vi "TCE.vi"() -> (11 "placeholder image":T1(plugin-control))   [LabVIEW 2024]
uses:
  DataCluster_TCAL.ctl
  <vilib>/vision/Image Controls.llb/IMAQ Image.ctl
  TCE_Config.ctl
  <vilib>/Utility/file.llb/Read Delimited Spreadsheet (string).vi
  <vilib>/Utility/file.llb/Write Delimited Spreadsheet (string).vi
  <vilib>/Utility/file.llb/Write Delimited Spreadsheet (DBL).vi
  <vilib>/Analysis/NI_AALBase.lvlib
panel:
  out "FreezeFract Concatinated":dbl[](array[numeric])
  in  "Correct Data":bool
  out "Offset Applied?":bool
  out "recentPaths":path[](array[path])=[path "D:/OneDrive/OneDrive - Aarhus Universitet/Data/D20_4/Result Data.csv"]
  out "version":string="version 0.0.0.1" caption="Version"
  out "Title":string="Thermal Camera Evaluation" caption="Version"
  in  "Remove_Correction":bool
  out "Offsets":dbl[](array[numeric])
  in  "Calc_All":bool
  in  "Well":i32=251
  in  "ImageIdx":u32(slide)=98 scale=0.0..527.0
  in  "Path":path
  out "MeltTemps":dbl[](array[numeric])=[-5.408275862068933, -5.766551724137912, -5.134827586206882, -4.684827586206836, -7.485172413793066, -5.2834482758620425, -5.345517241379298, -6.320689655172373, -3.992413793103424, -3.7082758620689447, -3.4782758620689265, -5.388275862068895, -5.597241379310333, -4.740689655172389, -4.031034482758571, -4.187241379310308, -6.245172413793114, -4.773793103448213, -4.427586206896535, -3.742413793103424, -4.568965517241338, -5.621379310344764, -4.7503448275861615, -5.029999999999973, -5.895517241379309, -4.551379310344771, -4.0196551724137635, -4.698965517241334, -4.126551724137926, -2.993448275862022, -4.383448275862065, -4.888965517241331, -5.901724137931012, -8.037586206896549, -3.918275862068924, -4.438620689655181, -5.749655172413782, -4.38241379310341, -4.932758620689583, -4.997586206896528, -4.125862068965489, -3.4279310344827536, -5.144482758620654, -2.891379310344803, -2.92999999999995, -3.1620689655172214, -3.216206896551739, -4.3248275862068795, -1.3320689655172373, -2.026551724137903, 0.5675862068965785, -0.5103448275861524, 0.4782758620689833, -1.9634482758620493, -0.1275862068965239, -0.1651724137930728, -0.9937931034482403, -0.6210344827586027, 0.2934482758620902, 0.6917241379310894, 1.3537931034483108, -1.852758620689599, -1.3782758620689037, 1.2606896551724844, -0.0275862068965012, -2.2548275862068294, -1.0710344827585914, -1.4565517241379098, -0.7220689655172237, -0.853793103448254, -0.2686206896551653, -0.5562068965517142, 0.0324137931034443, -0.2768965517241213, 1.1982758620689538, 1.2775862068966148, -0.6427586206896194, 0.5986206896552062, -0.3313793103448006, -0.6034482758620356, -2.0755172413792593, -2.182758620689583, -1.6548275862068635, -0.7234482758620402, -0.6872413793103078, -0.9086206896551516, -0.5427586206895967, -0.0527586206895876, 1.211379310344853, 0.2365517241379393, -0.526551724137903, -0.1537931034482085, 1.1865517241379848, 0.7089655172413813, -1.8837931034482267, 0.5872413793103988, -2.0686206896551766, -2.519310344827545, -2.2079310344827263, -2.2441379310344587, -2.0355172413792957, -2.3782758620689037, -2.0879310344827218, -1.998965517241345, -2.0948275862068613, -2.1227586206896376, -2.195517241379264, -1.969655172413752, -2.0175862068965102, -2.061724137931037, -2.028275862068938, -1.7403448275861706, -2.1765517241378802, -2.432758620689583, -2.186551724137928, -2.063448275862015, -2.331724137931019, -2.1351724137931, -2.0499999999999545, -2.1537931034482085, -2.235172413793066, -2.213793103448211, -2.082758620689617, -2.1703448275861774, -2.0434482758620334, -2.173448275862029, -1.9048275862068635, -1.683793103448238, -1.8931034482758378, -2.165172413793073, -2.068965517241338, -2.1862068965517096, -2.161034482758623, -2.085517241379307, -2.0631034482758537, -2.134137931034445, -2.104827586206852, -2.1775862068965353, -2.2255172413792934, -2.161724137931003, -2.0251724137930864, -2.0106896551724276, -2.211379310344796, -1.9093103448275315, -2.3158620689654867, -1.9827586206895944, -2.258275862068899, -2.2927586206895967, -2.0868965517241236, -2.0810344827585823, -2.17931034482757, -2.134137931034445, -2.151379310344794, -2.101034482758621, -2.2465517241379303, -2.339999999999975, -2.061379310344819, -2.082413793103399, -2.220689655172407, -2.0658620689654867, -2.1337931034482267, -2.0158620689654754, -2.1179310344827513, -2.1999999999999886, -2.130344827586157, -2.0489655172413563, -2.0534482758620243, -2.0851724137930887, -2.1079310344827036, -2.0241379310344882, -2.0693103448275565, -2.1348275862068817, -2.1431034482758378, -2.0268965517241213, -2.0317241379310076, -1.6172413793103146, -2.02103448275858, -2.331724137931019, -2.4068965517241168, -2.2337931034482494, -2.383103448275847, -2.1417241379310212, -2.1768965517240986, -2.2579310344827377, -2.1786206896551334, -2.032068965517226, -2.1162068965517165, -2.2706896551724185, -1.9220689655172123, -2.174482758620684, -2.11206896551721, -2.0858620689654686, -0.1458620689654708, -0.1541379310344837, -0.0103448275861524, -0.2106896551724162, -0.2299999999999613, -0.243448275862022, -0.2624137931034056, -0.2906896551724003, -0.3306896551724208, -0.3089655172413472, -0.2099999999999795, -0.276551724137903, -0.15896551724137, -0.0637931034482335, -0.2572413793103578, 0.1706896551724526, -0.0779310344827309, -0.0958620689654595, 0.0658620689655436, -0.1041379310344723, -0.4631034482758308, -0.1158620689654981, -0.1268965517240872, -0.3313793103448006, -0.2803448275861911, -0.1562068965517369, -0.06793103448274, -0.131379310344812, -0.0282758620689378, 0.0079310344827945, 0.0748275862069363, 0.2665517241379689, 0.0537931034482995, -0.2062068965516914, -0.1179310344827513, -0.3424137931033897, -0.0275862068965012, -0.2003448275861501, -0.1096551724137953, -0.0944827586206429, -0.4137931034482563, -0.5093103448275542, 0.0627586206896922, -0.1789655172413518, -0.0096551724137726, 0.0068965517241395, -0.0334482758620425, 0.2120689655172896, -0.1099999999999568, -0.2282758620689265, -0.1213793103447642, -0.1482758620689424, -0.2106896551724162, -0.0927586206896081, -0.1093103448275201, -0.076206896551696, -0.1593103448275315, -0.0886206896551585, -0.1924137931034124, -0.0558620689654958, -0.0313793103447892, -0.0799999999999841, -0.1262068965517074, 0.2117241379310713, -0.1141379310344632, -0.1796551724137885, -0.2003448275861501, -0.0327586206896058, 0.0655172413793252, -0.1886206896551812, -0.0327586206896058, -0.1424137931034011, -0.2406896551723889, -0.034827586206859, -0.1527586206896103, -0.1848275862068363, -0.0313793103447892, -0.0158620689654754, -0.0372413793103306, 0.2079310344827832, -0.2451724137931137, -0.6586206896551516, -0.0858620689654686, -0.2462068965517119, -0.2631034482758423, -0.0217241379310167, -0.2486206896551266, 0.0455172413793434, -0.2441379310344587, -0.1786206896551334, -0.230689655172398, -0.0131034482758423, -0.2613793103448074, -0.4093103448275315, -0.0124137931034056, 0.1572413793103919, 0.0, 0.0, 0.0, 1.7110344827586346, 1.5944827586206998, 1.9227586206896488, 0.1648275862069113, 1.3268965517241327, 0.0, 0.0, 0.0, 1.441379310344871, 0.8996551724138158, 2.017586206896567, 1.1068965517241622, 2.3413793103448484, 1.119655172413843, 1.9251724137931205, 1.484482758620743, 1.7410344827586641, 1.624137931034511, 1.9227586206896488, 1.88793103448279, 1.3758620689655459, -0.8037931034482426, 1.6562068965517938, 1.90758620689661, 2.0327586206896626, 1.5831034482758923, 2.1006896551724594, 2.216206896551796, 2.153448275862104, 1.9158620689655093, 2.1862068965517665, 1.9189655172414175, 2.0968965517241713, 1.4434482758620675, 1.914482758620693, 1.868620689655188, 1.9841379310345246, 2.0734482758621198, 1.9231034482759242, 1.7982758620689765, 1.852068965517276, 2.086551724137962, 2.055172413793173, 1.9510344827586437, 2.1220689655172578, 2.108620689655197, 2.3431034482758832, 0.0, 1.7272413793103851, 2.039655172413859, 1.9255172413793389, 2.2200000000000273, 1.5868965517241804, 1.914482758620693, 1.9610344827586343, 2.145517241379366, 1.9279310344828102, 1.8203448275862115, 2.199310344827609, 2.312413793103474, 2.407931034482772, 2.4206896551724526, 1.8224137931034647, 2.3637931034483017, 1.6882758620689629, 1.8193103448276133, 1.7324137931034898, 2.3037931034482995, 1.794137931034527, 2.011034482758646, 2.0013793103448734, 1.7558620689655413, 1.8893103448276065, 2.1520689655172873, 1.9962068965517685, 2.3103448275862206, 2.1217241379310963, 1.863103448275922, 1.9231034482759242, 1.5434482758620902, 1.6648275862069113, 1.8944827586207111, 1.63793103448279, 1.8379310344827786, 1.948620689655229, 2.157241379310392, 1.835517241379364, 1.950344827586207, 2.018275862069004, 1.9565517241379666, 1.7651724137931524, 2.068965517241395, 2.168275862068981]
  out "FreezeArray":bool[](array[boolean])=[TRUE, TRUE, TRUE, TRUE, TRUE, TRUE, TRUE, TRUE, TRUE, TRUE, TRUE, TRUE, TRUE, TRUE, TRUE, TRUE, TRUE, TRUE, TRUE, TRUE, TRUE, TRUE, TRUE, TRUE, TRUE, TRUE, TRUE, TRUE, TRUE, TRUE, TRUE, TRUE, TRUE, TRUE, TRUE, TRUE, TRUE, TRUE, TRUE, TRUE, TRUE, TRUE, TRUE, TRUE, TRUE, TRUE, TRUE, TRUE, TRUE, TRUE, TRUE, TRUE, TRUE, TRUE, TRUE, TRUE, TRUE, TRUE, TRUE, TRUE, TRUE, TRUE, TRUE, TRUE, TRUE, TRUE, TRUE, TRUE, TRUE, TRUE, TRUE, TRUE, TRUE, TRUE, TRUE, TRUE, TRUE, TRUE, TRUE, TRUE, TRUE, TRUE, TRUE, TRUE, TRUE, TRUE, TRUE, TRUE, TRUE, TRUE, TRUE, TRUE, TRUE, TRUE, TRUE, TRUE, TRUE, TRUE, TRUE, TRUE, TRUE, TRUE, TRUE, TRUE, TRUE, TRUE, TRUE, TRUE, TRUE, TRUE, TRUE, TRUE, TRUE, TRUE, TRUE, TRUE, TRUE, TRUE, TRUE, TRUE, TRUE, TRUE, TRUE, TRUE, TRUE, TRUE, TRUE, TRUE, TRUE, TRUE, TRUE, TRUE, TRUE, TRUE, TRUE, TRUE, TRUE, TRUE, TRUE, TRUE, TRUE, TRUE, TRUE, TRUE, TRUE, TRUE, TRUE, TRUE, TRUE, TRUE, TRUE, TRUE, TRUE, TRUE, TRUE, TRUE, TRUE, TRUE, TRUE, TRUE, TRUE, TRUE, TRUE, TRUE, TRUE, TRUE, TRUE, TRUE, TRUE, TRUE, TRUE, TRUE, TRUE, TRUE, TRUE, TRUE, TRUE, TRUE, TRUE, TRUE, TRUE, TRUE, TRUE, TRUE, TRUE, TRUE, TRUE, TRUE, TRUE, TRUE, TRUE, TRUE, TRUE, TRUE, TRUE, TRUE, TRUE, TRUE, TRUE, TRUE, TRUE, TRUE, TRUE, TRUE, TRUE, TRUE, TRUE, TRUE, TRUE, TRUE, TRUE, TRUE, TRUE, TRUE, TRUE, TRUE, TRUE, TRUE, TRUE, TRUE, TRUE, TRUE, TRUE, TRUE, TRUE, TRUE, TRUE, TRUE, TRUE, TRUE, TRUE, TRUE, TRUE, TRUE, TRUE, TRUE, TRUE, TRUE, TRUE, TRUE, TRUE, TRUE, TRUE, TRUE, TRUE, TRUE, TRUE, TRUE, TRUE, TRUE, TRUE, TRUE, TRUE, TRUE, TRUE, TRUE, TRUE, TRUE, TRUE, TRUE, TRUE, TRUE, TRUE, TRUE, TRUE, TRUE, TRUE, TRUE, TRUE, TRUE, TRUE, TRUE, TRUE, TRUE, TRUE, TRUE, TRUE, TRUE, TRUE, TRUE, TRUE, TRUE, TRUE, TRUE, TRUE, TRUE, TRUE, TRUE, FALSE, FALSE, FALSE, TRUE, TRUE, TRUE, TRUE, TRUE, FALSE, FALSE, FALSE, TRUE, TRUE, TRUE, TRUE, TRUE, TRUE, TRUE, TRUE, TRUE, TRUE, TRUE, TRUE, TRUE, TRUE, TRUE, TRUE, TRUE, TRUE, TRUE, TRUE, TRUE, TRUE, TRUE, TRUE, TRUE, TRUE, TRUE, TRUE, TRUE, TRUE, TRUE, TRUE, TRUE, TRUE, TRUE, TRUE, TRUE, TRUE, TRUE, FALSE, TRUE, TRUE, TRUE, TRUE, TRUE, TRUE, TRUE, TRUE, TRUE, TRUE, TRUE, TRUE, TRUE, TRUE, TRUE, TRUE, TRUE, TRUE, TRUE, TRUE, TRUE, TRUE, TRUE, TRUE, TRUE, TRUE, TRUE, TRUE, TRUE, TRUE, TRUE, TRUE, TRUE, TRUE, TRUE, TRUE, TRUE, TRUE, TRUE, TRUE, TRUE, TRUE, TRUE, TRUE, TRUE]
  out "ThermTemps":dbl[](array[numeric])
  out "PartitionArray":string[](array[string])=["A, MQ unfiltered", "A, MQ unfiltered", "A, MQ unfiltered", "A, MQ unfiltered", "A, MQ unfiltered", "A, MQ unfiltered", "A, MQ unfiltered", "A, MQ unfiltered", "A, MQ unfiltered", "A, MQ unfiltered", "A, MQ unfiltered", "A, MQ unfiltered", "A, MQ unfiltered", "A, MQ unfiltered", "A, MQ unfiltered", "A, MQ unfiltered", "A, MQ unfiltered", "A, MQ unfiltered", "A, MQ unfiltered", "A, MQ unfiltered", "A, MQ unfiltered", "A, MQ unfiltered", "A, MQ unfiltered", "A, MQ unfiltered", "A, MQ unfiltered", "A, MQ unfiltered", "A, MQ unfiltered", "A, MQ unfiltered", "A, MQ unfiltered", "A, MQ unfiltered", "A, MQ unfiltered", "A, MQ unfiltered", "A, MQ unfiltered", "A, MQ unfiltered", "A, MQ unfiltered", "A, MQ unfiltered", "A, MQ unfiltered", "A, MQ unfiltered", "A, MQ unfiltered", "A, MQ unfiltered", "A, MQ unfiltered", "A, MQ unfiltered", "A, MQ unfiltered", "A, MQ unfiltered", "A, MQ unfiltered", "A, MQ unfiltered", "A, MQ unfiltered", "A, MQ unfiltered", "B, D2O unfiltered", "B, D2O unfiltered", "B, D2O unfiltered", "B, D2O unfiltered", "B, D2O unfiltered", "B, D2O unfiltered", "B, D2O unfiltered", "B, D2O unfiltered", "B, D2O unfiltered", "B, D2O unfiltered", "B, D2O unfiltered", "B, D2O unfiltered", "B, D2O unfiltered", "B, D2O unfiltered", "B, D2O unfiltered", "B, D2O unfiltered", "B, D2O unfiltered", "B, D2O unfiltered", "B, D2O unfiltered", "B, D2O unfiltered", "B, D2O unfiltered", "B, D2O unfiltered", "B, D2O unfiltered", "B, D2O unfiltered", "B, D2O unfiltered", "B, D2O unfiltered", "B, D2O unfiltered", "B, D2O unfiltered", "B, D2O unfiltered", "B, D2O unfiltered", "B, D2O unfiltered", "B, D2O unfiltered", "B, D2O unfiltered", "B, D2O unfiltered", "B, D2O unfiltered", "B, D2O unfiltered", "B, D2O unfiltered", "B, D2O unfiltered", "B, D2O unfiltered", "B, D2O unfiltered", "B, D2O unfiltered", "B, D2O unfiltered", "B, D2O unfiltered", "B, D2O unfiltered", "B, D2O unfiltered", "B, D2O unfiltered", "B, D2O unfiltered", "B, D2O unfiltered", "C, 1mg/ml Snomax in MQ", "C, 1mg/ml Snomax in MQ", "C, 1mg/ml Snomax in MQ", "C, 1mg/ml Snomax in MQ", "C, 1mg/ml Snomax in MQ", "C, 1mg/ml Snomax in MQ", "C, 1mg/ml Snomax in MQ", "C, 1mg/ml Snomax in MQ", "C, 1mg/ml Snomax in MQ", "C, 1mg/ml Snomax in MQ", "C, 1mg/ml Snomax in MQ", "C, 1mg/ml Snomax in MQ", "C, 1mg/ml Snomax in MQ", "C, 1mg/ml Snomax in MQ", "C, 1mg/ml Snomax in MQ", "C, 1mg/ml Snomax in MQ", "C, 1mg/ml Snomax in MQ", "C, 1mg/ml Snomax in MQ", "C, 1mg/ml Snomax in MQ", "C, 1mg/ml Snomax in MQ", "C, 1mg/ml Snomax in MQ", "C, 1mg/ml Snomax in MQ", "C, 1mg/ml Snomax in MQ", "C, 1mg/ml Snomax in MQ", "C, 1mg/ml Snomax in MQ", "C, 1mg/ml Snomax in MQ", "C, 1mg/ml Snomax in MQ", "C, 1mg/ml Snomax in MQ", "C, 1mg/ml Snomax in MQ", "C, 1mg/ml Snomax in MQ", "C, 1mg/ml Snomax in MQ", "C, 1mg/ml Snomax in MQ", "C, 1mg/ml Snomax in MQ", "C, 1mg/ml Snomax in MQ", "C, 1mg/ml Snomax in MQ", "C, 1mg/ml Snomax in MQ", "C, 1mg/ml Snomax in MQ", "C, 1mg/ml Snomax in MQ", "C, 1mg/ml Snomax in MQ", "C, 1mg/ml Snomax in MQ", "C, 1mg/ml Snomax in MQ", "C, 1mg/ml Snomax in MQ", "C, 1mg/ml Snomax in MQ", "C, 1mg/ml Snomax in MQ", "C, 1mg/ml Snomax in MQ", "C, 1mg/ml Snomax in MQ", "C, 1mg/ml Snomax in MQ", "C, 1mg/ml Snomax in MQ", "C, 1mg/ml Snomax in MQ", "C, 1mg/ml Snomax in MQ", "C, 1mg/ml Snomax in MQ", "C, 1mg/ml Snomax in MQ", "C, 1mg/ml Snomax in MQ", "C, 1mg/ml Snomax in MQ", "C, 1mg/ml Snomax in MQ", "C, 1mg/ml Snomax in MQ", "C, 1mg/ml Snomax in MQ", "C, 1mg/ml Snomax in MQ", "C, 1mg/ml Snomax in MQ", "C, 1mg/ml Snomax in MQ", "C, 1mg/ml Snomax in MQ", "C, 1mg/ml Snomax in MQ", "C, 1mg/ml Snomax in MQ", "C, 1mg/ml Snomax in MQ", "C, 1mg/ml Snomax in MQ", "C, 1mg/ml Snomax in MQ", "C, 1mg/ml Snomax in MQ", "C, 1mg/ml Snomax in MQ", "C, 1mg/ml Snomax in MQ", "C, 1mg/ml Snomax in MQ", "C, 1mg/ml Snomax in MQ", "C, 1mg/ml Snomax in MQ", "C, 1mg/ml Snomax in MQ", "C, 1mg/ml Snomax in MQ", "C, 1mg/ml Snomax in MQ", "C, 1mg/ml Snomax in MQ", "C, 1mg/ml Snomax in MQ", "C, 1mg/ml Snomax in MQ", "C, 1mg/ml Snomax in MQ", "C, 1mg/ml Snomax in MQ", "C, 1mg/ml Snomax in MQ", "C, 1mg/ml Snomax in MQ", "C, 1mg/ml Snomax in MQ", "C, 1mg/ml Snomax in MQ", "C, 1mg/ml Snomax in MQ", "C, 1mg/ml Snomax in MQ", "C, 1mg/ml Snomax in MQ", "C, 1mg/ml Snomax in MQ", "C, 1mg/ml Snomax in MQ", "C, 1mg/ml Snomax in MQ", "C, 1mg/ml Snomax in MQ", "C, 1mg/ml Snomax in MQ", "C, 1mg/ml Snomax in MQ", "C, 1mg/ml Snomax in MQ", "C, 1mg/ml Snomax in MQ", "C, 1mg/ml Snomax in MQ", "D, 1mg/ml Snomax in 1:1 MQ:D2O", "D, 1mg/ml Snomax in 1:1 MQ:D2O", "D, 1mg/ml Snomax in 1:1 MQ:D2O", "D, 1mg/ml Snomax in 1:1 MQ:D2O", "D, 1mg/ml Snomax in 1:1 MQ:D2O", "D, 1mg/ml Snomax in 1:1 MQ:D2O", "D, 1mg/ml Snomax in 1:1 MQ:D2O", "D, 1mg/ml Snomax in 1:1 MQ:D2O", "D, 1mg/ml Snomax in 1:1 MQ:D2O", "D, 1mg/ml Snomax in 1:1 MQ:D2O", "D, 1mg/ml Snomax in 1:1 MQ:D2O", "D, 1mg/ml Snomax in 1:1 MQ:D2O", "D, 1mg/ml Snomax in 1:1 MQ:D2O", "D, 1mg/ml Snomax in 1:1 MQ:D2O", "D, 1mg/ml Snomax in 1:1 MQ:D2O", "D, 1mg/ml Snomax in 1:1 MQ:D2O", "D, 1mg/ml Snomax in 1:1 MQ:D2O", "D, 1mg/ml Snomax in 1:1 MQ:D2O", "D, 1mg/ml Snomax in 1:1 MQ:D2O", "D, 1mg/ml Snomax in 1:1 MQ:D2O", "D, 1mg/ml Snomax in 1:1 MQ:D2O", "D, 1mg/ml Snomax in 1:1 MQ:D2O", "D, 1mg/ml Snomax in 1:1 MQ:D2O", "D, 1mg/ml Snomax in 1:1 MQ:D2O", "D, 1mg/ml Snomax in 1:1 MQ:D2O", "D, 1mg/ml Snomax in 1:1 MQ:D2O", "D, 1mg/ml Snomax in 1:1 MQ:D2O", "D, 1mg/ml Snomax in 1:1 MQ:D2O", "D, 1mg/ml Snomax in 1:1 MQ:D2O", "D, 1mg/ml Snomax in 1:1 MQ:D2O", "D, 1mg/ml Snomax in 1:1 MQ:D2O", "D, 1mg/ml Snomax in 1:1 MQ:D2O", "D, 1mg/ml Snomax in 1:1 MQ:D2O", "D, 1mg/ml Snomax in 1:1 MQ:D2O", "D, 1mg/ml Snomax in 1:1 MQ:D2O", "D, 1mg/ml Snomax in 1:1 MQ:D2O", "D, 1mg/ml Snomax in 1:1 MQ:D2O", "D, 1mg/ml Snomax in 1:1 MQ:D2O", "D, 1mg/ml Snomax in 1:1 MQ:D2O", "D, 1mg/ml Snomax in 1:1 MQ:D2O", "D, 1mg/ml Snomax in 1:1 MQ:D2O", "D, 1mg/ml Snomax in 1:1 MQ:D2O", "D, 1mg/ml Snomax in 1:1 MQ:D2O", "D, 1mg/ml Snomax in 1:1 MQ:D2O", "D, 1mg/ml Snomax in 1:1 MQ:D2O", "D, 1mg/ml Snomax in 1:1 MQ:D2O", "D, 1mg/ml Snomax in 1:1 MQ:D2O", "D, 1mg/ml Snomax in 1:1 MQ:D2O", "D, 1mg/ml Snomax in 1:1 MQ:D2O", "D, 1mg/ml Snomax in 1:1 MQ:D2O", "D, 1mg/ml Snomax in 1:1 MQ:D2O", "D, 1mg/ml Snomax in 1:1 MQ:D2O", "D, 1mg/ml Snomax in 1:1 MQ:D2O", "D, 1mg/ml Snomax in 1:1 MQ:D2O", "D, 1mg/ml Snomax in 1:1 MQ:D2O", "D, 1mg/ml Snomax in 1:1 MQ:D2O", "D, 1mg/ml Snomax in 1:1 MQ:D2O", "D, 1mg/ml Snomax in 1:1 MQ:D2O", "D, 1mg/ml Snomax in 1:1 MQ:D2O", "D, 1mg/ml Snomax in 1:1 MQ:D2O", "D, 1mg/ml Snomax in 1:1 MQ:D2O", "D, 1mg/ml Snomax in 1:1 MQ:D2O", "D, 1mg/ml Snomax in 1:1 MQ:D2O", "D, 1mg/ml Snomax in 1:1 MQ:D2O", "D, 1mg/ml Snomax in 1:1 MQ:D2O", "D, 1mg/ml Snomax in 1:1 MQ:D2O", "D, 1mg/ml Snomax in 1:1 MQ:D2O", "D, 1mg/ml Snomax in 1:1 MQ:D2O", "D, 1mg/ml Snomax in 1:1 MQ:D2O", "D, 1mg/ml Snomax in 1:1 MQ:D2O", "D, 1mg/ml Snomax in 1:1 MQ:D2O", "D, 1mg/ml Snomax in 1:1 MQ:D2O", "D, 1mg/ml Snomax in 1:1 MQ:D2O", "D, 1mg/ml Snomax in 1:1 MQ:D2O", "D, 1mg/ml Snomax in 1:1 MQ:D2O", "D, 1mg/ml Snomax in 1:1 MQ:D2O", "D, 1mg/ml Snomax in 1:1 MQ:D2O", "D, 1mg/ml Snomax in 1:1 MQ:D2O", "D, 1mg/ml Snomax in 1:1 MQ:D2O", "D, 1mg/ml Snomax in 1:1 MQ:D2O", "D, 1mg/ml Snomax in 1:1 MQ:D2O", "D, 1mg/ml Snomax in 1:1 MQ:D2O", "D, 1mg/ml Snomax in 1:1 MQ:D2O", "D, 1mg/ml Snomax in 1:1 MQ:D2O", "D, 1mg/ml Snomax in 1:1 MQ:D2O", "D, 1mg/ml Snomax in 1:1 MQ:D2O", "D, 1mg/ml Snomax in 1:1 MQ:D2O", "D, 1mg/ml Snomax in 1:1 MQ:D2O", "D, 1mg/ml Snomax in 1:1 MQ:D2O", "D, 1mg/ml Snomax in 1:1 MQ:D2O", "D, 1mg/ml Snomax in 1:1 MQ:D2O", "D, 1mg/ml Snomax in 1:1 MQ:D2O", "D, 1mg/ml Snomax in 1:1 MQ:D2O", "D, 1mg/ml Snomax in 1:1 MQ:D2O", "D, 1mg/ml Snomax in 1:1 MQ:D2O", "D, 1mg/ml Snomax in 1:1 MQ:D2O", "E, 1mg/ml Snomax in D2O", "E, 1mg/ml Snomax in D2O", "E, 1mg/ml Snomax in D2O", "E, 1mg/ml Snomax in D2O", "E, 1mg/ml Snomax in D2O", "E, 1mg/ml Snomax in D2O", "E, 1mg/ml Snomax in D2O", "E, 1mg/ml Snomax in D2O", "E, 1mg/ml Snomax in D2O", "E, 1mg/ml Snomax in D2O", "E, 1mg/ml Snomax in D2O", "E, 1mg/ml Snomax in D2O", "E, 1mg/ml Snomax in D2O", "E, 1mg/ml Snomax in D2O", "E, 1mg/ml Snomax in D2O", "E, 1mg/ml Snomax in D2O", "E, 1mg/ml Snomax in D2O", "E, 1mg/ml Snomax in D2O", "E, 1mg/ml Snomax in D2O", "E, 1mg/ml Snomax in D2O", "E, 1mg/ml Snomax in D2O", "E, 1mg/ml Snomax in D2O", "E, 1mg/ml Snomax in D2O", "E, 1mg/ml Snomax in D2O", "E, 1mg/ml Snomax in D2O", "E, 1mg/ml Snomax in D2O", "E, 1mg/ml Snomax in D2O", "E, 1mg/ml Snomax in D2O", "E, 1mg/ml Snomax in D2O", "E, 1mg/ml Snomax in D2O", "E, 1mg/ml Snomax in D2O", "E, 1mg/ml Snomax in D2O", "E, 1mg/ml Snomax in D2O", "E, 1mg/ml Snomax in D2O", "E, 1mg/ml Snomax in D2O", "E, 1mg/ml Snomax in D2O", "E, 1mg/ml Snomax in D2O", "E, 1mg/ml Snomax in D2O", "E, 1mg/ml Snomax in D2O", "E, 1mg/ml Snomax in D2O", "E, 1mg/ml Snomax in D2O", "E, 1mg/ml Snomax in D2O", "E, 1mg/ml Snomax in D2O", "E, 1mg/ml Snomax in D2O", "E, 1mg/ml Snomax in D2O", "E, 1mg/ml Snomax in D2O", "E, 1mg/ml Snomax in D2O", "E, 1mg/ml Snomax in D2O", "E, 1mg/ml Snomax in D2O", "E, 1mg/ml Snomax in D2O", "E, 1mg/ml Snomax in D2O", "E, 1mg/ml Snomax in D2O", "E, 1mg/ml Snomax in D2O", "E, 1mg/ml Snomax in D2O", "E, 1mg/ml Snomax in D2O", "E, 1mg/ml Snomax in D2O", "E, 1mg/ml Snomax in D2O", "E, 1mg/ml Snomax in D2O", "E, 1mg/ml Snomax in D2O", "E, 1mg/ml Snomax in D2O", "E, 1mg/ml Snomax in D2O", "E, 1mg/ml Snomax in D2O", "E, 1mg/ml Snomax in D2O", "E, 1mg/ml Snomax in D2O", "E, 1mg/ml Snomax in D2O", "E, 1mg/ml Snomax in D2O", "E, 1mg/ml Snomax in D2O", "E, 1mg/ml Snomax in D2O", "E, 1mg/ml Snomax in D2O", "E, 1mg/ml Snomax in D2O", "E, 1mg/ml Snomax in D2O", "E, 1mg/ml Snomax in D2O", "E, 1mg/ml Snomax in D2O", "E, 1mg/ml Snomax in D2O", "E, 1mg/ml Snomax in D2O", "E, 1mg/ml Snomax in D2O", "E, 1mg/ml Snomax in D2O", "E, 1mg/ml Snomax in D2O", "E, 1mg/ml Snomax in D2O", "E, 1mg/ml Snomax in D2O", "E, 1mg/ml Snomax in D2O", "E, 1mg/ml Snomax in D2O", "E, 1mg/ml Snomax in D2O", "E, 1mg/ml Snomax in D2O", "E, 1mg/ml Snomax in D2O", "E, 1mg/ml Snomax in D2O", "E, 1mg/ml Snomax in D2O", "E, 1mg/ml Snomax in D2O", "E, 1mg/ml Snomax in D2O", "E, 1mg/ml Snomax in D2O", "E, 1mg/ml Snomax in D2O", "E, 1mg/ml Snomax in D2O", "E, 1mg/ml Snomax in D2O", "E, 1mg/ml Snomax in D2O", "E, 1mg/ml Snomax in D2O", "E, 1mg/ml Snomax in D2O"]
  out "FreezeTemps":dbl[](array[numeric])=[-17.102413793103437, -16.14275862068962, -19.01724137931032, -15.683103448275858, -25.12241379310342, -20.5310344827586, -21.968275862068907, -23.725862068965483, -16.464137931034486, -13.113793103448245, -11.636206896551698, -22.81517241379308, -23.049655172413765, -15.513103448275842, -18.779655172413783, -15.36448275862068, -23.218620689655154, -14.564137931034452, -14.352413793103437, -11.641724137931021, -17.657241379310335, -21.99793103448272, -23.813103448275854, -20.459310344827543, -22.592068965517228, -22.526206896551713, -16.890344827586148, -17.801724137931018, -17.235862068965474, -11.44310344827585, -16.035862068965457, -17.472413793103414, -17.914827586206854, -25.26724137931032, -15.10206896551722, -15.265862068965474, -22.079999999999984, -18.58586206896547, -20.5106896551724, -21.002758620689605, -21.88206896551722, -14.302068965517208, -23.049655172413765, -11.56448275862067, -9.727586206896547, -10.574482758620661, -10.471724137931005, -14.189999999999998, -18.853448275862036, -20.565517241379297, -14.187241379310308, -14.840344827586193, -14.906206896551737, -21.08172413793102, -19.829655172413766, -16.151379310344794, -20.792413793103407, -21.82482758620685, -14.474482758620638, -8.87551724137927, -5.148275862068942, -22.100689655172403, -21.813103448275854, -5.387931034482733, -13.19965517241377, -22.069655172413775, -20.66206896551722, -20.594137931034453, -19.319655172413775, -20.309999999999974, -16.707241379310346, -21.968275862068907, -18.70620689655172, -18.623448275862046, -6.637931034482733, -7.056206896551714, -22.052068965517208, -9.618275862068913, -16.901724137931012, -13.387241379310353, -20.70034482758618, -21.344137931034453, -21.40620689655171, -16.127241379310362, -20.572413793103408, -19.566206896551705, -19.49379310344824, -16.083448275862054, -5.782758620689606, -14.221034482758569, -19.863103448275837, -17.482068965517215, -5.9048275862068635, -8.006896551724083, -20.81793103448271, -11.433103448275858, -5.199999999999989, -5.525862068965466, -5.633448275862065, -5.417241379310326, -5.608965517241359, -5.6537931034482085, -5.74655172413793, -5.684482758620675, -5.691379310344814, -5.6758620689655, -5.808620689655129, -5.717586206896556, -5.676206896551719, -5.526896551724121, -5.435517241379273, -5.398620689655161, -5.285172413793077, -5.59172413793101, -5.664482758620636, -5.389999999999986, -5.610344827586175, -5.809999999999945, -5.582413793103399, -5.736896551724101, -5.824482758620661, -5.701379310344805, -5.67655172413788, -5.683103448275858, -5.648965517241322, -5.654482758620645, -5.394482758620654, -5.2789655172413745, -5.4324137931034215, -5.434482758620675, -5.513448275862061, -5.627931034482742, -5.778275862068938, -5.713103448275831, -5.601034482758621, -5.630689655172375, -5.699310344827552, -5.584482758620652, -5.70379310344822, -5.636896551724078, -5.628275862068904, -5.4948275862068385, -5.689310344827561, -5.402413793103392, -5.240689655172389, -5.448275862068897, -5.5555172413792775, -5.998965517241345, -5.548965517241356, -5.420689655172396, -5.645862068965471, -5.577931034482731, -5.6520689655172305, -5.590344827586193, -5.699999999999989, -5.640689655172423, -5.6299999999999955, -5.599310344827529, -5.45034482758615, -5.28793103448271, -5.263793103448222, -5.557931034482749, -5.471034482758569, -5.670344827586177, -5.626551724137926, -5.3606896551723935, -5.553448275862024, -5.736206896551721, -5.485517241379284, -5.536206896551732, -5.615862068965498, -5.4589655172413245, -5.904137931034484, -5.572413793103408, -5.5565517241379325, -5.072413793103408, -5.54482758620685, -5.425172413793064, -5.9865517241378825, -5.601724137931001, -5.816551724137923, -5.833448275862054, -5.495517241379275, -5.722068965517224, -5.5058620689654845, -5.552758620689588, -5.644137931034493, -5.5610344827586005, -5.523793103448213, -5.626551724137926, -5.5406896551724, -5.328275862068949, -2.799310344827518, -3.109999999999957, -3.088965517241377, -3.2558620689654845, -3.3810344827585936, -3.349310344827529, -3.327931034482731, -3.3241379310344428, -3.2679310344827286, -3.4796551724138, -3.1096551724137953, -3.299655172413793, -3.301379310344771, -3.1603448275861865, -2.941034482758596, -2.9506896551724253, -2.8889655172413313, -3.0858620689654686, -2.980689655172398, -3.146896551724126, -3.077931034482731, -3.2044827586206566, -3.164482758620636, -3.3927586206896194, -3.373103448275856, -3.2824137931033874, -3.2603448275861524, -3.264482758620659, -3.188275862068906, -3.086206896551687, -2.978965517241363, -2.9113793103447847, -2.8717241379310394, -3.0813793103448006, -3.0013793103448165, -2.8927586206896194, -3.1879310344827445, -3.2431034482758605, -3.254482758620668, -3.1889655172413427, -3.319655172413775, -3.3893103448275497, -3.1068965517241054, -2.8872413793103533, -2.9982758620689083, -3.2041379310344382, -3.2024137931034033, -2.812413793103417, -2.790344827586182, -3.00068965517238, -3.1693103448275224, -3.193103448275849, -3.195862068965482, -3.1141379310344632, -3.326896551724076, -3.2120689655172328, -3.224137931034477, -3.285862068965457, -3.215862068965464, -3.0582758620689106, -3.1924137931034124, -3.149655172413759, -3.17999999999995, -2.8662068965517165, -2.9058620689654617, -3.0134482758620607, -3.161724137931003, -3.131379310344812, -3.0813793103448006, -3.0351724137930773, -2.9986206896551266, -3.1968965517240804, -3.164482758620636, -3.0810344827585823, -3.220689655172407, -2.9931034482758605, -2.964137931034486, -3.17999999999995, -2.9920689655172055, -2.764827586206877, -2.886896551724078, -3.1758620689655004, -3.071724137931028, -3.196551724137919, -3.2237931034482585, -2.905172413793082, -3.262068965517244, -3.1627586206896012, -3.283793103448261, -3.164482758620636, -3.142413793103401, -3.1089655172413586, -3.034137931034479, -3.277586206896558, -3.0720689655172464, -2.629655172413777, 0.0, 0.0, 0.0, -0.7296551724137998, -1.1386206896551698, -1.0558620689654958, -1.305172413793116, -1.1862068965517096, 0.0, 0.0, 0.0, -1.1282758620689037, -1.1682758620689242, -0.5724137931034079, -1.1765517241378802, -0.2555172413792661, -1.0703448275861547, -0.7648275862068772, -1.057931034482749, -1.016551724137912, -0.9627586206896126, -1.0337931034482608, -0.9872413793103192, -1.2451724137931137, -1.3141379310344519, -1.0437931034482517, -1.0199999999999818, -0.95310344827584, -0.9817241379309962, -0.8799999999999955, -0.7527586206896331, -0.5689655172413381, -0.6779310344827536, -0.7651724137930955, -0.8879310344827331, -0.8582758620689219, -1.0286206896551562, -0.8986206896551607, -1.072413793103408, -0.8858620689654799, -0.9524137931034033, -0.9465517241379189, -0.9465517241379189, -0.6958620689654822, -0.9386206896551812, -0.6879310344827445, -0.8244827586206611, -0.540344827586182, -0.5341379310344792, -0.6255172413792707, 0.0, -0.8917241379310212, -0.8031034482758628, -0.7927586206895967, -0.3927586206896194, -1.0141379310344405, -0.7241379310344769, -0.8258620689654776, -0.8099999999999454, -0.7320689655172146, -0.8993103448275406, -0.6624137931034397, -0.5572413793103124, -0.355517241379289, 0.0244827586207066, -0.6931034482758491, -0.113103448275865, -0.8486206896551494, -0.581724137931019, -0.4658620689654641, -0.1306896551723753, -0.9151724137930728, -0.8689655172413495, -0.5741379310344428, -0.8624137931034284, -0.8899999999999864, -0.8365517241379052, -0.7541379310344496, -0.5631034482758537, -0.4710344827585686, -0.3586206896551403, -0.4551724137930933, -0.7186206896551539, -0.8586206896551403, -0.6134482758620265, -0.6841379310344564, -0.6020689655172191, -0.8358620689654686, -0.6906896551723776, -0.8324137931033988, -0.900689655172414, -0.5879310344827218, -0.8486206896551494, -0.6179310344827513, -0.4758620689654549, -0.4237931034482472]
  out "FreezeIdx":i32[](array[numeric])=[255, 242, 272, 236, 335, 287, 303, 320, 243, 209, 191, 311, 316, 234, 271, 238, 322, 225, 219, 192, 254, 301, 321, 283, 307, 309, 248, 257, 253, 193, 240, 259, 264, 335, 231, 232, 302, 265, 285, 291, 301, 219, 312, 192, 172, 182, 181, 221, 271, 285, 224, 228, 233, 290, 279, 240, 286, 296, 218, 162, 122, 305, 300, 128, 213, 302, 285, 284, 271, 280, 243, 297, 267, 262, 143, 147, 302, 170, 248, 214, 293, 293, 293, 240, 287, 272, 273, 236, 129, 217, 278, 252, 135, 153, 288, 192, 124, 131, 130, 125, 127, 127, 126, 129, 124, 127, 126, 126, 129, 126, 124, 128, 126, 126, 135, 125, 133, 136, 126, 131, 132, 131, 126, 125, 129, 132, 125, 128, 128, 127, 124, 126, 136, 130, 125, 129, 125, 134, 131, 126, 130, 125, 133, 128, 125, 130, 133, 137, 127, 124, 126, 124, 127, 126, 133, 130, 124, 133, 132, 124, 124, 129, 126, 128, 128, 123, 132, 131, 125, 127, 125, 124, 136, 126, 129, 126, 129, 126, 135, 126, 133, 130, 124, 126, 124, 124, 126, 123, 125, 125, 124, 129, 98, 100, 98, 105, 99, 102, 98, 100, 97, 104, 97, 98, 100, 99, 97, 99, 99, 105, 99, 106, 107, 99, 108, 104, 104, 100, 100, 98, 103, 98, 98, 99, 102, 106, 108, 96, 100, 108, 104, 99, 100, 108, 98, 97, 97, 99, 98, 98, 99, 99, 99, 110, 108, 100, 111, 100, 99, 107, 99, 98, 101, 99, 99, 99, 98, 98, 99, 99, 101, 107, 98, 99, 100, 98, 104, 98, 98, 99, 99, 98, 98, 99, 98, 100, 101, 100, 106, 101, 100, 99, 100, 99, 98, 102, 99, 98, 0, 0, 0, 71, 80, 75, 84, 81, 0, 0, 0, 74, 77, 72, 78, 75, 81, 73, 76, 80, 77, 76, 76, 82, 88, 77, 78, 79, 74, 74, 81, 78, 76, 75, 75, 77, 76, 82, 75, 74, 76, 83, 81, 72, 74, 73, 74, 74, 73, 79, 0, 79, 74, 75, 82, 76, 73, 80, 75, 73, 82, 73, 75, 79, 80, 77, 77, 74, 73, 73, 89, 77, 75, 71, 76, 76, 74, 74, 75, 73, 74, 71, 76, 78, 74, 74, 72, 75, 75, 75, 75, 73, 77, 73, 73, 75]
  out "maxSize":i32=527
  out "img":i32
  out "Slide":u8(slide) scale=0.0..100.0
  in  "Help":bool
  out "Tutorial":string="Load Image"
  out "Points":T2[](array[typedef])=[{"X"=62.0, "Y"=65.0}, {"X"=62.333332, "Y"=80.6}, {"X"=62.666668, "Y"=96.2}, {"X"=63.0, "Y"=111.8}, {"X"=63.333332, "Y"=127.4}, {"X"=63.666668, "Y"=143.0}, {"X"=64.0, "Y"=158.6}, {"X"=64.333336, "Y"=174.20001}, {"X"=64.666664, "Y"=189.8}, {"X"=65.0, "Y"=205.40001}, {"X"=65.333336, "Y"=221.0}, {"X"=65.666664, "Y"=236.6}, {"X"=66.0, "Y"=252.20001}, {"X"=66.333336, "Y"=267.8}, {"X"=66.666664, "Y"=283.40002}, {"X"=67.0, "Y"=299.0}, {"X"=77.565216, "Y"=64.695656}, {"X"=77.89855, "Y"=80.295654}, {"X"=78.23188, "Y"=95.89565}, {"X"=78.565216, "Y"=111.49565}, {"X"=78.89855, "Y"=127.09566}, {"X"=79.23188, "Y"=142.69565}, {"X"=79.565216, "Y"=158.29565}, {"X"=79.89855, "Y"=173.89566}, {"X"=80.23188, "Y"=189.49567}, {"X"=80.565216, "Y"=205.09566}, {"X"=80.89855, "Y"=220.69565}, {"X"=81.23188, "Y"=236.29565}, {"X"=81.565216, "Y"=251.89566}, {"X"=81.89855, "Y"=267.49567}, {"X"=82.23188, "Y"=283.09564}, {"X"=82.565216, "Y"=298.69565}, {"X"=93.13043, "Y"=64.391304}, {"X"=93.46377, "Y"=79.9913}, {"X"=93.797104, "Y"=95.59131}, {"X"=94.13043, "Y"=111.19131}, {"X"=94.46377, "Y"=126.791306}, {"X"=94.797104, "Y"=142.3913}, {"X"=95.13043, "Y"=157.9913}, {"X"=95.46377, "Y"=173.59131}, {"X"=95.797104, "Y"=189.19131}, {"X"=96.13043, "Y"=204.79132}, {"X"=96.46377, "Y"=220.39131}, {"X"=96.797104, "Y"=235.99132}, {"X"=97.13043, "Y"=251.59132}, {"X"=97.46377, "Y"=267.1913}, {"X"=97.797104, "Y"=282.79132}, {"X"=98.13043, "Y"=298.3913}, {"X"=108.69565, "Y"=64.08696}, {"X"=109.028984, "Y"=79.68696}, {"X"=109.36232, "Y"=95.28696}, {"X"=109.695656, "Y"=110.88696}, {"X"=110.028984, "Y"=126.48695}, {"X"=110.36232, "Y"=142.08696}, {"X"=110.695656, "Y"=157.68697}, {"X"=111.028984, "Y"=173.28696}, {"X"=111.36232, "Y"=188.88696}, {"X"=111.695656, "Y"=204.48697}, {"X"=112.028984, "Y"=220.08696}, {"X"=112.36232, "Y"=235.68697}, {"X"=112.695656, "Y"=251.28697}, {"X"=113.028984, "Y"=266.88696}, {"X"=113.36232, "Y"=282.48697}, {"X"=113.695656, "Y"=298.08698}, {"X"=124.260864, "Y"=63.782608}, {"X"=124.5942, "Y"=79.38261}, {"X"=124.927536, "Y"=94.982605}, {"X"=125.26087, "Y"=110.58261}, {"X"=125.5942, "Y"=126.18261}, {"X"=125.927536, "Y"=141.78261}, {"X"=126.26087, "Y"=157.38261}, {"X"=126.5942, "Y"=172.9826}, {"X"=126.927536, "Y"=188.58261}, {"X"=127.26087, "Y"=204.18262}, {"X"=127.5942, "Y"=219.78261}, {"X"=127.927536, "Y"=235.38261}, {"X"=128.26086, "Y"=250.98262}, {"X"=128.59421, "Y"=266.5826}, {"X"=128.92754, "Y"=282.18262}, {"X"=129.26086, "Y"=297.7826}, {"X"=139.82608, "Y"=63.47826}, {"X"=140.15942, "Y"=79.07826}, {"X"=140.49275, "Y"=94.67826}, {"X"=140.8261, "Y"=110.27826}, {"X"=141.15942, "Y"=125.878265}, {"X"=141.49275, "Y"=141.47827}, {"X"=141.8261, "Y"=157.07828}, {"X"=142.15942, "Y"=172.67827}, {"X"=142.49275, "Y"=188.27826}, {"X"=142.8261, "Y"=203.87827}, {"X"=143.15942, "Y"=219.47826}, {"X"=143.49275, "Y"=235.07826}, {"X"=143.8261, "Y"=250.67827}, {"X"=144.15942, "Y"=266.27826}, {"X"=144.49275, "Y"=281.87827}, {"X"=144.8261, "Y"=297.47827}, {"X"=155.3913, "Y"=63.173912}, {"X"=155.72464, "Y"=78.77391}, {"X"=156.05797, "Y"=94.37392}, {"X"=156.39131, "Y"=109.973915}, {"X"=156.72464, "Y"=125.57391}, {"X"=157.05797, "Y"=141.17392}, {"X"=157.39131, "Y"=156.77393}, {"X"=157.72464, "Y"=172.37392}, {"X"=158.05797, "Y"=187.9739}, {"X"=158.39131, "Y"=203.57393}, {"X"=158.72464, "Y"=219.17392}, {"X"=159.05797, "Y"=234.77393}, {"X"=159.39131, "Y"=250.37393}, {"X"=159.72464, "Y"=265.97394}, {"X"=160.05797, "Y"=281.5739}, {"X"=160.39131, "Y"=297.17392}, {"X"=170.95651, "Y"=62.869564}, {"X"=171.28986, "Y"=78.46957}, {"X"=171.62318, "Y"=94.069565}, {"X"=171.95653, "Y"=109.66957}, {"X"=172.28986, "Y"=125.26956}, {"X"=172.62318, "Y"=140.86957}, {"X"=172.95653, "Y"=156.46957}, {"X"=173.28986, "Y"=172.06958}, {"X"=173.62318, "Y"=187.66957}, {"X"=173.95653, "Y"=203.26958}, {"X"=174.28986, "Y"=218.86957}, {"X"=174.62318, "Y"=234.46957}, {"X"=174.95653, "Y"=250.06958}, {"X"=175.28986, "Y"=265.66956}, {"X"=175.62318, "Y"=281.2696}, {"X"=175.95653, "Y"=296.86957}, {"X"=186.52173, "Y"=62.565216}, {"X"=186.85507, "Y"=78.16522}, {"X"=187.1884, "Y"=93.76522}, {"X"=187.52174, "Y"=109.36522}, {"X"=187.85507, "Y"=124.96522}, {"X"=188.1884, "Y"=140.56522}, {"X"=188.52174, "Y"=156.16522}, {"X"=188.85507, "Y"=171.76523}, {"X"=189.1884, "Y"=187.36522}, {"X"=189.52174, "Y"=202.96523}, {"X"=189.85507, "Y"=218.56522}, {"X"=190.1884, "Y"=234.16522}, {"X"=190.52174, "Y"=249.76523}, {"X"=190.85507, "Y"=265.36523}, {"X"=191.1884, "Y"=280.9652}, {"X"=191.52174, "Y"=296.56522}, {"X"=202.08696, "Y"=62.260868}, {"X"=202.42029, "Y"=77.86087}, {"X"=202.75363, "Y"=93.46087}, {"X"=203.08696, "Y"=109.06087}, {"X"=203.42029, "Y"=124.66087}, {"X"=203.75363, "Y"=140.26086}, {"X"=204.08696, "Y"=155.86087}, {"X"=204.42029, "Y"=171.46088}, {"X"=204.75363, "Y"=187.06088}, {"X"=205.08696, "Y"=202.66087}, {"X"=205.42029, "Y"=218.26086}, {"X"=205.75363, "Y"=233.86087}, {"X"=206.08696, "Y"=249.46088}, {"X"=206.42029, "Y"=265.06085}, {"X"=206.75363, "Y"=280.6609}, {"X"=207.08696, "Y"=296.26086}, {"X"=217.65218, "Y"=61.95652}, {"X"=217.9855, "Y"=77.55652}, {"X"=218.31885, "Y"=93.156525}, {"X"=218.65218, "Y"=108.75652}, {"X"=218.9855, "Y"=124.35652}, {"X"=219.31885, "Y"=139.95651}, {"X"=219.65218, "Y"=155.55652}, {"X"=219.9855, "Y"=171.15652}, {"X"=220.31885, "Y"=186.75653}, {"X"=220.65218, "Y"=202.35654}, {"X"=220.9855, "Y"=217.95653}, {"X"=221.31885, "Y"=233.55653}, {"X"=221.65218, "Y"=249.15654}, {"X"=221.9855, "Y"=264.75653}, {"X"=222.31885, "Y"=280.35654}, {"X"=222.65218, "Y"=295.95654}, {"X"=233.21739, "Y"=61.652176}, {"X"=233.55072, "Y"=77.252174}, {"X"=233.88406, "Y"=92.85217}, {"X"=234.21739, "Y"=108.45218}, {"X"=234.55072, "Y"=124.05218}, {"X"=234.88406, "Y"=139.65218}, {"X"=235.21739, "Y"=155.25218}, {"X"=235.55072, "Y"=170.85217}, {"X"=235.88406, "Y"=186.45218}, {"X"=236.21739, "Y"=202.05219}, {"X"=236.55072, "Y"=217.65218}, {"X"=236.88406, "Y"=233.25218}, {"X"=237.21739, "Y"=248.85219}, {"X"=237.55072, "Y"=264.45218}, {"X"=237.88406, "Y"=280.0522}, {"X"=238.21739, "Y"=295.65216}, {"X"=248.78261, "Y"=61.347828}, {"X"=249.11594, "Y"=76.94783}, {"X"=249.44928, "Y"=92.54783}, {"X"=249.78261, "Y"=108.14783}, {"X"=250.11594, "Y"=123.74783}, {"X"=250.44928, "Y"=139.34782}, {"X"=250.78261, "Y"=154.94783}, {"X"=251.11594, "Y"=170.54782}, {"X"=251.44928, "Y"=186.14783}, {"X"=251.78261, "Y"=201.74783}, {"X"=252.11594, "Y"=217.34782}, {"X"=252.44928, "Y"=232.94783}, {"X"=252.78261, "Y"=248.54784}, {"X"=253.11594, "Y"=264.14783}, {"X"=253.44928, "Y"=279.74783}, {"X"=253.78261, "Y"=295.34784}, {"X"=264.34784, "Y"=61.04348}, {"X"=264.68115, "Y"=76.64348}, {"X"=265.0145, "Y"=92.24348}, {"X"=265.34784, "Y"=107.84348}, {"X"=265.68115, "Y"=123.44348}, {"X"=266.0145, "Y"=139.04349}, {"X"=266.34784, "Y"=154.6435}, {"X"=266.68115, "Y"=170.24348}, {"X"=267.0145, "Y"=185.84348}, {"X"=267.34784, "Y"=201.44348}, {"X"=267.68115, "Y"=217.04347}, {"X"=268.0145, "Y"=232.64348}, {"X"=268.34784, "Y"=248.24348}, {"X"=268.68115, "Y"=263.84348}, {"X"=269.0145, "Y"=279.44348}, {"X"=269.34784, "Y"=295.04346}, {"X"=279.91302, "Y"=60.739132}, {"X"=280.24637, "Y"=76.33913}, {"X"=280.5797, "Y"=91.93913}, {"X"=280.91306, "Y"=107.53914}, {"X"=281.24637, "Y"=123.13913}, {"X"=281.5797, "Y"=138.73914}, {"X"=281.91306, "Y"=154.33914}, {"X"=282.24637, "Y"=169.93913}, {"X"=282.5797, "Y"=185.53912}, {"X"=282.91306, "Y"=201.13914}, {"X"=283.24637, "Y"=216.73914}, {"X"=283.5797, "Y"=232.33914}, {"X"=283.91306, "Y"=247.93915}, {"X"=284.24637, "Y"=263.53912}, {"X"=284.5797, "Y"=279.13916}, {"X"=284.91306, "Y"=294.73914}, {"X"=295.47827, "Y"=60.434784}, {"X"=295.81158, "Y"=76.03478}, {"X"=296.14493, "Y"=91.63478}, {"X"=296.47827, "Y"=107.23479}, {"X"=296.81158, "Y"=122.834785}, {"X"=297.14493, "Y"=138.43478}, {"X"=297.47827, "Y"=154.03479}, {"X"=297.81158, "Y"=169.6348}, {"X"=298.14493, "Y"=185.23479}, {"X"=298.47827, "Y"=200.8348}, {"X"=298.81158, "Y"=216.43478}, {"X"=299.14493, "Y"=232.03479}, {"X"=299.47827, "Y"=247.6348}, {"X"=299.81158, "Y"=263.2348}, {"X"=300.14493, "Y"=278.83478}, {"X"=300.47827, "Y"=294.43478}, {"X"=311.04346, "Y"=60.130436}, {"X"=311.3768, "Y"=75.73044}, {"X"=311.71014, "Y"=91.33044}, {"X"=312.0435, "Y"=106.930435}, {"X"=312.3768, "Y"=122.53044}, {"X"=312.71014, "Y"=138.13043}, {"X"=313.0435, "Y"=153.73044}, {"X"=313.3768, "Y"=169.33044}, {"X"=313.71014, "Y"=184.93044}, {"X"=314.0435, "Y"=200.53044}, {"X"=314.3768, "Y"=216.13043}, {"X"=314.71014, "Y"=231.73044}, {"X"=315.0435, "Y"=247.33044}, {"X"=315.3768, "Y"=262.93042}, {"X"=315.71014, "Y"=278.53046}, {"X"=316.0435, "Y"=294.13043}, {"X"=326.6087, "Y"=59.826088}, {"X"=326.94205, "Y"=75.42609}, {"X"=327.27536, "Y"=91.02609}, {"X"=327.6087, "Y"=106.62609}, {"X"=327.94205, "Y"=122.22609}, {"X"=328.27536, "Y"=137.82608}, {"X"=328.6087, "Y"=153.42609}, {"X"=328.94205, "Y"=169.0261}, {"X"=329.27536, "Y"=184.6261}, {"X"=329.6087, "Y"=200.22609}, {"X"=329.94205, "Y"=215.82608}, {"X"=330.27536, "Y"=231.42609}, {"X"=330.6087, "Y"=247.0261}, {"X"=330.94205, "Y"=262.6261}, {"X"=331.27536, "Y"=278.22607}, {"X"=331.6087, "Y"=293.82608}, {"X"=342.17392, "Y"=59.52174}, {"X"=342.50726, "Y"=75.12174}, {"X"=342.84058, "Y"=90.72174}, {"X"=343.17392, "Y"=106.32175}, {"X"=343.50726, "Y"=121.92174}, {"X"=343.84058, "Y"=137.52173}, {"X"=344.17392, "Y"=153.12173}, {"X"=344.50726, "Y"=168.72174}, {"X"=344.84058, "Y"=184.32175}, {"X"=345.17392, "Y"=199.92175}, {"X"=345.50726, "Y"=215.52174}, {"X"=345.84058, "Y"=231.12175}, {"X"=346.17392, "Y"=246.72176}, {"X"=346.50726, "Y"=262.32175}, {"X"=346.84058, "Y"=277.92175}, {"X"=347.17392, "Y"=293.52173}, {"X"=357.73914, "Y"=59.217392}, {"X"=358.07248, "Y"=74.81739}, {"X"=358.4058, "Y"=90.41739}, {"X"=358.73914, "Y"=106.017395}, {"X"=359.07248, "Y"=121.61739}, {"X"=359.4058, "Y"=137.21739}, {"X"=359.73914, "Y"=152.8174}, {"X"=360.07248, "Y"=168.41739}, {"X"=360.4058, "Y"=184.0174}, {"X"=360.73914, "Y"=199.6174}, {"X"=361.07248, "Y"=215.21739}, {"X"=361.4058, "Y"=230.8174}, {"X"=361.73914, "Y"=246.4174}, {"X"=362.07248, "Y"=262.0174}, {"X"=362.4058, "Y"=277.6174}, {"X"=362.73914, "Y"=293.2174}, {"X"=373.30435, "Y"=58.913044}, {"X"=373.6377, "Y"=74.51305}, {"X"=373.971, "Y"=90.113045}, {"X"=374.30435, "Y"=105.71304}, {"X"=374.6377, "Y"=121.31305}, {"X"=374.971, "Y"=136.91304}, {"X"=375.30435, "Y"=152.51305}, {"X"=375.6377, "Y"=168.11305}, {"X"=375.971, "Y"=183.71304}, {"X"=376.30435, "Y"=199.31305}, {"X"=376.6377, "Y"=214.91304}, {"X"=376.971, "Y"=230.51305}, {"X"=377.30435, "Y"=246.11305}, {"X"=377.6377, "Y"=261.71304}, {"X"=377.971, "Y"=277.31305}, {"X"=378.30435, "Y"=292.91302}, {"X"=388.86957, "Y"=58.608696}, {"X"=389.2029, "Y"=74.208694}, {"X"=389.53622, "Y"=89.8087}, {"X"=389.86957, "Y"=105.4087}, {"X"=390.2029, "Y"=121.0087}, {"X"=390.53622, "Y"=136.6087}, {"X"=390.86957, "Y"=152.20871}, {"X"=391.2029, "Y"=167.8087}, {"X"=391.53622, "Y"=183.40869}, {"X"=391.86957, "Y"=199.0087}, {"X"=392.2029, "Y"=214.6087}, {"X"=392.53622, "Y"=230.20871}, {"X"=392.86957, "Y"=245.80872}, {"X"=393.2029, "Y"=261.4087}, {"X"=393.53622, "Y"=277.0087}, {"X"=393.86957, "Y"=292.6087}, {"X"=404.43478, "Y"=58.304348}, {"X"=404.76813, "Y"=73.90435}, {"X"=405.10144, "Y"=89.50435}, {"X"=405.43478, "Y"=105.104355}, {"X"=405.76813, "Y"=120.704346}, {"X"=406.10144, "Y"=136.30435}, {"X"=406.43478, "Y"=151.90436}, {"X"=406.76813, "Y"=167.50435}, {"X"=407.10144, "Y"=183.10435}, {"X"=407.43478, "Y"=198.70436}, {"X"=407.76813, "Y"=214.30435}, {"X"=408.10144, "Y"=229.90436}, {"X"=408.43478, "Y"=245.50436}, {"X"=408.76813, "Y"=261.10437}, {"X"=409.10144, "Y"=276.70435}, {"X"=409.43478, "Y"=292.30435}, {"X"=420.0, "Y"=58.0}, {"X"=420.33334, "Y"=73.6}, {"X"=420.66666, "Y"=89.2}, {"X"=421.0, "Y"=104.8}, {"X"=421.33334, "Y"=120.4}, {"X"=421.66666, "Y"=136.0}, {"X"=422.0, "Y"=151.6}, {"X"=422.33334, "Y"=167.20001}, {"X"=422.66666, "Y"=182.8}, {"X"=423.0, "Y"=198.40001}, {"X"=423.33334, "Y"=214.0}, {"X"=423.66666, "Y"=229.6}, {"X"=424.0, "Y"=245.20001}, {"X"=424.33334, "Y"=260.8}, {"X"=424.66666, "Y"=276.40002}, {"X"=425.0, "Y"=292.0}] {"Y" format="%.2f"; "X" format="%.2f"}
  out "Image":T1(plugin-control)
  out "MeltTemp":dbl=-0.0558620689654958 caption="Melt temp" format="%.3g °C"
  out "FreezeTemp":dbl=-3.0582758620689106 caption="Froze at" format="%.3g °C"
  out "Title 2":string="Well Data" caption="Version"
  out "Well":string="L16"
  out "CurTemp":dbl=-0.9882758620689174 caption="Temp" format="%.3g °C"
  out "Contents":string="D, 1mg/ml Snomax in 1:1 MQ:D2O"
  out "Temps":dbl[][](graph)
  out "Temps single":dbl[](graph)
  out "Fraction Single":dbl[](graph)=[0.0, 0.0, 0.0, 0.0, 0.0, 0.0, 0.0, 0.0, 0.0, 0.0, 0.0, 0.0, 0.0, 0.0, 0.0, 0.0, 0.0, 0.0, 0.0, 0.0, 0.0, 0.0, 0.0, 0.0, 0.0, 0.0, 0.0, 0.0, 0.0, 0.0, 0.0, 0.0, 0.0, 0.0, 0.0, 0.0, 0.0, 0.0, 0.0, 0.0, 0.0, 0.0, 0.0, 0.0, 0.0, 0.0, 0.0, 0.0, 0.0, 0.0, 0.0, 0.0, 0.0, 0.0, 0.0, 0.0, 0.0, 0.0, 0.0, 0.0, 0.0, 0.0, 0.0, 0.0, 0.0, 0.0, 0.0, 0.0, 0.0, 0.0, 0.0, 0.0, 0.0, 0.0, 0.0, 0.0, 0.0, 0.0, 0.0, 0.0, 0.0, 0.0, 0.0, 0.0, 0.0, 0.0, 0.0, 0.0, 0.0, 0.0, 0.0, 0.0, 0.0, 0.0, 0.0, 0.0, 0.0, 0.05263157894736842, 0.28421052631578947, 0.5578947368421052, 0.7052631578947368, 0.7473684210526316, 0.7789473684210526, 0.7894736842105263, 0.8421052631578947, 0.8631578947368421, 0.8947368421052632, 0.9263157894736842, 0.9789473684210527, 0.9789473684210527, 0.9894736842105263, 1.0, 1.0, 1.0, 1.0, 1.0, 1.0, 1.0, 1.0, 1.0, 1.0, 1.0, 1.0, 1.0, 1.0, 1.0, 1.0, 1.0, 1.0, 1.0, 1.0, 1.0, 1.0, 1.0, 1.0, 1.0, 1.0, 1.0, 1.0, 1.0, 1.0, 1.0, 1.0, 1.0, 1.0, 1.0, 1.0, 1.0, 1.0, 1.0, 1.0, 1.0, 1.0, 1.0, 1.0, 1.0, 1.0, 1.0, 1.0, 1.0, 1.0, 1.0, 1.0, 1.0, 1.0, 1.0, 1.0, 1.0, 1.0, 1.0, 1.0, 1.0, 1.0, 1.0, 1.0, 1.0, 1.0, 1.0, 1.0, 1.0, 1.0, 1.0, 1.0, 1.0, 1.0, 1.0, 1.0, 1.0, 1.0, 1.0, 1.0, 1.0, 1.0, 1.0, 1.0, 1.0, 1.0, 1.0, 1.0, 1.0, 1.0, 1.0, 1.0, 1.0, 1.0, 1.0, 1.0, 1.0, 1.0, 1.0, 1.0, 1.0, 1.0, 1.0, 1.0, 1.0, 1.0, 1.0, 1.0, 1.0, 1.0, 1.0, 1.0, 1.0, 1.0, 1.0, 1.0, 1.0, 1.0, 1.0, 1.0, 1.0, 1.0, 1.0, 1.0, 1.0, 1.0, 1.0, 1.0, 1.0, 1.0, 1.0, 1.0, 1.0, 1.0, 1.0, 1.0, 1.0, 1.0, 1.0, 1.0, 1.0, 1.0, 1.0, 1.0, 1.0, 1.0, 1.0, 1.0, 1.0, 1.0, 1.0, 1.0, 1.0, 1.0, 1.0, 1.0, 1.0, 1.0, 1.0, 1.0, 1.0, 1.0, 1.0, 1.0, 1.0, 1.0, 1.0, 1.0, 1.0, 1.0, 1.0, 1.0, 1.0, 1.0, 1.0, 1.0, 1.0, 1.0, 1.0, 1.0, 1.0, 1.0, 1.0, 1.0, 1.0, 1.0, 1.0, 1.0, 1.0, 1.0, 1.0, 1.0, 1.0, 1.0, 1.0, 1.0, 1.0, 1.0, 1.0, 1.0, 1.0, 1.0, 1.0, 1.0, 1.0, 1.0, 1.0, 1.0, 1.0, 1.0, 1.0, 1.0, 1.0, 1.0, 1.0, 1.0, 1.0, 1.0, 1.0, 1.0, 1.0, 1.0, 1.0, 1.0, 1.0, 1.0, 1.0, 1.0, 1.0, 1.0, 1.0, 1.0, 1.0, 1.0, 1.0, 1.0, 1.0, 1.0, 1.0, 1.0, 1.0, 1.0, 1.0, 1.0, 1.0, 1.0, 1.0, 1.0, 1.0, 1.0, 1.0, 1.0, 1.0, 1.0, 1.0, 1.0, 1.0, 1.0, 1.0, 1.0, 1.0, 1.0, 1.0, 1.0, 1.0, 1.0, 1.0, 1.0, 1.0, 1.0, 1.0, 1.0, 1.0, 1.0, 1.0, 1.0, 1.0, 1.0, 1.0, 1.0, 1.0, 1.0, 1.0, 1.0, 1.0, 1.0, 1.0, 1.0, 1.0, 1.0, 1.0, 1.0, 1.0, 1.0, 1.0, 1.0, 1.0, 1.0, 1.0, 1.0, 1.0, 1.0, 1.0, 1.0, 1.0, 1.0, 1.0, 1.0, 1.0, 1.0, 1.0, 1.0, 1.0, 1.0, 1.0, 1.0, 1.0, 1.0, 1.0, 1.0, 1.0, 1.0, 1.0, 1.0, 1.0, 1.0, 1.0, 1.0, 1.0, 1.0, 1.0, 1.0, 1.0, 1.0, 1.0, 1.0, 1.0, 1.0, 1.0, 1.0, 1.0, 1.0, 1.0, 1.0, 1.0, 1.0, 1.0, 1.0, 1.0, 1.0, 1.0, 1.0, 1.0, 1.0, 1.0, 1.0, 1.0, 1.0, 1.0, 1.0, 1.0, 1.0, 1.0, 1.0, 1.0, 1.0, 1.0, 1.0, 1.0, 1.0, 1.0, 1.0, 1.0, 1.0, 1.0, 1.0, 1.0, 1.0, 1.0, 1.0, 1.0, 1.0, 1.0, 1.0, 1.0, 1.0, 1.0, 1.0, 1.0, 1.0, 1.0, 1.0, 1.0, 1.0, 1.0, 1.0, 1.0, 1.0, 1.0, 1.0, 1.0, 1.0, 1.0, 1.0, 1.0, 1.0, 1.0, 1.0, 1.0, 1.0, 1.0, 1.0, 1.0, 1.0, 1.0, 1.0, 1.0]
  out "FrozenFractionGraph":dbl[][](graph)
  out "Temps single grad":dbl[](graph)
  out "Temps grads":dbl[][](graph)
  # "hints: \nUse the Mouse Wheel to zoom in and out"
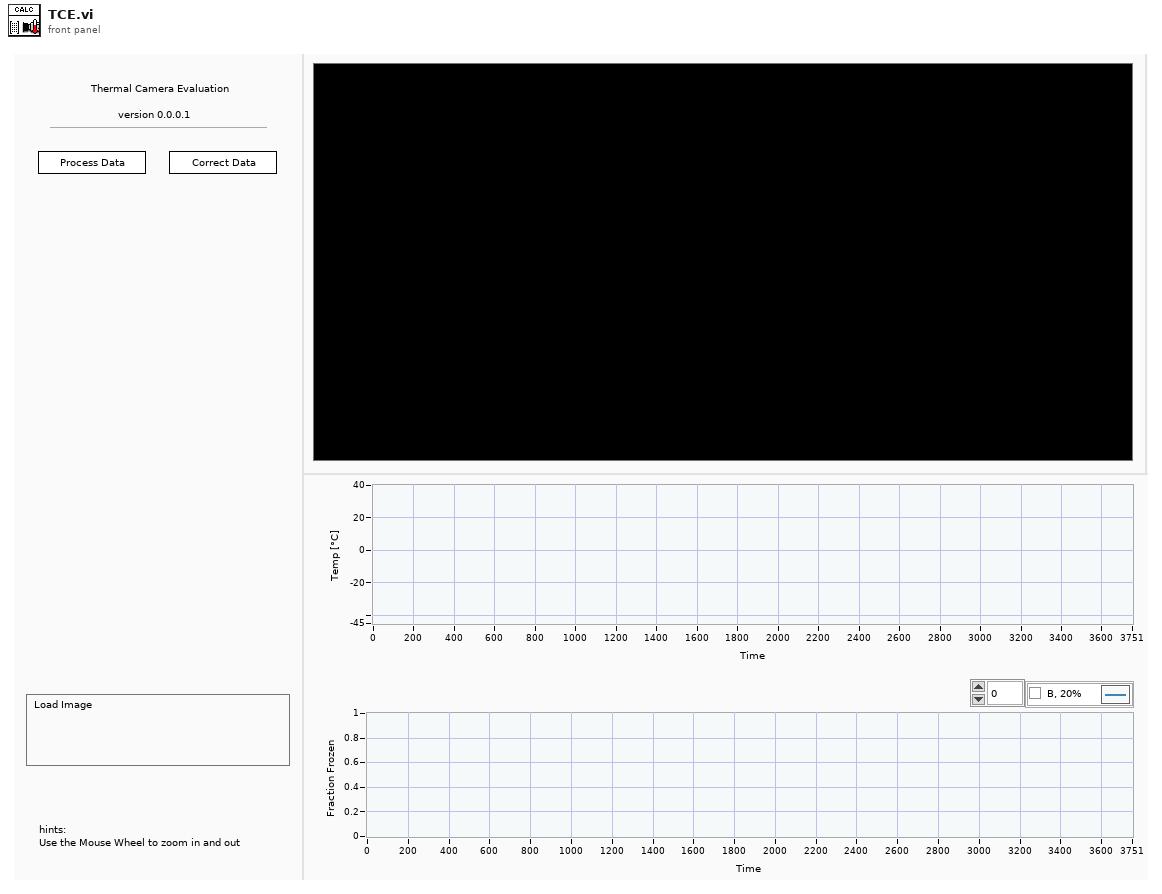
[diagram p1: front panel]
types:
  T1 = typedef "IMAQ Image.ctl" = refnum<image>
  T2 = typedef "IMAQ Point" = cluster{"X":sgl, "Y":sgl}
  T3 = typedef "TCE_Config.ctl" = cluster{"Freezing":cluster{"Cutoff":dbl, "EndIndex":i32}}
  T4 = typedef "DataCluster_TCAL.ctl" = cluster{"Core":cluster{"Current VI Reference":refnum<vi>, "Close Panel on Exit?":bool}, "Image Out":T1, "State":i32, "Points":cluster{"Top Left":T2, "Top Right":T2, "Bottom Left":T2, "Bottom Right":T2, "x space 2":dbl, "y space 2":sgl, "x_space":sgl, "y_space":sgl, "Pixels":cluster{"X":i32, "Y":i32}[][], "Fixpoint":T2}, "img_array":T1[], "Temps":dbl[], "Temps_Array":dbl[][], "Scan Area":dbl, "Fixpoint Area":dbl, "Config":T3, "PCR Size":u16, "ImageCount":i32, "ShowGradient":bool, "Save Well data":bool, "Save Blackbody data":bool, "Save Temps For Offset":bool}
  T5 = enum32{"Invalid", "Standard", "Closed", "Hidden", "Minimized", "Maximized"}
  T6 = enum32{"invalid app kind", "Development System", "Run Time System", "Student Edition", "Embedded LabVIEW", "Evaluation", "Custom"}
  T7 = cluster{"Global Rectangle":i32[], "Contours":cluster{"Contour Type":u32, "ROI Type":u32, "Points":i32[]}[]}
  T8 = enum8{"Enabled", "Disabled", "Disabled and Grayed Out"}
  T9 = enum16{"Ignore", "All Wells Mean", "Pixel Values Wells"}
  T10 = cluster{"Desired Font (Application)":enum16{"User-specified Font", "Application Font", "System Font", "Dialog Font"}, "[User-specified Font]":cluster{"Font Name":string, "Size":i16, "Strikeout?":bool, "Italic?":bool, "Underline?":bool, "Outline?":bool, "Shadow?":bool, "Bold?":bool, "Rotation Angle":dbl}, "Horizontal Alignment":i16, "Vertical Alignment":i16}
  T11 = typedef "ROI Descriptor" = cluster{"Global Rectangle":i32[], "Contours":cluster{"ID":enum32{"External", "Internal"}, "Type":u32, "Coordinates":i32[]}[]}
  T12 = cluster{"Current VI Reference":refnum<vi>, "Close Panel on Exit?":bool}
  T13 = typedef "Image Type" = u32
  T14 = cluster{"Top Left":T2, "Top Right":T2, "Bottom Left":T2, "Bottom Right":T2, "x space 2":dbl, "y space 2":sgl, "x_space":sgl, "y_space":sgl, "Pixels":cluster{"X":i32, "Y":i32}[][], "Fixpoint":T2}
  T15 = cluster{"Mean of Pixels from Well x1":dbl, "Pixel for well x1 each picture":dbl[], "Mean of Pixels from Well x2":dbl, "Pixel for well x2 each picture":dbl[], "Mean of Pixels from Well x3":dbl, "Pixel for well x3 each picture":dbl[], "Mean of Pixels from Well x4":dbl, "Pixel for well x4 each picture":dbl[], "Pixel Number":i32}
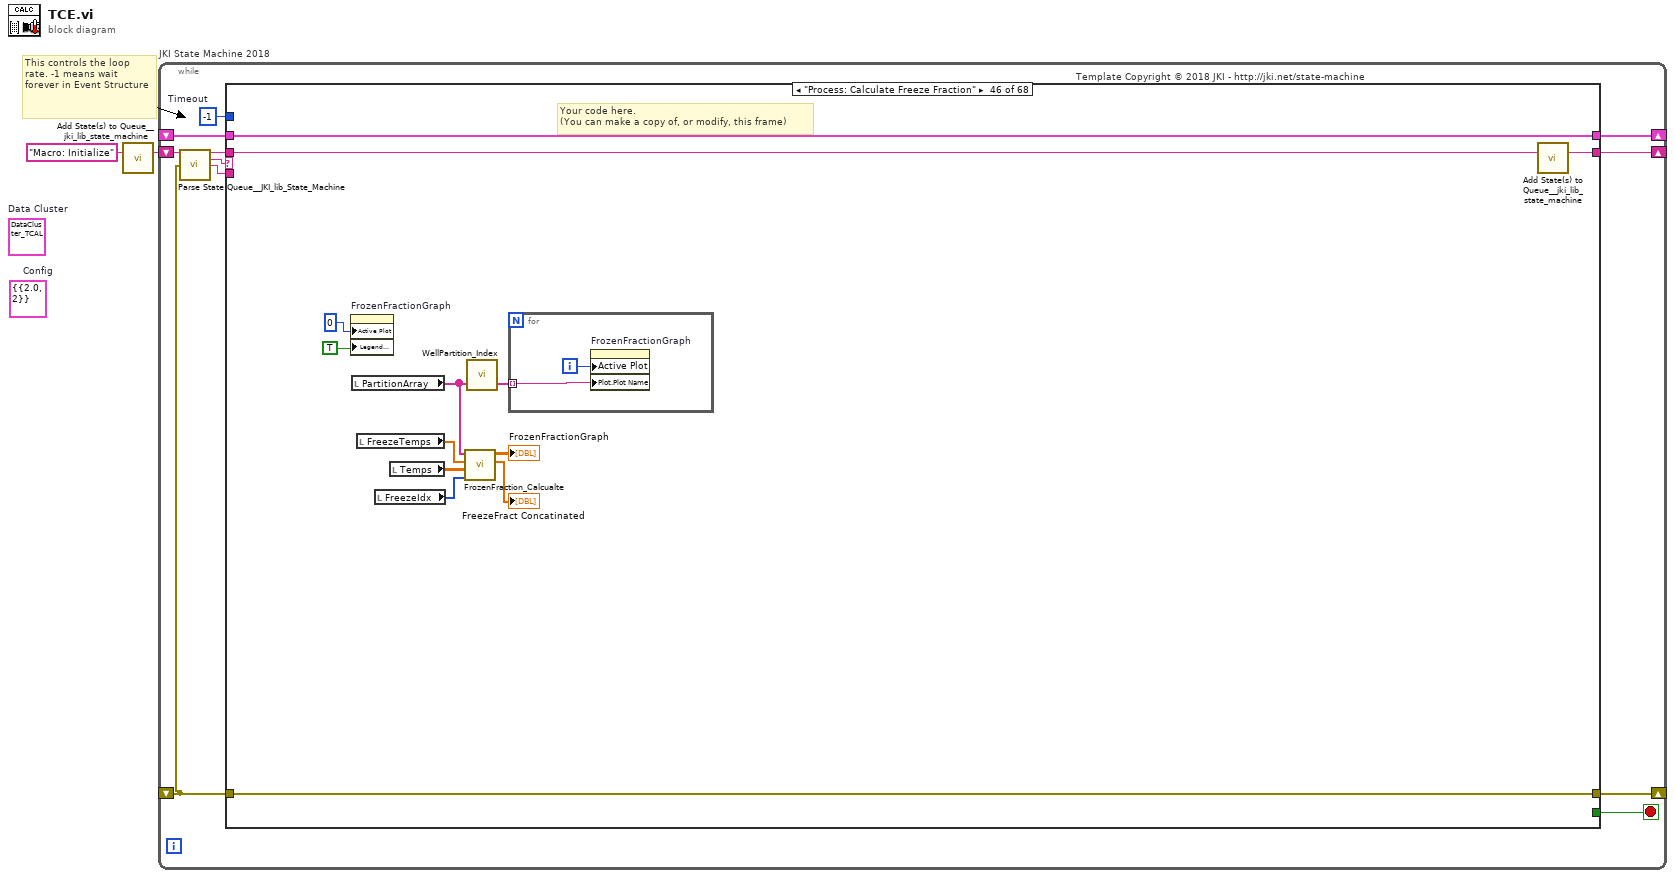
[diagram p0: block diagram]
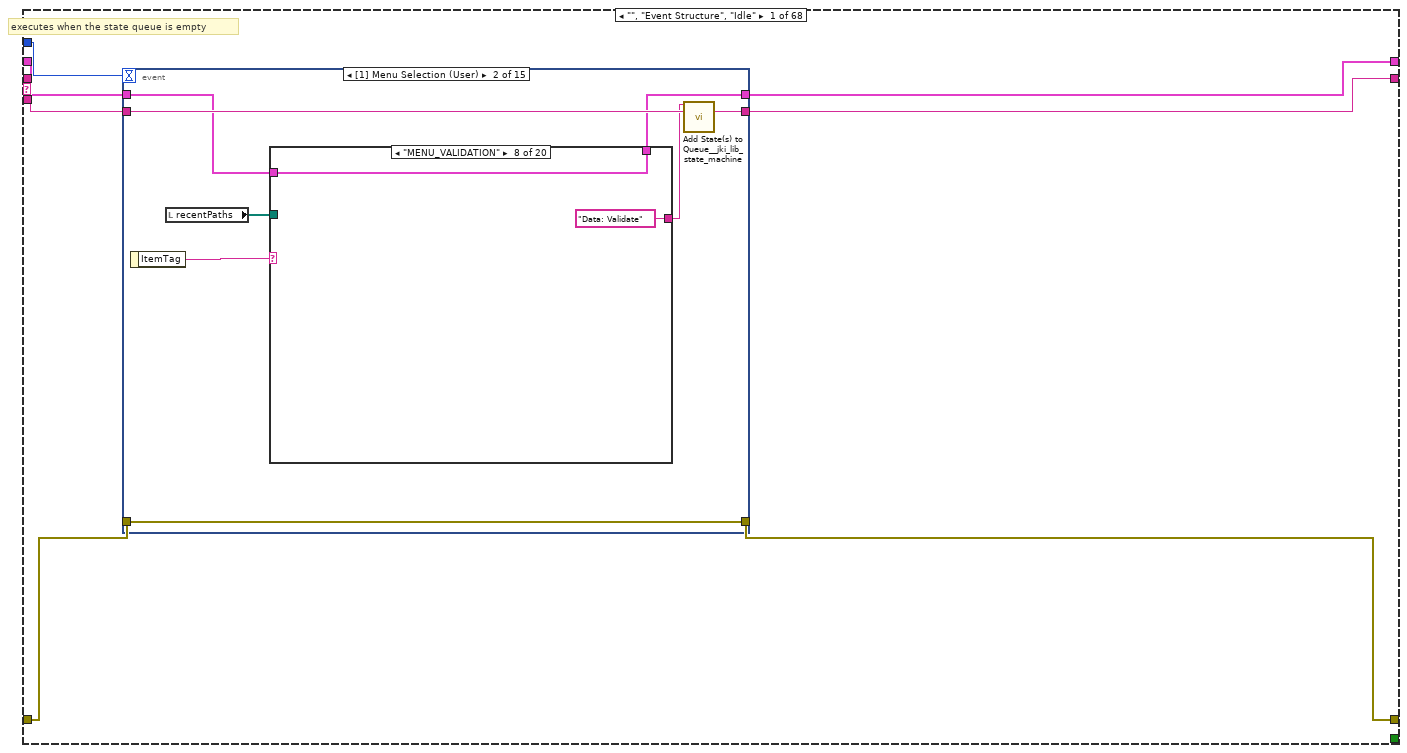
[diagram p2: hidden frame]
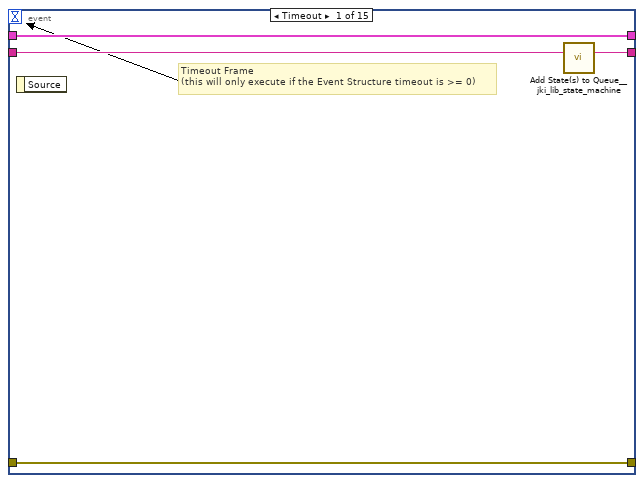
[diagram p3: hidden frame]
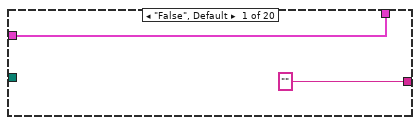
[diagram p4: hidden frame]
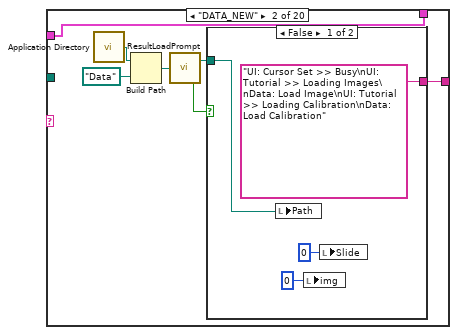
[diagram p5: hidden frame]
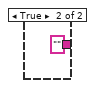
[diagram p6: hidden frame]
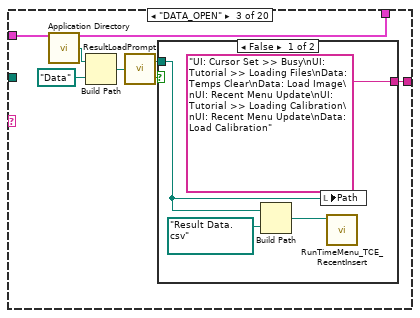
[diagram p7: hidden frame]
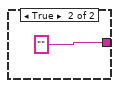
[diagram p8: hidden frame]
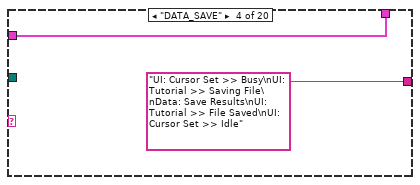
[diagram p9: hidden frame]
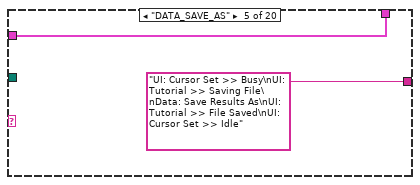
[diagram p10: hidden frame]
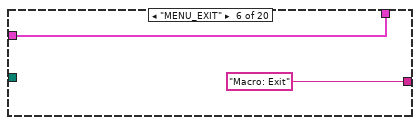
[diagram p11: hidden frame]
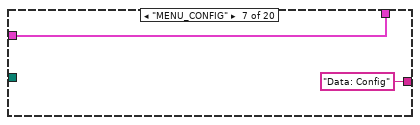
[diagram p12: hidden frame]
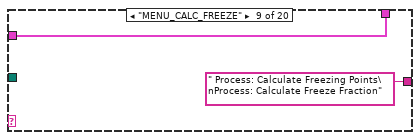
[diagram p13: hidden frame]
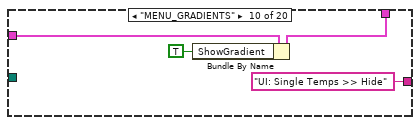
[diagram p14: hidden frame]
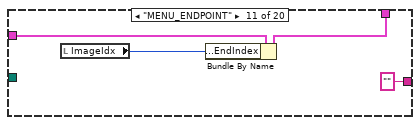
[diagram p15: hidden frame]
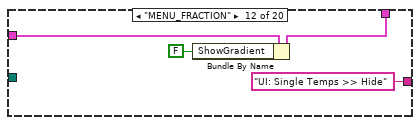
[diagram p16: hidden frame]
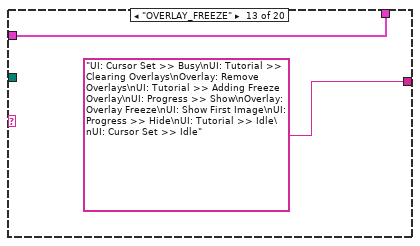
[diagram p17: hidden frame]
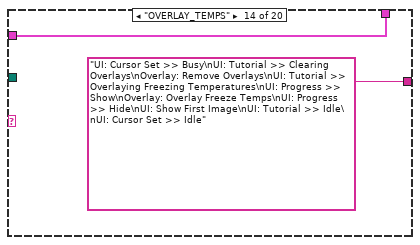
[diagram p18: hidden frame]
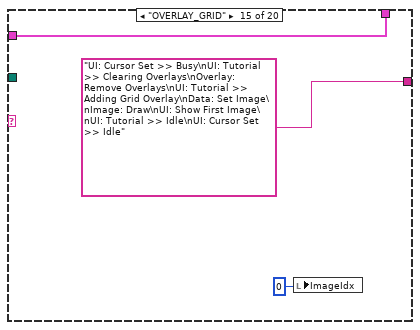
[diagram p19: hidden frame]
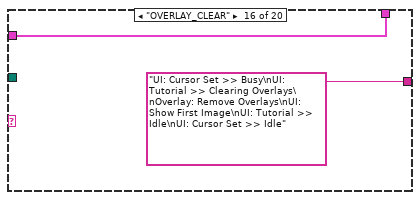
[diagram p20: hidden frame]
diagram:
  (unwired) T3 {"Freezing"={"Cutoff"=2.0, "EndIndex"=2}}  # Config
  (unwired) T4 {"Core"={"Current VI Reference"=refnum, "Close Panel on Exit?"=FALSE}, "Image Out"=refnum, "State"=0, "Points"={"Top Left"={"X"=0.0, "Y"=0.0}, "Top Right"={"X"=0.0, "Y"=0.0}, "Bottom Left"={"X"=0.0, "Y"=0.0}, "Bottom Right"={"X"=0.0, "Y"=0.0}, "x space 2"=0.0, "y space 2"=0.0, "x_space"=0.0, "y_space"=0.0, "Pixels"=[], "Fixpoint"={"X"=0.0, "Y"=0.0}}, "img_array"=[], "Temps"=[], "Temps_Array"=[], "Scan Area"=0.0, "Fixpoint Area"=0.0, "Config"={"Freezing"={"Cutoff"=2.0, "EndIndex"=2}}, "PCR Size"=0, "ImageCount"=0, "ShowGradient"=FALSE, "Save Well data"=FALSE, "Save Blackbody data"=FALSE, "Save Temps For Offset"=FALSE}  # Data Cluster
  # "This controls the loop rate. -1 means wait forever in Event Structure"
  n1 = call <vilib>:"Add State(s) to Queue__jki_lib_state_machine.vi"("State(s) in (\"\")"="Macro: Initialize") -> ("States Out"=w2:string)  [unwired: 14 in]
  n2 = while "JKI State Machine 2018" {
    shift-right: [w6] -> _
    shift-left: _ -> [w5]
    shift-right: [w9] -> _
    shift-left: _ -> [w3]
    shift-right: [w8] -> _
    shift-left: w2 -> [w10]
    stop <- w7 stop-if-true
    w4 = -1  # Timeout
    # "Template Copyright © 2018 JKI - http://jki.net/state-machine"
    n3 = call <vilib>:"Parse State Queue__JKI_lib_State_Machine.vi"("State Queue"=w10, "Error In (no error)"=w3) -> ("Remaining States"=w12:string, "Current State"=w13:string, "Arguments"=w11:string)  [unwired: 11 in]
    n4 = case shown="\"Process: Calculate Freeze Fraction\"" w13 {
      selector: w13 -> [_ _ w232 _ _ _ _ _ _ _ _ _ _ _ _ _ _ _ _ _ _ _ _ _ _ _ _ _ _ _ _ _ _ _ _ _ _ _ _ _ _ _ _ _ _ _ _ _ _ _ _ _ _ _ _ _ _ _ _ _ _ _ _ _ _ _ _ _]
      tunnel: w12 -> [w20 w231 w236 w255 w261 w266 w270 w287 w296 w304 w309 w326 w382 w410 w440 w445 w452 w459 w475 w526 w555 w590 w598 w606 w613 w618 w625 w637 w649 w659 w669 w684 w701 w770 w775 w785 w789 w794 w799 w816 w838 w885 w955 w985 w1011 w1032 w1041 w1050 w1067 w1074 w1079 w1084 w1093 w1113 w1130 w1196 w1222 w1242 w1260 w1276 w1285 w1294 w1306 w1315 w1355 w1399 w1434 w1450]
      tunnel: w11 -> [_ _ _ _ _ _ _ _ _ _ _ _ _ _ _ _ _ _ _ _ _ _ w594 _ _ w614 w621 w632 w645 w655 w665 w681 w695 _ _ _ _ _ _ _ _ _ _ _ _ _ _ _ _ _ _ _ _ _ w1128 _ _ _ _ _ _ _ _ _ _ _ _ _]
      tunnel: w5 -> [w18 w228 w234 w248 w258 w264 w267 _ w294 w301 w306 w313 w379 w403 w437 w441 w449 w456 w473 w517 w552 w588 w596 w604 w610 w616 w623 w635 w647 w657 w667 w678 w697 w767 w772 w782 w786 w791 w796 w805 w822 w871 w952 w978 w1008 w1029 w1038 w1047 w1064 w1071 w1076 w1081 w1090 w1094 w1126 w1183 w1213 w1233 w1251 w1265 w1283 w1289 w1303 w1312 w1352 w1394 w1431 w1441]
      tunnel: [w17 w229 w238 w252 errorcluster {"status"=FALSE, "code"=0, "source"=""} ("error out") w263 w268 w276 w293 w302 w307 w315 w380 w408 w434 w443 w450 w457 w460 w511 w553 w587 w595 w603 w611 w615 w622 w633 w646 w656 w666 w682 w698 w768 w773 w783 w787 w792 w797 w814 w836 w883 w953 w983 w1009 w1030 w1039 w1048 w1065 w1072 w1077 w1082 w1091 w1111 w1123 w1193 w1220 w1240 w1258 w1274 w1280 w1286 w1304 w1313 w1353 w1397 w1432 w1448] -> w9
      tunnel: w3 -> [w16 w229 w237 w252 w257 w263 w268 w276 w290 w302 w307 w322 w380 w408 w434 w443 w450 w457 w460 w511 w553 w587 w595 w603 w611 w615 w622 w634 w646 w656 w666 w682 w699 w768 w773 w783 w787 w792 w797 w814 w836 w883 w953 w983 w1009 w1030 w1039 w1048 w1065 w1072 w1077 w1082 w1091 w1111 w1124 w1193 w1220 w1240 w1258 w1274 w1281 w1288 w1304 w1313 w1353 w1397 w1432 w1448]
      tunnel: [w19 w230 w235 w254 w260 w265 w269 w286 w295 w303 w308 w325 w381 w409 w439 w444 w451 w458 w474 w525 w554 w589 w597 w605 w612 w617 w624 w636 w648 w658 w668 w683 w700 w769 w774 w784 w788 w793 w798 w815 w837 w884 w954 w984 w1010 w1031 w1040 w1049 w1066 w1073 w1078 w1083 w1092 w1112 w1129 w1195 w1221 w1241 w1259 w1275 w1284 w1293 w1305 w1314 w1354 w1398 w1433 w1449] -> w8
      tunnel: [_ _ _ _ _ TRUE _ _ _ _ _ _ _ _ _ _ _ _ _ _ _ _ _ _ _ _ _ _ _ _ _ _ _ _ _ _ _ _ _ _ _ _ _ _ _ _ _ _ _ _ _ _ _ _ _ _ _ _ _ _ _ _ _ _ _ _ _ _] -> w7
      tunnel: [w15 w228 w234 w253 w258 w264 w267 w285 w294 w300 w305 w324 w379 w402 w438 w441 w449 w455 w473 w517 w552 w588 w596 w604 w610 w616 w623 w635 w647 w657 w667 w678 w697 w767 w772 w782 w786 w791 w796 w805 w821 w871 w952 w978 w1008 w1029 w1038 w1047 w1064 w1071 w1076 w1081 w1090 w1094 w1126 w1182 w1212 w1232 w1250 w1265 w1283 w1289 w1303 w1312 w1352 w1394 w1431 w1441] -> w6
      tunnel: w4 -> [w14 _ _ _ _ _ _ _ _ _ _ _ _ _ _ _ _ _ _ _ _ _ _ _ _ _ _ _ _ _ _ _ _ _ _ _ _ _ _ _ _ _ _ _ _ _ _ _ _ _ _ _ _ _ _ _ _ _ _ _ _ _ _ _ _ _ _ _]
      frame "", "Event Structure", "Idle" {
        # "executes when the state queue is empty"
        n5 = event shown="[1] Menu Selection (User)" {
          selector: _ -> [_ _ _ _ _ _ _ _ _ _ _ _ _ _ _]
          dyn-events: _ -> [_ _ _ _ _ _ _ _ _ _ _ _ _ _ _]
          timeout: w14 -> [_ _ _ _ _ _ _ _ _ _ _ _ _ _ _]
          tunnel: w20 -> [w24 w32 w119 w131 w141 w147 w156 w165 w174 w183 w192 w201 w211 w219 w227]
          tunnel: [w23 w31 w118 w130 w140 w146 w155 w164 w173 w182 w191 w200 w210 w218 w226] -> w19
          tunnel: w18 -> [w21 w26 w116 w128 w138 w144 w153 w162 w171 w180 w189 w198 w208 w216 w224]
          tunnel: [w22 w30 w117 w129 w139 w145 w154 w163 w172 w181 w190 w199 w209 w217 w225] -> w17
          tunnel: w16 -> [w22 w30 w117 w129 w139 w145 w154 w163 w172 w181 w190 w199 w209 w217 w225]
          tunnel: [w21 w25 w116 w128 w138 w144 w153 w162 w171 w180 w189 w198 w208 w216 w224] -> w15
          event Timeout {
            # "Timeout Frame\n(this will only execute if the Event Structure timeout is >= 0)"
            n6 = event-data() -> ()  [unwired: 1 in, 1 out]
            n7 = call <vilib>:"Add State(s) to Queue__jki_lib_state_machine.vi"("State(s) in (\"\")"=w24) -> ("States Out"=w23:string)  [unwired: 14 in]
          }
          event Menu Selection (User) {
            n8 = event-data() -> ("ItemTag"=w29:string)  [unwired: 1 in]
            n9 = local read "recentPaths"() -> (w27:path[])
            n10 = case shown="\"MENU_VALIDATION\"" w29 {
              tunnel: ["" w41 w53 "UI: Cursor Set >> Busy\nUI: Tutorial >> Saving File\nData: Save Results\nUI: Tutorial >> File Saved\nUI: Cursor Set >> Idle" "UI: Cursor Set >> Busy\nUI: Tutorial >> Saving File\nData: Save Results As\nUI: Tutorial >> File Saved\nUI: Cursor Set >> Idle" "Macro: Exit" "Data: Config" "Data: Validate" " Process: Calculate Freezing Points\nProcess: Calculate Freeze Fraction" "UI: Single Temps >> Hide" "" "UI: Single Temps >> Hide" "UI: Cursor Set >> Busy\nUI: Tutorial >> Clearing Overlays\nOverlay: Remove Overlays\nUI: Tutorial >> Adding Freeze Overlay\nUI: Progress >> Show\nOverlay: Overlay Freeze\nUI: Show First Image\nUI: Progress >> Hide\nUI: Tutorial >> Idle\nUI: Cursor Set >> Idle" "UI: Cursor Set >> Busy\nUI: Tutorial >> Clearing Overlays\nOverlay: Remove Overlays\nUI: Tutorial >> Overlaying Freezing Temperatures\nUI: Progress >> Show\nOverlay: Overlay Freeze Temps\nUI: Progress >> Hide\nUI: Show First Image\nUI: Tutorial >> Idle\nUI: Cursor Set >> Idle" "UI: Cursor Set >> Busy\nUI: Tutorial >> Clearing Overlays\nOverlay: Remove Overlays\nUI: Tutorial >> Adding Grid Overlay\nData: Set Image\nImage: Draw\nUI: Show First Image\nUI: Tutorial >> Idle\nUI: Cursor Set >> Idle" "UI: Cursor Set >> Busy\nUI: Tutorial >> Clearing Overlays\nOverlay: Remove Overlays\nUI: Show First Image\nUI: Tutorial >> Idle\nUI: Cursor Set >> Idle" "UI: Cursor Set >> Busy\nUI: Tutorial >> Loading Files\nData: Temps Clear\nData: Load Image\nUI: Tutorial >> Loading Calibration\nData: Load Calibration" "UI: Cursor Set >> Busy\nUI: Tutorial >> Loading Files\nData: Temps Clear\nData: Load Image\nUI: Tutorial >> Loading Calibration\nData: Load Calibration" "UI: Cursor Set >> Busy\nUI: Tutorial >> Loading Files\nData: Temps Clear\nData: Load Image\nUI: Tutorial >> Loading Calibration\nData: Load Calibration" "UI: Cursor Set >> Busy\nUI: Tutorial >> Loading Files\nData: Temps Clear\nData: Load Image\nUI: Tutorial >> Loading Calibration\nData: Load Calibration"] -> w28
              tunnel: w27 -> [_ _ _ _ _ _ _ _ _ _ _ _ _ _ _ _ w96 w102 w108 w114]
              tunnel: w26 -> [w33 w35 w47 w59 w61 w63 w65 w67 w69 w73 w77 w81 w83 w85 w87 w90 w92 w98 w104 w110]
              tunnel: [w33 w35 w47 w59 w61 w63 w65 w67 w69 w72 w76 w80 w83 w85 w87 w90 w92 w98 w104 w110] -> w25
              frame "False", Default {
              }
              frame "DATA_NEW" {
                n11 = call <vilib>:"Application Directory.vi"() -> ("Application Directory"=w40:path)
                n12 = Build Path(base path=w40, name or relative path=path "Data") -> (appended path=w39:path)
                n13 = call "ResultLoadPrompt.vi"("Path"=w39) -> ("selected path"=w36:path, "cancel?"=w37:bool)
                n14 = case shown="False" w37 {
                  tunnel: ["UI: Cursor Set >> Busy\nUI: Tutorial >> Loading Images\nData: Load Image\nUI: Tutorial >> Loading Calibration\nData: Load Calibration" ""] -> w41
                  tunnel: w36 -> [w42 _]
                  frame False {
                    n15 = local write "Path"(w42) -> ()
                    n16 = local write "img"(0 ("img")) -> ()
                    n17 = local write "Slide"(u8 0 ("Slide")) -> ()
                  }
                  frame True {
                  }
                }
              }
              frame "DATA_OPEN" {
                n18 = call <vilib>:"Application Directory.vi"() -> ("Application Directory"=w52:path)
                n19 = Build Path(base path=w52, name or relative path=path "Data") -> (appended path=w50:path)
                n20 = call "ResultLoadPrompt.vi"("Path"=w50) -> ("selected path"=w49:path, "cancel?"=w48:bool)
                n21 = case shown="False" w48 {
                  tunnel: ["UI: Cursor Set >> Busy\nUI: Tutorial >> Loading Files\nData: Temps Clear\nData: Load Image\nUI: Recent Menu Update\nUI: Tutorial >> Loading Calibration\nUI: Recent Menu Update\nData: Load Calibration" ""] -> w53
                  tunnel: w49 -> [w56 _]
                  frame False {
                    n22 = Build Path(base path=w56, name or relative path=path "Result Data.csv") -> (appended path=w54:path)
                    n23 = local write "Path"(w56) -> ()
                    n24 = call "RunTimeMenu_TCE_RecentInsert.vi"("NewPath"=w54) -> ()  [unwired: 11 in]
                  }
                  frame True {
                  }
                }
              }
              frame "DATA_SAVE" {
              }
              frame "DATA_SAVE_AS" {
              }
              frame "MENU_EXIT" {
              }
              frame "MENU_CONFIG" {
              }
              frame "MENU_VALIDATION" {
              }
              frame "MENU_CALC_FREEZE" {
              }
              frame "MENU_GRADIENTS" {
                n25 = Bundle By Name(cluster=w73, "ShowGradient"=TRUE) -> (w72:T4)
              }
              frame "MENU_ENDPOINT" {
                n26 = local read "ImageIdx"() -> (w75:u32)
                n27 = Bundle By Name(cluster=w77, "Config.Freezing.EndIndex"=w75) -> (w76:T4)
              }
              frame "MENU_FRACTION" {
                n28 = Bundle By Name(cluster=w81, "ShowGradient"=FALSE) -> (w80:T4)
              }
              frame "OVERLAY_FREEZE" {
              }
              frame "OVERLAY_TEMPS" {
              }
              frame "OVERLAY_GRID" {
                n29 = local write "ImageIdx"(0 ("img")) -> ()
              }
              frame "OVERLAY_CLEAR" {
              }
              frame "MENU_RECENT_0" {
                n30 = Index Array(array=w96, index=0) -> (element=w94:path)
                n31 = Strip Path(path=w94) -> (stripped path=w93:path)  [unwired: 1 out]
                n32 = local write "Path"(w93) -> ()
              }
              frame "MENU_RECENT_1" {
                n33 = Index Array(array=w102, index=1) -> (element=w100:path)
                n34 = Strip Path(path=w100) -> (stripped path=w99:path)  [unwired: 1 out]
                n35 = local write "Path"(w99) -> ()
              }
              frame "MENU_RECENT_2" {
                n36 = Index Array(array=w108, index=2) -> (element=w106:path)
                n37 = Strip Path(path=w106) -> (stripped path=w105:path)  [unwired: 1 out]
                n38 = local write "Path"(w105) -> ()
              }
              frame "MENU_RECENT_3" {
                n39 = Index Array(array=w114, index=3) -> (element=w112:path)
                n40 = Strip Path(path=w112) -> (stripped path=w111:path)  [unwired: 1 out]
                n41 = local write "Path"(w111) -> ()
              }
            }
            n42 = call <vilib>:"Add State(s) to Queue__jki_lib_state_machine.vi"("State(s) in Front (\"\")"=w28, "State(s) in (\"\")"=w32) -> ("States Out"=w31:string)  [unwired: 13 in]
          }
          event "Help": Value Change {
            # "Timeout Frame\n(this will only execute if the Event Structure timeout is >= 0)"
            n43 = event-data() -> ()  [unwired: 1 in, 6 out]
            n44 = call <vilib>:"Add State(s) to Queue__jki_lib_state_machine.vi"("State(s) in (\"\")"=w119) -> ("States Out"=w118:string)  [unwired: 14 in]
          }
          event "Image": Mouse Wheel {
            n45 = event-data() -> ("Delta"=w127:i32)  [unwired: 1 in, 1 out]
            n46 = property on="Image" class="ImageControl"() -> ("Last Mouse Position"=w121:cluster{"X":i32, "Y":i32}, "X Zoom"=w122:sgl)  [unwired: 2 in, 2 out]
            n47 = Greater Than 0?(x=w127) -> (x > 0?=w126:bool)
            n48 = Select(t=1.2, s=w126, f=0.8) -> (s? t:f=w123:dbl)
            n49 = Multiply(x=w123, y=w122) -> (x*y=w120:dbl)
            n50 = property on="Image" class="ImageControl"("X Zoom"=w120, "Y Zoom"=w120, "Image Center Position"=w121) -> ()  [unwired: 2 in, 2 out]
            n51 = call <vilib>:"Add State(s) to Queue__jki_lib_state_machine.vi"("State(s) in (\"\")"=w131) -> ("States Out"=w130:string)  [unwired: 14 in]
          }
          event "Image": Mouse Up {
            n52 = event-data() -> ()  [unwired: 1 in, 1 out]
            n53 = property on="Image" class="ImageControl"() -> ("Last Mouse Position"=w137:cluster{"X":i32, "Y":i32})  [unwired: 2 in, 2 out]
            n54 = local read "Temps"() -> (w132:dbl[][])
            n55 = local read "Points"() -> (w136:T2[])
            n56 = call "SingleWellUpdater.vi"("Temps"=w132, "Well Coordinates"=w136, "Last Mouse Position"=w137) -> ("Well idx"=w133:i32, "ROI Descriptor"=w134:T11, "State out"=w135:string)  [unwired: 6 in]
            n57 = property on="Image" class="ImageControl"("ROI"=w134) -> ()  [unwired: 2 in, 2 out]
            n58 = local write "Well"(w133) -> ()
            n59 = call <vilib>:"Add State(s) to Queue__jki_lib_state_machine.vi"("State(s) in Front (\"\")"=w135, "State(s) in (\"\")"=w141) -> ("States Out"=w140:string)  [unwired: 13 in]
          }
          event Panel Close? {
            # "Discard the event because we'll close the front panel ourselves in Macro: Exit"
            # "Close Panel button (pressed) Event\n(this executes Macro: Exit to terminate the VI)"
            n60 = event-data() -> ()  [unwired: 1 in, 1 out]
            n61 = call <vilib>:"Add State(s) to Queue__jki_lib_state_machine.vi"("State(s) in Front (\"\")"="Macro: Exit", "State(s) in (\"\")"=w147) -> ("States Out"=w146:string)  [unwired: 13 in]
            n62 = event-data("Discard?"=TRUE) -> ()  [unwired: 1 in, 1 out]
          }
          event "Temps single": Cursor Move {
            n63 = event-data() -> ()  [unwired: 1 in, 9 out]
            n64 = property on="Temps single" class="WFGraph (strict)"() -> ("Cursor.Cursor X"=w151:dbl)  [unwired: 2 in, 2 out]
            n65 = local read "maxSize"() -> (w150:i32)
            n66 = In Range and Coerce(upper limit=w150, x=w151, lower limit=0) -> (coerced(x)=w148:dbl)  [unwired: 1 out]
            n67 = local write "ImageIdx"(w148) -> ()
            n68 = call <vilib>:"Add State(s) to Queue__jki_lib_state_machine.vi"("State(s) in Front (\"\")"="Image: Set Cursors\nData: Set Image\nData: Show Img\nData: Update Well Temp", "State(s) in (\"\")"=w156) -> ("States Out"=w155:string)  [unwired: 13 in]
          }
          event "Temps": Cursor Move {
            n69 = event-data() -> ()  [unwired: 1 in, 1 out]
            n70 = property on="Temps" class="WFGraph (strict)"() -> ("Cursor.Cursor X"=w160:dbl)  [unwired: 2 in, 2 out]
            n71 = local read "maxSize"() -> (w158:i32)
            n72 = In Range and Coerce(upper limit=w158, x=w160, lower limit=0) -> (coerced(x)=w157:dbl)  [unwired: 1 out]
            n73 = local write "ImageIdx"(w157) -> ()
            n74 = call <vilib>:"Add State(s) to Queue__jki_lib_state_machine.vi"("State(s) in Front (\"\")"="Image: Set Cursors\nData: Set Image\nData: Show Img\nData: Update Well Temp", "State(s) in (\"\")"=w165) -> ("States Out"=w164:string)  [unwired: 13 in]
          }
          event "Temps single grad": Cursor Move {
            n75 = event-data() -> ()  [unwired: 1 in, 1 out]
            n76 = property on="Temps single grad" class="WFGraph (strict)"() -> ("Cursor.Cursor X"=w169:dbl)  [unwired: 2 in, 2 out]
            n77 = local read "maxSize"() -> (w167:i32)
            n78 = In Range and Coerce(upper limit=w167, x=w169, lower limit=0) -> (coerced(x)=w166:dbl)  [unwired: 1 out]
            n79 = local write "ImageIdx"(w166) -> ()
            n80 = call <vilib>:"Add State(s) to Queue__jki_lib_state_machine.vi"("State(s) in Front (\"\")"="Image: Set Cursors\nData: Set Image\nData: Show Img\nData: Update Well Temp", "State(s) in (\"\")"=w174) -> ("States Out"=w173:string)  [unwired: 13 in]
          }
          event "FrozenFractionGraph": Cursor Move {
            n81 = event-data() -> ()  [unwired: 1 in, 1 out]
            n82 = property on="FrozenFractionGraph" class="WFGraph (strict)"() -> ("Cursor.Cursor X"=w178:dbl)  [unwired: 2 in, 2 out]
            n83 = local read "maxSize"() -> (w176:i32)
            n84 = In Range and Coerce(upper limit=w176, x=w178, lower limit=0) -> (coerced(x)=w175:dbl)  [unwired: 1 out]
            n85 = local write "ImageIdx"(w175) -> ()
            n86 = call <vilib>:"Add State(s) to Queue__jki_lib_state_machine.vi"("State(s) in Front (\"\")"="Image: Set Cursors\nData: Set Image\nData: Show Img\nData: Update Well Temp", "State(s) in (\"\")"=w183) -> ("States Out"=w182:string)  [unwired: 13 in]
          }
          event "Fraction Single": Cursor Move {
            n87 = event-data() -> ()  [unwired: 1 in, 1 out]
            n88 = property on="Fraction Single" class="WFGraph (strict)"() -> ("Cursor.Cursor X"=w187:dbl)  [unwired: 2 in, 2 out]
            n89 = local read "maxSize"() -> (w185:i32)
            n90 = In Range and Coerce(upper limit=w185, x=w187, lower limit=0) -> (coerced(x)=w186:dbl)  [unwired: 1 out]
            n91 = local write "ImageIdx"(w186) -> ()
            n92 = call <vilib>:"Add State(s) to Queue__jki_lib_state_machine.vi"("State(s) in Front (\"\")"="Image: Set Cursors\nData: Set Image\nData: Show Img\nData: Update Well Temp", "State(s) in (\"\")"=w192) -> ("States Out"=w191:string)  [unwired: 13 in]
          }
          event "Temps grads": Cursor Move {
            n93 = event-data() -> ()  [unwired: 1 in, 9 out]
            n94 = property on="Temps grads" class="WFGraph (strict)"() -> ("Cursor.Cursor X"=w196:dbl)  [unwired: 2 in, 2 out]
            n95 = local read "maxSize"() -> (w195:i32)
            n96 = In Range and Coerce(upper limit=w195, x=w196, lower limit=0) -> (coerced(x)=w193:dbl)  [unwired: 1 out]
            n97 = local write "ImageIdx"(w193) -> ()
            n98 = call <vilib>:"Add State(s) to Queue__jki_lib_state_machine.vi"("State(s) in Front (\"\")"="Image: Set Cursors\nData: Set Image\nData: Show Img\nData: Update Well Temp", "State(s) in (\"\")"=w201) -> ("States Out"=w200:string)  [unwired: 13 in]
          }
          event "Calc_All": Value Change {
            w202 = FALSE ("Visible")
            w206 = u8 0 ("Slide")
            n99 = event-data() -> ()  [unwired: 1 in, 6 out]
            n100 = local write "ImageIdx"(w206) -> ()
            n101 = local write "Slide"(w206) -> ()
            n102 = local write "img"(0 ("img")) -> ()
            n103 = property on="Temps" class="WFGraph (strict)"("Visible"=TRUE) -> ()  [unwired: 2 in, 2 out]
            n104 = property on="Temps single" class="WFGraph (strict)"("Visible"=w202) -> ()  [unwired: 2 in, 2 out]
            n105 = property on="Temps single grad" class="WFGraph (strict)"("Visible"=w202) -> ()  [unwired: 2 in, 2 out]
            n106 = property on="Temp grads" class="WFGraph (strict)"("Visible"=w202) -> ()  [unwired: 2 in, 2 out]
            n107 = local write "Offset Applied?"(FALSE ("Offset Applied?")) -> ()
            n108 = call <vilib>:"Add State(s) to Queue__jki_lib_state_machine.vi"("State(s) in Front (\"\")"="Process: Calculate All", "State(s) in (\"\")"=w211) -> ("States Out"=w210:string)  [unwired: 13 in]
          }
          event "Correct Data": Value Change {
            n109 = event-data() -> ()  [unwired: 1 in, 6 out]
            n110 = property on="Correct Data" class="Bool"("Visible"=FALSE) -> ()  [unwired: 2 in, 2 out]
            n111 = property on="Remove_Correction" class="Bool"("Visible"=TRUE) -> ()  [unwired: 2 in, 2 out]
            n112 = call <vilib>:"Add State(s) to Queue__jki_lib_state_machine.vi"("State(s) in Front (\"\")"="UI: Cursor Set >> Busy\nUI: Tutorial >> Correcting Data\nProcess: Correct Offset\nProcess: Recalculate\nOverlay: Update Focus Well\nUI: Tutorial >> Done\nUI: Cursor Set >> Idle", "State(s) in (\"\")"=w219) -> ("States Out"=w218:string)  [unwired: 13 in]
            "Offset Applied?" <- TRUE ("Offset Applied?")
          }
          event "Remove_Correction": Value Change {
            n113 = event-data() -> ()  [unwired: 1 in, 6 out]
            n114 = property on="Remove_Correction" class="Bool"("Visible"=FALSE) -> ()  [unwired: 2 in, 2 out]
            n115 = property on="Correct Data" class="Bool"("Visible"=TRUE) -> ()  [unwired: 2 in, 2 out]
            n116 = local write "Offset Applied?"(FALSE ("Offset Applied?")) -> ()
            n117 = call <vilib>:"Add State(s) to Queue__jki_lib_state_machine.vi"("State(s) in Front (\"\")"="UI: Cursor Set >> Busy\nUI: Tutorial >> Correcting Data\nProcess: Remove Offset\nProcess: Recalculate\nOverlay: Update Focus Well\nUI: Tutorial >> Done\nUI: Cursor Set >> Idle", "State(s) in (\"\")"=w227) -> ("States Out"=w226:string)  [unwired: 13 in]
          }
        }
      }
      frame "---------- Core ----------" {
        # "Do not put any code in this frame.\n(it is a separator no-op)"
        n118 = call <vilib>:"Add State(s) to Queue__jki_lib_state_machine.vi"("State(s) in (\"\")"=w231) -> ("States Out"=w230:string)  [unwired: 14 in]
      }
      frame Default {
        w241 = 42 items=["No error", "Argument error", "Memory is full", "Out of zone", "End of file", "File already open", "Generic file I/O error", "File not found", "File permission error", "Disk is full", "Duplicate path", "Too many files open", "System feature not enabled", "Resource file not found", "Cannot add resource", "Resource not found", "Image not found", "Image memory error", "Pen does not exist", "Config type invalid", "Config token not found", "Config parse error", "Config memory error", "Bad external code format", "Bad external code offset", "External code not present", "Null window", "Destroy window error", "Null menu", "Print aborted", "Bad print record", "Print driver error", "Windows error during printing", "Memory error during printing", "Print dialog error", "Generic print error", "Invalid device refnum", "Device not found", "Device parameter error", "Device unit error", "Cannot open device", "Device call aborted", "Generic error", "Cancelled by user", "Object ID too low", "Object ID too high", "Object not in heap", "Unknown heap", "Unknown object (invalid DefProc)", "Unknown object (DefProc not in table)", "Message out of range", "Invalid (null) method", "Unknown message", "Manager call not supported", "Bad address", "Network operation in progress", "Network operation timed out", "Connection is busy", "Network attribute not supported", "Network error", "Address in use", "System out of memory", "Connection aborted", "Connection refused", "Not connected", "Already connected", "Connection closed", "Initialization error (interapplication manager)", "Bad occurrence", "Wait on unbound occurrence handler", "Occurrence queue overflow", "Datalog type conflict", "Unused", "Unrecognized type (interapplication manager)", "Memory corrupt", "Failed to make temporary DLL", "Old CIN version", "Drag socket not found", "Failed to load drop-object", "Failed to register OLE object", "Failed to release OLE object", "Format specifier type mismatch", "Unknown format specifier", "Too few format specifiers", "Too many format specifiers", "Scan failed", "Newer CIN version", "Error converting to variant", "Runtime menu error", "Password tampered", "Variant attribute not found", "Incompatible variant data type", "Event data is not available", "Event Store is not present", "Occurrence is not found", "Event Queue is not created", "Event info is not available", "Refnum passed is NULL", "Error retrieving Class GUID", "Error retrieving CoClass GUID", "Error retrieving TypeLib GUID.", "Bad built application magic bytes.", "Specific driver is different from the specific driver associated with the Logical Name.", "There is no session opened to the class driver.", "Max Error", "MAX - Error with config objects", "MAX - Error loading configuration", "MAX - Group not supported"]
        # "Current State"
        # "Do not delete, rename, or modify this frame.\n(this is used to capture unhandled states and typos)"
        # "Handle mistyped state name (developer tool)"
        n119 = Format Into String(format string="Software Exception: Unhandled State \"%s\"." ("message"), error in=w237, w232) -> (resulting string=w240:string, error out=w239:errorcluster)  [unwired: 1 in]
        n120 = call <vilib>:"Error Cluster From Error Code.vi"("show call chain? (False)"=TRUE, "error in (no error)"=w239, "error message (\"\")"=w240, "error code (0)"=w241) -> ("error out"=w238:errorcluster)  [unwired: 5 in]
        n121 = call <vilib>:"Add State(s) to Queue__jki_lib_state_machine.vi"("State(s) in (\"\")"=w236) -> ("States Out"=w235:string)  [unwired: 14 in]
      }
      frame "Initialize Core Data" {
        # "Do not delete, rename, or modify this frame.\n(this is used to determine panel behavior on exit)"
        # "originally closed?"
        # "exe?"
        # "If panel starts closed or is an EXE, then close it when we exit"
        n122 = property class="App"() -> ("App.Kind"=w251:T6)  [unwired: 2 in, 2 out]
        n123 = control-ref of="Current VI Reference"() -> (w246:refnum<vi>)
        n124 = property class="VI"() -> ("FP.State"=w245:T5)  [unwired: 2 in, 2 out]
        n125 = Equal?(x=w245, y=T5."Closed" ("Front Panel Window:State")) -> (x = y?=w243:bool)
        n126 = Equal?(x=w251, y=T6."Run Time System" ("Application:Kind")) -> (x = y?=w249:bool)
        n127 = Or(x=w243, y=w249) -> (x .or. y?=w247:bool)
        n128 = Bundle By Name(cluster=w248, "Core.Current VI Reference"=w246, "Core.Close Panel on Exit?"=w247) -> (w253:T4)
        n129 = call <vilib>:"Add State(s) to Queue__jki_lib_state_machine.vi"("State(s) in (\"\")"=w255) -> ("States Out"=w254:string)  [unwired: 14 in]
      }
      frame "Error Handler" {
        # "Unhandled Error -- Display it"
        # "Handle any errors here.\nYou can also output any states to clean-up after errors occur"
        # "Clear error"
        n130 = call <vilib>:"General Error Handler.vi"("error in (no error)"=w257) -> ()  [unwired: 10 in, 5 out]
        n131 = call <vilib>:"Add State(s) to Queue__jki_lib_state_machine.vi"("State(s) in Front (\"\")"="/* Post Error States", "State(s) in (\"\")"=w261) -> ("States Out"=w260:string)  [unwired: 13 in]
      }
      frame "Exit" {
        # "Do not put any code in this frame.\n(No errors that occur here will be handled.)"
        n132 = call <vilib>:"Add State(s) to Queue__jki_lib_state_machine.vi"("State(s) in (\"\")"=w266) -> ("States Out"=w265:string)  [unwired: 14 in]
      }
      frame "---------- Data ----------" {
        # "Do not put any code in this frame.\n(It is a separator no-op. You can make a copy of this frame to create a new Data frame)"
        n133 = call <vilib>:"Add State(s) to Queue__jki_lib_state_machine.vi"("State(s) in (\"\")"=w270) -> ("States Out"=w269:string)  [unwired: 14 in]
      }
      frame "Data: Initialize" {
        w275 = dbl[] [] ("Offsets")
        w277 = dbl[][] []  # Temps_Array
        w278 = dbl[] []  # Temps
        w281 = T1[] []  # img_array
        w283 = u32 1 items=["Zoom Tool"=8, "Selection Tool"=0, "Pan Tool"=9, "Point Tool"=1, "Line Tool"=2, "Rectangle Tool"=3, "Rotated Rectangle Tool"=12, "Polyline Tool"=10, "Polygon Tool"=5, "Freehand Tool"=11, "Closed Freehand Tool"=6, "Ellipse Tool"=4, "Annulus Tool"=7] ("Current ROI Tool")
        w280 = 0  # State
        w284 = T12 {"Current VI Reference"=refnum, "Close Panel on Exit?"=FALSE}  # Core
        # "Initialize the shift-register data, here.\n(data names are defined by what you wire into the bundle function)"
        n134 = property on="Image" class="ImageControl"("Current ROI Tool"=w283) -> ()  [unwired: 2 in, 2 out]
        n135 = local write "Offsets"(w275) -> ()
        n136 = local write "FreezeFract Concatinated"(w275) -> ()
        n137 = local write "ThermTemps"(w275) -> ()
        n138 = local write "Slide"(w280) -> ()
        n139 = call "TCE_Config_Load.vi"() -> ("error out"=w272:errorcluster, "Config"=w274:T3)  [unwired: 10 in]
        n140 = call "TCE_Config_Save.vi"("error in"=w272, "Config"=w274) -> ("Config dup"=w273:T3)  [unwired: 8 in, 1 out]
        n141 = Bundle By Name(cluster=T4 {"Core"={"Current VI Reference"=refnum, "Close Panel on Exit?"=FALSE}, "Image Out"=refnum, "State"=0, "Points"={"Top Left"={"X"=0.0, "Y"=0.0}, "Top Right"={"X"=0.0, "Y"=0.0}, "Bottom Left"={"X"=0.0, "Y"=0.0}, "Bottom Right"={"X"=0.0, "Y"=0.0}, "x space 2"=0.0, "y space 2"=0.0, "x_space"=0.0, "y_space"=0.0, "Pixels"=[], "Fixpoint"={"X"=0.0, "Y"=0.0}}, "img_array"=[], "Temps"=[], "Temps_Array"=[], "Scan Area"=0.0, "Fixpoint Area"=0.0, "Config"={"Freezing"={"Cutoff"=2.0, "EndIndex"=2}}, "PCR Size"=0, "ImageCount"=0, "ShowGradient"=FALSE, "Save Well data"=FALSE, "Save Blackbody data"=FALSE, "Save Temps For Offset"=FALSE} ("Cluster"), "Core"=w284, "Image Out"=T1 refnum, "State"=w280, "img_array"=w281, "Temps"=w278, "Temps_Array"=w277, "Config"=w273, "ShowGradient"=FALSE) -> (w285:T4)
        n142 = call <vilib>:"Add State(s) to Queue__jki_lib_state_machine.vi"("State(s) in (\"\")"=w287) -> ("States Out"=w286:string)  [unwired: 14 in]
      }
      frame "Data: Cleanup" {
        # "Cleanup any data and references, here.\n(this is called automatically, by the Macro: Exit)"
        n143 = Unbundle By Name(w294) -> ("Config"=w288:T3, "img_array"=w292:T1[], "Image Out"=w291:T1)
        n144 = call "TCE_Config_Save.vi"("Config"=w288) -> ()  [unwired: 9 in, 2 out]
        n145 = call "IMAQ Dispose"("Image"=w291, "error in (no error)"=w290) -> ("error out"=w289:errorcluster)  [unwired: 4 in]
        n146 = for {
          shift-right: [w298] -> w293
          shift-left: w289 -> [w299]
          tunnel: w292 -> [w297] mode=indexing
          n147 = call "IMAQ Dispose"("Image"=w297, "error in (no error)"=w299) -> ("error out"=w298:errorcluster)  [unwired: 4 in]
        }
        n148 = call <vilib>:"Add State(s) to Queue__jki_lib_state_machine.vi"("State(s) in (\"\")"=w296) -> ("States Out"=w295:string)  [unwired: 14 in]
      }
      frame "Data: Config" {
        # "Do not put any code in this frame.\n(It is a separator no-op. You can make a copy of this frame to create a new Data frame)"
        n149 = call "TCE_Config.vi"("Cluster"=w301) -> ("Config out"=w300:T4)  [unwired: 9 in, 1 out]
        n150 = call <vilib>:"Add State(s) to Queue__jki_lib_state_machine.vi"("State(s) in (\"\")"=w304) -> ("States Out"=w303:string)  [unwired: 14 in]
      }
      frame "Data: Validate" {
        # "Do not put any code in this frame.\n(It is a separator no-op. You can make a copy of this frame to create a new Data frame)"
        n151 = call "Validation_Data.vi"("Data Cluster"=w306) -> ("Data Cluster Out"=w305:T4)
        n152 = call <vilib>:"Add State(s) to Queue__jki_lib_state_machine.vi"("State(s) in (\"\")"=w309) -> ("States Out"=w308:string)  [unwired: 14 in]
      }
      frame "Data: Load Image" {
        # "Do not put any code in this frame.\n(It is a separator no-op. You can make a copy of this frame to create a new Data frame)"
        n153 = local write "Slide"(u8 0 ("Slide")) -> ()
        n154 = local write "img"(0 ("img")) -> ()
        n155 = Empty String/Path?(string/path="Path") -> (empty?=w320:bool)
        n156 = case shown="False" w320 {
          tunnel: [w341 _] -> w323
          tunnel: w322 -> [w338 w372]
          tunnel: [w342 w372] -> w316
          tunnel: "Path" -> [w330 _]
          tunnel: [w340 _] -> w318
          tunnel: w313 -> [w332 _]
          tunnel: [w327 0] -> w310
          frame False {
            n157 = Build Path(base path=w330, name or relative path=path "Images") -> (appended path=w333:path)
            n158 = List Folder(path=w333) -> (filenames=w328:string[])  [unwired: 3 in, 3 out]
            n159 = property on="Slide" class="Slide (strict)"(error in=w338, "Visible"=TRUE) -> (error out=w337:errorcluster)  [unwired: 1 in, 1 out]
            n160 = call "Partition_Extract.vi"("input cluster"=w332, "Path"=w330) -> ("PartitionArray"=→"PartitionArray":string[])
            n161 = call "Thermistor_Extract.vi"("Path"=w330, "filenames"=w328) -> ("ThermTemps"=→"ThermTemps":dbl[])
            n162 = Array Size(array=w328) -> (size(s)=w336:i32)
            n163 = Format Into String(w336) -> (resulting string=w335:string)  [unwired: 3 in, 1 out]
            n164 = for {
              tunnel: [w370] -> w344
              tunnel: [w354] -> w340 mode=indexing
              tunnel: [w357] -> _ mode=indexing
              tunnel: w328 -> [w362] mode=indexing
              tunnel: w333 -> [w361]
              tunnel: w336 -> [w356]
              tunnel: w337 -> [w357]
              workers-P: _ -> [_]
              tunnel: w335 -> [w346]
              i -> [w355]
              w365 = T13 7 items=["Grayscale (U8)", "Grayscale (I16)", "Grayscale (SGL)", "Complex (CSG)", "RGB (U32)", "HSL (U32)", "RGB (U64)", "Grayscale (U16)"] ("Image Type")
              n165 = Format Into String(w355) -> (resulting string=w363:string)  [unwired: 3 in, 1 out]
              n166 = local read "img"() -> (w353:i32)
              n167 = Concatenate Strings("img_" ("Image Name"), w363) -> (w364:string)
              n168 = Build Path(base path=w361, name or relative path=w362) -> (appended path=w360:path)
              n169 = Increment(x=w353) -> (x+1=w347:i32)
              n170 = call "IMAQ Create"("Image Name"=w364, "Image Type"=w365, "error in (no error)"=w357) -> ("New Image"=w368:T1, "error out"=w369:errorcluster)  [unwired: 2 in]
              n171 = Format Into String(w347) -> (resulting string=w350:string)  [unwired: 3 in, 1 out]
              n172 = local write "img"(w347) -> ()
              n173 = call "IMAQ ReadFile 2"("File Path"=w360, "error in (no error)"=w369, "Image"=w368) -> ("error out"=w367:errorcluster, "Image Out"=w345:T1)  [unwired: 4 in, 3 out]
              n174 = Divide(x=w347, y=w356) -> (x/y=w359:dbl)
              n175 = Concatenate Strings("Loading image " ("Tutorial"), w350, " of " ("Tutorial"), w346) -> (w351:string)
              n176 = Multiply(x=w359, y=100.0) -> (x*y=→"Slide":dbl)
              n177 = local write "Tutorial"(w351) -> ()
              n178 = call "IMAQ Clear Overlay"("error in (no error)"=w367, "Image"=w345) -> ("error out"=w370:errorcluster, "Image Out"=w354:T1)  [unwired: 8 in]
              n179 = local write "Image"(w354) -> ()
            }
            n180 = Decrement(x=w336) -> (x-1=w327:i32)
            "maxSize" <- w327
            n181 = Index Array(array=w340) -> (element=w341:T1)  [unwired: 1 in]
            "Image" <- w341
            n182 = property on="Image" class="ImageControl"(error in=w344, "ROI"=T7 {"Global Rectangle"=[], "Contours"=[]}) -> (error out=w342:errorcluster)  [unwired: 1 in, 1 out]
          }
          frame True {
            (unwired) FALSE ("Visible")
          }
        }
        n183 = property on="Slide" class="Slide (strict)"(error in=w316, "Visible"=FALSE) -> (error out=w315:errorcluster)  [unwired: 1 in, 1 out]
        n184 = Bundle By Name(cluster=w313, "Image Out"=w323, "img_array"=w318, "Config.Freezing.EndIndex"=w310, "ImageCount"=w310) -> (w324:T4)
        n185 = local write "ImageIdx"(u32 0 ("Image")) -> ()
        n186 = call <vilib>:"Add State(s) to Queue__jki_lib_state_machine.vi"("State(s) in Front (\"\")"="Image: Set Cursors\nImage: Draw" ("State(s) in Front (\"\")"), "State(s) in (\"\")"=w326) -> ("States Out"=w325:string)  [unwired: 13 in]
      }
      frame "Data: Load Results" {
        # "Do not put any code in this frame.\n(It is a separator no-op. You can make a copy of this frame to create a new Data frame)"
        n187 = local read "Path"() -> (w375:path)
        n188 = Build Path(base path=w375, name or relative path=path "Data.TCE") -> (appended path=w376:path)
        n189 = call <vilib>:"Check if File or Folder Exists.vi"("path"=w376) -> ("file or folder exists?"=w378:bool, "dup path"=w377:path)  [unwired: 8 in, 1 out]
        n190 = case shown="True" w378 {
          tunnel: w377 -> [_ w392]
          tunnel: ["" ("State(s) in Front (\"\")") "UI: Single Temps >> Hide" ("State(s) in Front (\"\")")] -> w373
          frame False {
          }
          frame True {
            n191 = call-poly <vilib>:"Read Delimited Spreadsheet.vi"("file path (dialog if empty)"=w392, "delimiter (\\t)"=";" ("delimiter (\\t)")) -> ("all rows"=w391:string[][])  [unwired: 8 in, 5 out]
            n192 = call <vilib>:"Application Directory.vi"() -> ("Application Directory"=w394:path)
            n193 = Path To String(path=w392) -> (string=w399:string)
            n194 = call "DataArray_Reformatter.vi"("Data Array"=w391) -> ("MeltTemps"=w384:dbl[], "Offsets"=w387:dbl[], "FreezeTemps"=w390:dbl[], "Temps"=w389:dbl[][], "Offset Applied"=w386:bool)
            n195 = Build Path(base path=w394, name or relative path=path "TCEM.ini" ("file path (dialog if empty)")) -> (appended path=w395:path)
            n196 = Build Array(w399) -> (w398:string[])
            n197 = Not(x=w386) -> (.not. x?=w385:bool)
            n198 = local write "Offsets"(w387) -> ()
            n199 = local write "Offset Applied?"(w386) -> ()
            n200 = property on="Remove_Correction" class="Bool"("Visible"=w386) -> ()  [unwired: 2 in, 2 out]
            n201 = local write "MeltTemps"(w384) -> ()
            n202 = local write "Temps"(w389) -> ()
            n203 = local write "FreezeTemps"(w390) -> ()
            n204 = call-poly <vilib>:"Write Delimited Spreadsheet.vi"("file path (dialog if empty)"=w395, "1D data"=w398, "append to file? (new file:F)"=TRUE) -> ()  [unwired: 11 in, 2 out]
            n205 = property on="Correct Data" class="Bool"("Visible"=w385) -> ()  [unwired: 2 in, 2 out]
          }
        }
        n206 = call <vilib>:"Add State(s) to Queue__jki_lib_state_machine.vi"("State(s) in Front (\"\")"=w373, "State(s) in (\"\")"=w382) -> ("States Out"=w381:string)  [unwired: 13 in]
      }
      frame "Data: Load Calibration" {
        # "Do not put any code in this frame.\n(It is a separator no-op. You can make a copy of this frame to create a new Data frame)"
        n207 = local read "Path"() -> (w401:path)
        n208 = Build Path(base path=w401, name or relative path=path "TCC.cal") -> (appended path=w406:path)
        n209 = call <vilib>:"Check if File or Folder Exists.vi"("path"=w406) -> ("file or folder exists?"=w407:bool, "dup path"=w404:path)  [unwired: 8 in, 1 out]
        n210 = case shown="False" w407 {
          tunnel: w404 -> [_ w432]
          tunnel: w403 -> [w412 w431]
          tunnel: [w413 w430] -> w402
          tunnel: w401 -> [w416 _]
          tunnel: [w411 "Image: Draw\nData: Load Results\nData: Set Image\nProcess: Recalculate\nUI: Calc >> True\nUI: Menu Overlay Grid >> True\nUI: Menu Overlay Temps >> True\nUI: Progress >> Hide\nUI: Cursor Set >> Idle\nUI: Tutorial >> Click on a Well to show single or click outside the plate to show all."] -> w400
          frame False {
            n211 = call "CalibrationLoadPrompt.vi"("Root Path"=w416) -> ("cancel?"=w414:bool, "selected path"=w415:path)  [unwired: 9 in]
            n212 = case shown="False" w414 {
              tunnel: w415 -> [w420 _]
              tunnel: [w418 w425] -> w413
              tunnel: w412 -> [w419 w425]
              tunnel: ["Image: Draw\nData: Load Results\nData: Set Image\nProcess: Recalculate\nUI: Menu Overlay Grid >> True\nUI: Menu Overlay Temps >> True\nUI: Calc >> True\nUI: Progress >> Hide\nUI: Cursor Set >> Idle\nUI: Tutorial >> Click on a Well to show single or click outside the plate to show all." "UI: Calc >> Disable\nUI: Progress >> Hide\nUI: Cursor Set >> Idle\nUI: Tutorial >> Error: Missing Calibration File!"] -> w411
              frame False {
                n213 = call "TCam_Calibration_LoadSettings.vi"("path"=w420) -> ("Fixpoint Area"=w421:dbl, "Scan Area"=w422:dbl, "Points"=w423:T14)  [unwired: 7 in, 1 out]
                n214 = Bundle By Name(cluster=w419, "Points"=w423, "Scan Area"=w422, "Fixpoint Area"=w421) -> (w418:T4)
              }
              frame True {
              }
            }
          }
          frame True {
            n215 = call "TCam_Calibration_LoadSettings.vi"("path"=w432) -> ("Fixpoint Area"=w428:dbl, "Scan Area"=w429:dbl, "Points"=w426:T14)  [unwired: 7 in, 1 out]
            n216 = Bundle By Name(cluster=w431, "Points"=w426, "Scan Area"=w429, "Fixpoint Area"=w428) -> (w430:T4)
          }
        }
        n217 = call <vilib>:"Add State(s) to Queue__jki_lib_state_machine.vi"("State(s) in Front (\"\")"=w400, "State(s) in (\"\")"=w410) -> ("States Out"=w409:string)  [unwired: 13 in]
      }
      frame "Data: Set Image" {
        # "Do not put any code in this frame.\n(It is a separator no-op. You can make a copy of this frame to create a new Data frame)"
        n218 = Unbundle By Name(w437) -> ("img_array"=w436:T1[])
        n219 = Index Array(array=w436, index="ImageIdx") -> (element=w433:T1)
        n220 = Bundle By Name(cluster=w437, "Image Out"=w433) -> (w438:T4)
        n221 = call <vilib>:"Add State(s) to Queue__jki_lib_state_machine.vi"("State(s) in (\"\")"=w440) -> ("States Out"=w439:string)  [unwired: 14 in]
      }
      frame "Data: Show Img" {
        # "Do not put any code in this frame.\n(It is a separator no-op. You can make a copy of this frame to create a new Data frame)"
        n222 = Unbundle By Name(w441) -> ("Image Out"=w442:T1)
        n223 = local write "Image"(w442) -> ()
        n224 = call <vilib>:"Add State(s) to Queue__jki_lib_state_machine.vi"("State(s) in (\"\")"=w445) -> ("States Out"=w444:string)  [unwired: 14 in]
      }
      frame "Data: Update Well Temp" {
        # "Initialize the shift-register data, here.\n(data names are defined by what you wire into the bundle function)"
        n225 = local read "Temps single"() -> (w447:dbl[])
        n226 = local read "ImageIdx"() -> (w448:u32)
        n227 = Index Array(array=w447, index=w448) -> (element=w446:dbl)
        n228 = local write "CurTemp"(w446) -> ()
        n229 = call <vilib>:"Add State(s) to Queue__jki_lib_state_machine.vi"("State(s) in (\"\")"=w452) -> ("States Out"=w451:string)  [unwired: 14 in]
      }
      frame "Data: Temps Clear" {
        w453 = dbl[][] [] ("Temps_Array")
        w454 = dbl[] []  # Temps
        # "Initialize the shift-register data, here.\n(data names are defined by what you wire into the bundle function)"
        n230 = local write "Temps single"(w454) -> ()
        n231 = local write "Temps grads"(w453) -> ()
        n232 = local write "Temps"(w453) -> ()
        n233 = local write "Temps single grad"(w454) -> ()
        n234 = Bundle By Name(cluster=w456, "Temps"=w454, "Temps_Array"=w453) -> (w455:T4)
        n235 = call <vilib>:"Add State(s) to Queue__jki_lib_state_machine.vi"("State(s) in (\"\")"=w459) -> ("States Out"=w458:string)  [unwired: 14 in]
      }
      frame "Data: Save Results" {
        # "Initialize the shift-register data, here.\n(data names are defined by what you wire into the bundle function)"
        n236 = local read "Temps"() -> (w472:dbl[][])
        n237 = local read "FreezeTemps"() -> (w471:dbl[])
        n238 = local read "MeltTemps"() -> (w469:dbl[])
        n239 = local read "FreezeFract Concatinated"() -> (w470:dbl[])
        n240 = local read "PartitionArray"() -> (w468:string[])
        n241 = local read "Offsets"() -> (w467:dbl[])
        n242 = local read "Offset Applied?"() -> (w466:bool)
        n243 = call "TCE_SaveConfiguration.vi"("input cluster"=w473, "Temps"=w472, "FreezeTemps"=w471, "MeltTemps"=w469, "FrozenFraction"=w470, "PartitionArray"=w468, "Offsets"=w467, "Offset Applied?"=w466) -> ("Save Array out"=w464:string[][], "Full Array"=w463:string[][], "Canceled"=w462:bool)  [unwired: 9 in]
        n244 = case shown="False" w462 {
          tunnel: w460 -> [w490 w510]
          tunnel: w464 -> [w483 _]
          tunnel: [w482 "" ("State(s) in Front (\"\")")] -> w465
          tunnel: w463 -> [w478 _]
          tunnel: [w477 w510] -> w461
          frame False {
            n245 = local read "Path"() -> (w480:path)
            n246 = Build Path(base path=w480, name or relative path=path "Result Data.csv") -> (appended path=w485:path)
            n247 = Build Path(base path=w480, name or relative path=path "Data.TCE") -> (appended path=w479:path)
            n248 = call <vilib>:"Check if File or Folder Exists.vi"("path"=w485) -> ("file or folder exists?"=w488:bool, "dup path"=w484:path)  [unwired: 8 in, 1 out]
            n249 = case shown="True" w488 {
              selector: w488 -> [_ w496]
              tunnel: w480 -> [w494 _]
              tunnel: [w493 w495] -> w487
              tunnel: [w491 w496] -> w486
              tunnel: w484 -> [_ w495]
              frame False {
                n250 = call "ResultSavePrompt.vi"("Path"=w494) -> ("selected path"=w493:path, "cancel?"=w492:bool)
                n251 = Not(x=w492) -> (.not. x?=w491:bool)
              }
              frame True {
              }
            }
            n252 = case shown="True" w486 {
              tunnel: w483 -> [_ w508]
              tunnel: w490 -> [w497 w507]
              tunnel: w487 -> [_ w506]
              tunnel: ["" ("State(s) in Front (\"\")") "UI: Recent Menu Update" ("State(s) in Front (\"\")")] -> w482
              tunnel: w479 -> [_ w504]
              tunnel: w478 -> [_ w503]
              tunnel: [w497 w500] -> w477
              frame False {
              }
              frame True {
                w502 = ";" ("delimiter (\\t)")
                n253 = call-poly <vilib>:"Write Delimited Spreadsheet.vi"("file path (dialog if empty)"=w506, "2D data"=w508, "error in (no error)"=w507, "delimiter (\\t)"=w502) -> ("error out"=w501:errorcluster)  [unwired: 10 in, 1 out]
                n254 = call-poly <vilib>:"Write Delimited Spreadsheet.vi"("file path (dialog if empty)"=w504, "2D data"=w503, "error in (no error)"=w501, "delimiter (\\t)"=w502) -> ("new file path (Not A Path if cancelled)"=w499:path, "error out"=w500:errorcluster)  [unwired: 10 in]
                n255 = call "RunTimeMenu_TCE_RecentInsert.vi"("NewPath"=w499) -> ()  [unwired: 11 in]
              }
            }
          }
          frame True {
          }
        }
        n256 = case shown="Error .." w461 {
          frame No Error {
          }
          frame Error {
            n257 = One Button Dialog(message="File Save Error!\nClose file if open.") -> ()  [unwired: 1 in, 1 out]
          }
        }
        n258 = call <vilib>:"Add State(s) to Queue__jki_lib_state_machine.vi"("State(s) in Front (\"\")"=w465, "State(s) in (\"\")"=w475) -> ("States Out"=w474:string)  [unwired: 13 in]
      }
      frame "Data: Save Results As" {
        # "Initialize the shift-register data, here.\n(data names are defined by what you wire into the bundle function)"
        n259 = local read "FreezeFract Concatinated"() -> (w522:dbl[])
        n260 = local read "Offset Applied?"() -> (w518:bool)
        n261 = local read "PartitionArray"() -> (w520:string[])
        n262 = local read "FreezeTemps"() -> (w523:dbl[])
        n263 = local read "MeltTemps"() -> (w521:dbl[])
        n264 = local read "Offsets"() -> (w519:dbl[])
        n265 = local read "Temps"() -> (w524:dbl[][])
        n266 = call "TCE_SaveConfiguration.vi"("input cluster"=w517, "Temps"=w524, "FreezeTemps"=w523, "MeltTemps"=w521, "FrozenFraction"=w522, "PartitionArray"=w520, "Offsets"=w519, "Offset Applied?"=w518) -> ("Save Array out"=w516:string[][], "Full Array"=w513:string[][], "Canceled"=w514:bool)  [unwired: 9 in]
        n267 = case shown="False" w514 {
          tunnel: w511 -> [w535 w550]
          tunnel: w516 -> [w532 _]
          tunnel: [w531 "" ("State(s) in Front (\"\")")] -> w515
          tunnel: [w529 w550] -> w512
          tunnel: w513 -> [w528 _]
          frame False {
            n268 = local read "Path"() -> (w530:path)
            n269 = call "ResultSavePrompt.vi"("Path"=w530) -> ("selected path"=w534:path, "cancel?"=w533:bool)
            n270 = case shown="False" w533 {
              tunnel: w532 -> [w547 _]
              tunnel: w535 -> [w546 w548]
              tunnel: w534 -> [w545 _]
              tunnel: ["UI: Recent Menu Update" ("State(s) in Front (\"\")") "" ("State(s) in Front (\"\")")] -> w531
              tunnel: w530 -> [w543 _]
              tunnel: [w539 w548] -> w529
              tunnel: w528 -> [w538 _]
              frame False {
                w537 = ";" ("delimiter (\\t)")
                n271 = call-poly <vilib>:"Write Delimited Spreadsheet.vi"("file path (dialog if empty)"=w545, "2D data"=w547, "error in (no error)"=w546, "delimiter (\\t)"=w537) -> ("error out"=w540:errorcluster)  [unwired: 10 in, 1 out]
                n272 = Build Path(base path=w543, name or relative path=path "Data.TCE") -> (appended path=w541:path)
                n273 = call-poly <vilib>:"Write Delimited Spreadsheet.vi"("file path (dialog if empty)"=w541, "2D data"=w538, "error in (no error)"=w540, "delimiter (\\t)"=w537) -> ("new file path (Not A Path if cancelled)"=w536:path, "error out"=w539:errorcluster)  [unwired: 10 in]
                n274 = call "RunTimeMenu_TCE_RecentInsert.vi"("NewPath"=w536) -> ()  [unwired: 11 in]
              }
              frame True {
              }
            }
          }
          frame True {
          }
        }
        n275 = case shown="Error .." w512 {
          frame No Error {
          }
          frame Error {
            n276 = One Button Dialog(message="File Save Error!\nClose file if open.") -> ()  [unwired: 1 in, 1 out]
          }
        }
        n277 = call <vilib>:"Add State(s) to Queue__jki_lib_state_machine.vi"("State(s) in Front (\"\")"=w515, "State(s) in (\"\")"=w526) -> ("States Out"=w525:string)  [unwired: 13 in]
      }
      frame "---------- UI ----------" {
        # "Do not put any code in this frame.\n(It is a separator no-op. You can make a copy of this frame to create a new UI frame)"
        n278 = call <vilib>:"Add State(s) to Queue__jki_lib_state_machine.vi"("State(s) in (\"\")"=w555) -> ("States Out"=w554:string)  [unwired: 14 in]
      }
      frame "UI: Initialize" {
        w564 = FALSE ("Visible")
        w575 = T13 4 items=["Grayscale (U8)", "Grayscale (I16)", "Grayscale (SGL)", "Complex (CSG)", "RGB (U32)", "HSL (U32)", "RGB (U64)", "Grayscale (U16)"] ("Image Type")
        w556 = FALSE ("Visible")
        w563 = TRUE ("Zoom to Fit Mode")
        w560 = 0.0 ("X Scale.Range:Minimum")
        w562 = dbl[] []
        w559 = 0.0 ("Cursor.Cursor Position:Cursor X")
        w561 = dbl[][] []
        # "Initialize the User Interface, here.\n(this is called automatically, by the Macro: Init)"
        n279 = property on="Temps grads" class="WFGraph (strict)"("Visible"=w564) -> ()  [unwired: 2 in, 2 out]
        n280 = property on="Temps single grad" class="WFGraph (strict)"("Visible"=w564) -> ()  [unwired: 2 in, 2 out]
        n281 = control-ref of="Splitter 4"() -> (w566:refnum<vi>)
        n282 = local write "Offset Applied?"(FALSE ("Offset Applied?")) -> ()
        n283 = property on="FrozenFractionGraph" class="WFGraph (strict)"("Active Plot"=u32 0, "Legend Visible"=FALSE ("Legend:Visible")) -> ()  [unwired: 2 in, 2 out]
        n284 = property on="Image" class="ImageControl"("Zoom to Fit Mode"=w563) -> ()  [unwired: 2 in, 2 out]
        n285 = property on="FrozenFractionGraph" class="WFGraph (strict)"("Visible"=w563) -> ()  [unwired: 2 in, 2 out]
        n286 = property on="Temps" class="WFGraph (strict)"("XScale.Minimum"=w560) -> ()  [unwired: 2 in, 2 out]
        n287 = property on="FrozenFractionGraph" class="WFGraph (strict)"("XScale.Minimum"=w560) -> ()  [unwired: 2 in, 2 out]
        n288 = call "ShowHideSplit.vi"("Splitter in"=w566, "Show Split"=w556) -> ()  [unwired: 1 in]
        n289 = property on="Contents" class="Str"("Visible"=w556) -> ()  [unwired: 2 in, 2 out]
        n290 = property on="Calc_All" class="Bool"("Visible"=w556) -> ()  [unwired: 2 in, 2 out]
        n291 = property on="CurTemp" class="DigNum (strict)"("Visible"=FALSE) -> ()  [unwired: 2 in, 2 out]
        n292 = property on="Fraction Single" class="WFGraph (strict)"("Visible"=w556) -> ()  [unwired: 2 in, 2 out]
        n293 = call <vilib>:"Application Directory.vi"() -> ("Application Directory"=w579:path)
        n294 = property on="Well" class="Str"("Visible"=w556) -> ()  [unwired: 2 in, 2 out]
        n295 = call "Read Exe Version.vi"("Application name"=path "TCE.exe") -> ("FileVersion"=w571:string)  [unwired: 7 in, 3 out]
        n296 = Path To String(path=w579) -> (string=w581:string)
        n297 = Concatenate Strings("version " ("string"), w571) -> (→"version":string)
        n298 = property on="Remove_Correction" class="Bool"("Visible"=w556) -> ()  [unwired: 2 in, 2 out]
        n299 = property on="Correct Data" class="Bool"("Visible"=w556) -> ()  [unwired: 2 in, 2 out]
        n300 = call "IMAQ Create"("Image Name"="placeholder_img_TCE", "Image Type"=w575) -> ("New Image"=w578:T1)  [unwired: 3 in, 1 out]
        n301 = Concatenate Strings(w581, "\\camera_placeholder.png") -> (w580:string)
        n302 = String To Path(string=w580) -> (path=w582:path)
        n303 = call "IMAQ ReadFile 2"("Use File Path Image Type"=FALSE, "File Path"=w582, "Image"=w578) -> ("Image Out"=w573:T1)  [unwired: 4 in, 4 out]
        "placeholder image" <- w573
        n304 = local write "FrozenFractionGraph"(w561) -> ()
        n305 = local write "Temps"(w561) -> ()
        n306 = local write "Temps single grad"(w562) -> ()
        n307 = local write "Temps grads"(w561) -> ()
        n308 = local write "Image"(w573) -> ()
        n309 = local write "Path"(path "" ("Path")) -> ()
        n310 = local write "Temps single"(w562) -> ()
        n311 = property on="Temps single" class="WFGraph (strict)"("Cursor.Cursor X"=w559) -> ()  [unwired: 2 in, 2 out]
        n312 = property on="Temps" class="WFGraph (strict)"("Cursor.Cursor X"=w559) -> ()  [unwired: 2 in, 2 out]
        n313 = property on="Temps grads" class="WFGraph (strict)"("Cursor.Cursor X"=w559) -> ()  [unwired: 2 in, 2 out]
        n314 = property on="Temps single grad" class="WFGraph (strict)"("Cursor.Cursor X"=w559) -> ()  [unwired: 2 in, 2 out]
        n315 = property on="FrozenFractionGraph" class="WFGraph (strict)"("Cursor.Cursor X"=w559) -> ()  [unwired: 2 in, 2 out]
        n316 = call <vilib>:"Add State(s) to Queue__jki_lib_state_machine.vi"("State(s) in Front (\"\")"="UI: Tutorial\nUI: Recent Menu Update\nUI: Progress >> Hide\nUI: Menu Save >> Hide\nUI: Menu Overlay Grid >> Hide\nUI: Menu Overlay Temps >> Hide" ("State(s) in Front (\"\")"), "State(s) in (\"\")"=w590) -> ("States Out"=w589:string)  [unwired: 13 in]
        "img" <- 0
        "Title" <- "Thermal Camera Evaluation" ("Title")
        "Title 2" <- "Well Data" ("Title 2")
      }
      frame "UI: Progress" {
        # "Initialize the User Interface, here.\n(this is called automatically, by the Macro: Init)"
        n317 = case shown="\"Hide\", Default" w594 {
          tunnel: [FALSE ("Visible") TRUE ("Visible")] -> w593
          frame "Hide", Default {
          }
          frame "Show" {
          }
        }
        n318 = local write "img"(0 ("img")) -> ()
        n319 = local write "Slide"(u8 0 ("Slide")) -> ()
        n320 = property on="Slide" class="Slide (strict)"("Visible"=w593) -> ()  [unwired: 2 in, 2 out]
        n321 = call <vilib>:"Add State(s) to Queue__jki_lib_state_machine.vi"("State(s) in (\"\")"=w598) -> ("States Out"=w597:string)  [unwired: 14 in]
      }
      frame "UI: Recent Menu Update" {
        # "Initialize the User Interface, here.\n(this is called automatically, by the Macro: Init)"
        n322 = Current VI's Menubar() -> (w602:refnum<k9>)
        n323 = call "RunTimeMenu_Initialize_TCE.vi"("Menu in"=w602) -> ("paths"=→"recentPaths":path[])  [unwired: 9 in, 1 out]
        n324 = call <vilib>:"Add State(s) to Queue__jki_lib_state_machine.vi"("State(s) in (\"\")"=w606) -> ("States Out"=w605:string)  [unwired: 14 in]
      }
      frame "UI: Show First Image" {
        w607 = 0.0 ("Cursor.Cursor Position:Cursor X")
        # "Initialize the User Interface, here.\n(this is called automatically, by the Macro: Init)"
        n325 = Unbundle By Name(w610) -> ("img_array"=w609:T1[])
        n326 = property on="Temps" class="WFGraph (strict)"("Cursor.Cursor X"=w607) -> ()  [unwired: 2 in, 2 out]
        n327 = property on="Temps grads" class="WFGraph (strict)"("Cursor.Cursor X"=w607) -> ()  [unwired: 2 in, 2 out]
        n328 = property on="Temps single grad" class="WFGraph (strict)"("Cursor.Cursor X"=w607) -> ()  [unwired: 2 in, 2 out]
        n329 = property on="Temps single" class="WFGraph (strict)"("Cursor.Cursor X"=w607) -> ()  [unwired: 2 in, 2 out]
        n330 = property on="FrozenFractionGraph" class="WFGraph (strict)"("Cursor.Cursor X"=w607) -> ()  [unwired: 2 in, 2 out]
        n331 = property on="Fraction Single" class="WFGraph (strict)"("Cursor.Cursor X"=w607) -> ()  [unwired: 2 in, 2 out]
        n332 = Index Array(array=w609) -> (element=w608:T1)  [unwired: 1 in]
        n333 = local write "Image"(w608) -> ()
        n334 = call <vilib>:"Add State(s) to Queue__jki_lib_state_machine.vi"("State(s) in (\"\")"=w613) -> ("States Out"=w612:string)  [unwired: 14 in]
      }
      frame "UI: Tutorial" {
        # "Initialize the User Interface, here.\n(this is called automatically, by the Macro: Init)"
        n335 = call <vilib>:"Add State(s) to Queue__jki_lib_state_machine.vi"("State(s) in (\"\")"=w618) -> ("States Out"=w617:string)  [unwired: 14 in]
        "Tutorial" <- w614
      }
      frame "UI: Calc" {
        # "Initialize the User Interface, here.\n(this is called automatically, by the Macro: Init)"
        n336 = case shown="\"Hidden\", \"Hide\"" w621 {
          tunnel: [T8."Disabled and Grayed Out" ("Disabled") T8."Disabled and Grayed Out" ("Disabled") T8."Enabled" ("Disabled")] -> w620
          tunnel: [TRUE FALSE TRUE] -> w619
          frame "Disable", "False", Default {
          }
          frame "Hidden", "Hide" {
          }
          frame "True" {
          }
        }
        n337 = property on="Calc_All" class="Bool"("DisabledEnum"=w620) -> ()  [unwired: 2 in, 2 out]
        n338 = property on="Calc_All" class="Bool"("Visible"=w619) -> ()  [unwired: 2 in, 2 out]
        n339 = call <vilib>:"Add State(s) to Queue__jki_lib_state_machine.vi"("State(s) in (\"\")"=w625) -> ("States Out"=w624:string)  [unwired: 14 in]
      }
      frame "UI: Cursor Set" {
        # "Argument"
        # "Set and Unset Cursor Busy.\n(Usage: \"UI: Cursor Set >> Busy|Idle\")"
        n340 = case shown="\"Busy\"" w632 {
          tunnel: w634 -> [w639 w641]
          tunnel: [w638 w640] -> w633
          frame "Idle", Default {
            n341 = call <vilib>:"Unset Busy.vi"("error in (no error)"=w639) -> ("error out"=w638:errorcluster)  [unwired: 10 in]
          }
          frame "Busy" {
            n342 = call <vilib>:"Set Busy.vi"("error in (no error)"=w641) -> ("error out"=w640:errorcluster)  [unwired: 9 in, 1 out]
          }
        }
        n343 = call <vilib>:"Add State(s) to Queue__jki_lib_state_machine.vi"("State(s) in (\"\")"=w637) -> ("States Out"=w636:string)  [unwired: 14 in]
      }
      frame "UI: Menu Save" {
        # "Argument"
        # "Set and Unset Cursor Busy.\n(Usage: \"UI: Cursor Set >> Busy|Idle\")"
        n344 = case shown="\"Disable\", \"False\", Default" w645 {
          tunnel: [FALSE TRUE] -> w643
          frame "Disable", "False", Default {
          }
          frame "Active", "Show", "True" {
          }
        }
        n345 = Current VI's Menubar() -> (w644:refnum<k9>)
        n346 = call "RunTimeMenu_Save_State_TCE.vi"("enabled"=w643, "item tag"=string[] ["DATA_SAVE", "DATA_SAVE_AS"], "Menu in"=w644) -> ()  [unwired: 8 in, 1 out]
        n347 = call <vilib>:"Add State(s) to Queue__jki_lib_state_machine.vi"("State(s) in (\"\")"=w649) -> ("States Out"=w648:string)  [unwired: 14 in]
      }
      frame "UI: Menu Overlay Grid" {
        # "Argument"
        # "Set and Unset Cursor Busy.\n(Usage: \"UI: Cursor Set >> Busy|Idle\")"
        n348 = case shown="\"Disable\", \"False\", Default" w655 {
          tunnel: [FALSE TRUE] -> w653
          frame "Disable", "False", Default {
          }
          frame "Active", "Show", "True" {
          }
        }
        n349 = Current VI's Menubar() -> (w654:refnum<k9>)
        n350 = call "RunTimeMenu_Save_State_TCE.vi"("enabled"=w653, "item tag"=string[] ["OVERLAY_GRID", "OVERLAY_CLEAR"], "Menu in"=w654) -> ()  [unwired: 8 in, 1 out]
        n351 = call <vilib>:"Add State(s) to Queue__jki_lib_state_machine.vi"("State(s) in (\"\")"=w659) -> ("States Out"=w658:string)  [unwired: 14 in]
      }
      frame "UI: Menu Overlay Temps" {
        # "Argument"
        # "Set and Unset Cursor Busy.\n(Usage: \"UI: Cursor Set >> Busy|Idle\")"
        n352 = case shown="\"Disable\", \"False\", Default" w665 {
          tunnel: [FALSE TRUE] -> w663
          frame "Disable", "False", Default {
          }
          frame "Active", "Show", "True" {
          }
        }
        n353 = Current VI's Menubar() -> (w664:refnum<k9>)
        n354 = call "RunTimeMenu_Save_State_TCE.vi"("enabled"=w663, "item tag"=string[] ["OVERLAY_TEMPS", "OVERLAY_FREEZE"], "Menu in"=w664) -> ()  [unwired: 8 in, 1 out]
        n355 = call <vilib>:"Add State(s) to Queue__jki_lib_state_machine.vi"("State(s) in (\"\")"=w669) -> ("States Out"=w668:string)  [unwired: 14 in]
      }
      frame "UI: Single Temps" {
        # "Argument"
        # "Set and Unset Cursor Busy.\n(Usage: \"UI: Cursor Set >> Busy|Idle\")"
        n356 = control-ref of="Splitter 4"() -> (w680:refnum<vi>)
        n357 = Unbundle By Name(w678) -> ("ShowGradient"=w677:bool)
        n358 = case shown="\"Disable\", \"False\", Default" w681 {
          tunnel: [w691 w694] -> w674
          tunnel: w680 -> [w692 w693]
          frame "Disable", "False", Default {
            w691 = FALSE
            n359 = call "ShowHideSplit.vi"("Splitter in"=w692, "Show Split"=w691) -> ()  [unwired: 1 in]
          }
          frame "Active", "Show", "True" {
            w694 = TRUE
            n360 = call "ShowHideSplit.vi"("Splitter in"=w693, "Show Split"=w694) -> ()  [unwired: 1 in]
          }
        }
        n361 = case shown="False" w677 {
          tunnel: [w687 w690] -> w676
          tunnel: [w686 w690] -> w675
          tunnel: [w685 w689] -> w673
          tunnel: w674 -> [w687 w689]
          tunnel: [w685 w688] -> w672
          frame False {
            w685 = FALSE
            n362 = Not(x=w687) -> (.not. x?=w686:bool)
          }
          frame True {
            w690 = FALSE
            n363 = Not(x=w689) -> (.not. x?=w688:bool)
          }
        }
        n364 = Not(x=w674) -> (.not. x?=w679:bool)
        n365 = property on="Temps single" class="WFGraph (strict)"("Visible"=w674) -> ()  [unwired: 2 in, 2 out]
        n366 = property on="Temps" class="WFGraph (strict)"("Visible"=w679) -> ()  [unwired: 2 in, 2 out]
        n367 = property on="Fraction Single" class="WFGraph (strict)"("Visible"=w676) -> ()  [unwired: 2 in, 2 out]
        n368 = property on="FrozenFractionGraph" class="WFGraph (strict)"("Visible"=w675) -> ()  [unwired: 2 in, 2 out]
        n369 = property on="Temps grads" class="WFGraph (strict)"("Visible"=w672) -> ()  [unwired: 2 in, 2 out]
        n370 = property on="Temps single grad" class="WFGraph (strict)"("Visible"=w673) -> ()  [unwired: 2 in, 2 out]
        n371 = property on="CurTemp" class="DigNum (strict)"("Visible"=w674) -> ()  [unwired: 2 in, 2 out]
        n372 = property on="Contents" class="Str"("Visible"=w674) -> ()  [unwired: 2 in, 2 out]
        n373 = property on="Well" class="Str"("Visible"=w674) -> ()  [unwired: 2 in, 2 out]
        n374 = call <vilib>:"Add State(s) to Queue__jki_lib_state_machine.vi"("State(s) in (\"\")"=w684) -> ("States Out"=w683:string)  [unwired: 14 in]
      }
      frame "UI: Front Panel State" {
        # "Argument"
        # "Set Front Panel Open or Closed\n(Usage: \"UI: Front Panel State >> Open|Close\")"
        n375 = Unbundle By Name(w697) -> ("Core.Current VI Reference"=w696:refnum<vi>)
        n376 = case shown="\"Open\", \"Standard\", Default" w695 {
          tunnel: w699 -> [w707 w722 w733 w746 w759]
          tunnel: [w709 w723 w735 w748 w761] -> w698
          tunnel: w696 -> [w708 w720 w734 w747 w760]
          frame "Open", "Standard", Default {
            w702 = T5."Standard" ("State")
            n377 = property class="VI"(reference=w708, error in=w707) -> (reference out=w705:refnum<vi>, error out=w706:errorcluster, "FP.State"=w704:T5)
            n378 = Not Equal?(x=w704, y=w702) -> (x != y?=w703:bool)
            n379 = case shown="False" w703 {
              tunnel: [w713 w715] -> w709
              tunnel: w706 -> [w712 w715]
              tunnel: w705 -> [w711 _]
              tunnel: w702 -> [w710 _]
              frame True {
                n380 = invoke class="VI" method="FP.Open"(reference=w711, error in=w712, "Activate"=TRUE, "State"=w710) -> (error out=w713:errorcluster)  [unwired: 1 in, 4 out]
              }
              frame False {
              }
            }
          }
          frame "Close", "Closed" {
            n381 = property class="VI"(reference=w720, error in=w722) -> (reference out=w719:refnum<vi>, error out=w721:errorcluster, "FP.State"=w717:T5)
            n382 = Not Equal?(x=w717, y=T5."Closed" ("Front Panel Window:State")) -> (x != y?=w716:bool)
            n383 = case shown="True" w716 {
              tunnel: [w724 w727] -> w723
              tunnel: w721 -> [w724 w726]
              tunnel: w719 -> [_ w725]
              frame False {
              }
              frame True {
                n384 = invoke class="VI" method="FP.Close"(reference=w725, error in=w726) -> (error out=w727:errorcluster)  [unwired: 1 in, 2 out]
              }
            }
          }
          frame "Hidden", "Hide" {
            w728 = T5."Hidden" ("State")
            n385 = property class="VI"(reference=w734, error in=w733) -> (reference out=w731:refnum<vi>, error out=w732:errorcluster, "FP.State"=w730:T5)
            n386 = Not Equal?(x=w730, y=w728) -> (x != y?=w729:bool)
            n387 = case shown="True" w729 {
              tunnel: [w739 w740] -> w735
              tunnel: w732 -> [w738 w740]
              tunnel: w731 -> [w737 _]
              tunnel: w728 -> [w736 _]
              frame True {
                n388 = invoke class="VI" method="FP.Open"(reference=w737, error in=w738, "State"=w736) -> (error out=w739:errorcluster)  [unwired: 2 in, 4 out]
              }
              frame False {
              }
            }
          }
          frame "Minimize", "Minimized" {
            w741 = T5."Minimized" ("State")
            n389 = property class="VI"(reference=w747, error in=w746) -> (reference out=w744:refnum<vi>, error out=w745:errorcluster, "FP.State"=w743:T5)
            n390 = Not Equal?(x=w743, y=w741) -> (x != y?=w742:bool)
            n391 = case shown="True" w742 {
              tunnel: [w752 w753] -> w748
              tunnel: w745 -> [w751 w753]
              tunnel: w744 -> [w750 _]
              tunnel: w741 -> [w749 _]
              frame True {
                n392 = invoke class="VI" method="FP.Open"(reference=w750, error in=w751, "State"=w749) -> (error out=w752:errorcluster)  [unwired: 2 in, 4 out]
              }
              frame False {
              }
            }
          }
          frame "Maximize", "Maximized" {
            w754 = T5."Maximized" ("State")
            n393 = property class="VI"(reference=w760, error in=w759) -> (reference out=w757:refnum<vi>, error out=w758:errorcluster, "FP.State"=w756:T5)
            n394 = Not Equal?(x=w756, y=w754) -> (x != y?=w755:bool)
            n395 = case shown="True" w755 {
              tunnel: [w765 w766] -> w761
              tunnel: w758 -> [w764 w766]
              tunnel: w757 -> [w763 _]
              tunnel: w754 -> [w762 _]
              frame True {
                n396 = invoke class="VI" method="FP.Open"(reference=w763, error in=w764, "State"=w762) -> (error out=w765:errorcluster)  [unwired: 2 in, 4 out]
              }
              frame False {
              }
            }
          }
        }
        n397 = call <vilib>:"Add State(s) to Queue__jki_lib_state_machine.vi"("State(s) in (\"\")"=w701) -> ("States Out"=w700:string)  [unwired: 14 in]
      }
      frame "---------- Macro ----------" {
        # "Do not put any code in this frame.\n(It is a separator no-op. You can make a copy of this frame to create a new Macro frame)"
        n398 = call <vilib>:"Add State(s) to Queue__jki_lib_state_machine.vi"("State(s) in (\"\")"=w770) -> ("States Out"=w769:string)  [unwired: 14 in]
      }
      frame "Macro: Initialize" {
        w771 = "// UI: Cursor Set >> Busy\nData: Initialize\nInitialize Core Data\nUI: Initialize\nUI: Front Panel State >> Show\nUI: Tutorial >> Load Image\n// Image: Draw\n// UI: Cursor Set >> Idle"  # // UI: Cursor Set >> Busy Data: Initialize Initialize Core Data UI: Initialize UI: Front Panel State >> Show UI: Tutorial >> Load Image // Image: Draw // UI: Cursor Set >> Idle
        # "Initialization Macro\n(This is called once, when the VI starts)"
        n399 = call <vilib>:"Add State(s) to Queue__jki_lib_state_machine.vi"("State(s) in Front (\"\")"=w771, "State(s) in (\"\")"=w775) -> ("States Out"=w774:string)  [unwired: 13 in]
      }
      frame "Macro: Exit" {
        # "Exit Macro\n(This is called once, when the VI exits)"
        n400 = Unbundle By Name(w782) -> ("Core.Close Panel on Exit?"=w781:bool)
        n401 = Select(t="UI: Front Panel State >> Close", s=w781, f="") -> (s? t:f=w778:string)
        n402 = call <vilib>:"Add State(s) to Queue__jki_lib_state_machine.vi"("State(s) in (\"\")"=w778, "State(s) at Back (\"\")"="Data: Cleanup\nExit") -> ("States Out"=w776:string)  [unwired: 13 in]
        n403 = call <vilib>:"Add State(s) to Queue__jki_lib_state_machine.vi"("State(s) in Front (\"\")"=w776, "State(s) in (\"\")"=w785) -> ("States Out"=w784:string)  [unwired: 13 in]
      }
      frame "---------- Process ----------" {
        # "Template Separator\n(You can make a copy of, or modify, this frame)"
        n404 = call <vilib>:"Add State(s) to Queue__jki_lib_state_machine.vi"("State(s) in (\"\")"=w789) -> ("States Out"=w788:string)  [unwired: 14 in]
      }
      frame "Process: Calculate All" {
        # "Template Separator\n(You can make a copy of, or modify, this frame)"
        n405 = call <vilib>:"Add State(s) to Queue__jki_lib_state_machine.vi"("State(s) in Front (\"\")"="Data: Temps Clear\nData: Set Image\nUI: Cursor Set >> Busy\nUI: Progress >> Show\nProcess: Calculate All Temps\nProcess: Calculate Gradients\nProcess: Calculate Freezing Points\nProcess: Calculate Offset\nProcess: Calculate Melt Temp\nProcess: Calculate Freeze Fraction\nUI: Progress >> Hide\nUI: Cursor Set >> Idle\nUI: Tutorial >> Click on a Well to show single or click outside the plate to show all." ("State(s) in Front (\"\")"), "State(s) in (\"\")"=w794) -> ("States Out"=w793:string)  [unwired: 13 in]
      }
      frame "Process: Recalculate" {
        # "Template Separator\n(You can make a copy of, or modify, this frame)"
        n406 = call <vilib>:"Add State(s) to Queue__jki_lib_state_machine.vi"("State(s) in Front (\"\")"="Process: Calculate Gradients\nProcess: Calculate Freezing Points\nProcess: Calculate Melt Temp\nProcess: Calculate Freeze Fraction" ("State(s) in Front (\"\")"), "State(s) in (\"\")"=w799) -> ("States Out"=w798:string)  [unwired: 13 in]
      }
      frame "Process: Calculate Temps" {
        # "Your code here.\n(You can make a copy of, or modify, this frame)"
        n407 = Unbundle By Name(w805) -> ("Image Out"=w803:T1, "Points.Pixels"=w802:cluster{"X":i32, "Y":i32}[][], "Points.Top Left.X"=w813:sgl, "Points.Top Right.X"=w812:sgl, "Points.Bottom Left.X"=w811:sgl, "Points.Bottom Right.X"=w810:sgl)
        n408 = Equal To 0?(x=w813) -> (x = 0?=w809:bool)
        n409 = Equal To 0?(x=w812) -> (x = 0?=w808:bool)
        n410 = Equal To 0?(x=w811) -> (x = 0?=w807:bool)
        n411 = Equal To 0?(x=w810) -> (x = 0?=w806:bool)
        n412 = local read "Points"() -> (w801:T2[])
        n413 = Compound Arithmetic op=OR(w809, w808, w807, w806) -> (w804:bool)
        n414 = case shown="False" w804 {
          tunnel: w803 -> [w819 w820]
          tunnel: w802 -> [w818 _]
          tunnel: w801 -> [_ _]
          tunnel: [w817 w820] -> w800
          frame False {
            n415 = call "TCam_WellTemp.vi"("Pixels"=w818, "Image in"=w819) -> ("Image Out"=w817:T1)  [unwired: 5 in, 4 out]
          }
          frame True {
          }
        }
        n416 = local write "Image"(w800) -> ()
        n417 = call <vilib>:"Add State(s) to Queue__jki_lib_state_machine.vi"("State(s) in (\"\")"=w816) -> ("States Out"=w815:string)  [unwired: 14 in]
      }
      frame "Process: Calculate Well" {
        # "Your code here.\n(You can make a copy of, or modify, this frame)"
        n418 = Unbundle By Name(w822) -> ("Image Out"=w827:T1, "Points.Pixels"=w826:cluster{"X":i32, "Y":i32}[][], "Points.Top Left.X"=w835:sgl, "Points.Top Right.X"=w834:sgl, "Points.Bottom Left.X"=w833:sgl, "Points.Bottom Right.X"=w832:sgl)
        n419 = local read "Points"() -> (w825:T2[])
        n420 = Equal To 0?(x=w835) -> (x = 0?=w831:bool)
        n421 = Equal To 0?(x=w834) -> (x = 0?=w830:bool)
        n422 = Equal To 0?(x=w833) -> (x = 0?=w829:bool)
        n423 = Equal To 0?(x=w832) -> (x = 0?=w828:bool)
        n424 = Compound Arithmetic op=OR(w831, w830, w829, w828) -> (w824:bool)
        n425 = case shown="False" w824 {
          tunnel: w827 -> [w860 _]
          tunnel: w826 -> [w859 _]
          tunnel: w825 -> [w858 _]
          tunnel: [w853 _] -> w823
          tunnel: w822 -> [w846 _]
          tunnel: w822 -> [w844 w865]
          tunnel: [w843 w865] -> w821
          frame False {
            n426 = local read "ImageIdx"() -> (w840:u32)
            n427 = property on="ImageIdx" class="Slide (strict)"() -> ("Scale.Maximum"=w848:dbl)  [unwired: 2 in, 2 out]
            n428 = call "TCam_WellCalculater.vi"("DrawTempOverlay"=TRUE, "Well Pos"=w858, "Pixels"=w859, "Image in"=w860, "index"="Well") -> ("Image Out"=w857:T1, "mean"=w842:dbl)  [unwired: 4 in, 1 out]
            n429 = Increment(x=w840) -> (x+1=w854:u32)
            n430 = local write "Image"(w857) -> ()
            n431 = Greater?(x=w854, y=w848) -> (0:w856:bool)
            n432 = case shown="False" w856 {
              tunnel: w854 -> [_ w864]
              tunnel: [w863 w864] -> w855
              tunnel: w854 -> [w863 _]
              tunnel: ["Data: Set Image\nProcess: Calculate Well" ("State(s) in Front (\"\")") _] -> w853
              tunnel: [TRUE _] -> w852
              frame False {
              }
              frame True {
              }
            }
            n433 = Unbundle By Name(w846) -> ("Temps"=w845:dbl[])
            n434 = Divide(x=w840, y=w848) -> (x/y=w851:dbl)
            n435 = property on="Temps single" class="WFGraph (strict)"("Cursor.Cursor X"=w840) -> ()  [unwired: 2 in, 2 out]
            n436 = Multiply(x=w851, y=100.0) -> (x*y=w849:dbl)
            n437 = Build Array (concatenate)(w845, w842) -> (w841:dbl[])
            "Temps single" <- w841
            n438 = local write "Slide"(w849) -> ()
            n439 = Bundle By Name(cluster=w844, "Temps"=w841) -> (w843:T4)
            n440 = local write "ImageIdx"(w855) -> ()
            n441 = property on="Slide" class="Slide (strict)"("Visible"=w852) -> ()  [unwired: 2 in, 2 out]
          }
          frame True {
          }
        }
        n442 = call <vilib>:"Add State(s) to Queue__jki_lib_state_machine.vi"("State(s) in Front (\"\")"=w823, "State(s) in (\"\")"=w838) -> ("States Out"=w837:string)  [unwired: 13 in]
      }
      frame "Process: Calculate All Temps" {
        # "Your code here.\n(You can make a copy of, or modify, this frame)"
        n443 = Unbundle By Name(w871) -> ("img_array"=w874:T1[], "Points.Pixels"=w873:cluster{"X":i32, "Y":i32}[][], "Points.Top Left.X"=w882:sgl, "Points.Top Right.X"=w881:sgl, "Points.Bottom Left.X"=w880:sgl, "Points.Bottom Right.X"=w879:sgl, "Save Well data"=w866:bool)
        n444 = local read "Path"() -> (w868:path)
        n445 = Equal To 0?(x=w882) -> (x = 0?=w878:bool)
        n446 = Equal To 0?(x=w881) -> (x = 0?=w877:bool)
        n447 = Equal To 0?(x=w880) -> (x = 0?=w876:bool)
        n448 = Equal To 0?(x=w879) -> (x = 0?=w875:bool)
        n449 = Compound Arithmetic op=OR(w878, w877, w876, w875) -> (w872:bool)
        n450 = case shown="False" w872 {
          tunnel: w874 -> [w902 _]
          tunnel: w873 -> [w904 _]
          tunnel: [TRUE ("Visible") w948] -> w870
          tunnel: [w900 dbl[][] []] -> w869
          tunnel: w868 -> [w890 _]
          tunnel: [w889 w948] -> w867
          tunnel: w866 -> [w889 _]
          frame False {
            n451 = for {
              N -> [w934]
              tunnel: w902 -> [w945] mode=indexing
              tunnel: w904 -> [w944]
              tunnel: [w943] -> w903 mode=indexing
              workers-P: _ -> [_]
              tunnel: [w930] -> w895 mode=indexing
              tunnel: [w929] -> w899 mode=indexing
              tunnel: [w928] -> w894 mode=indexing
              tunnel: [w927] -> w898 mode=indexing
              tunnel: [w926] -> w893 mode=indexing
              tunnel: [w925] -> w897 mode=indexing
              tunnel: [w924] -> w892 mode=indexing
              tunnel: [w923] -> w896 mode=indexing
              tunnel: [w922] -> w891
              i -> [w932]
              n452 = call "TCam_WellTemp.vi"("Pixels"=w944, "Image in"=w945) -> ("Temps"=w943:dbl[], "Output cluster"=w931:T15)  [unwired: 5 in, 3 out]
              n453 = Unbundle By Name(w931) -> ("Mean of Pixels from Well x1"=w930:dbl, "Pixel for well x1 each picture"=w929:dbl[], "Mean of Pixels from Well x2"=w928:dbl, "Pixel for well x2 each picture"=w927:dbl[], "Mean of Pixels from Well x3"=w926:dbl, "Pixel for well x3 each picture"=w925:dbl[], "Mean of Pixels from Well x4"=w924:dbl, "Pixel for well x4 each picture"=w923:dbl[], "Pixel Number"=w922:i32)
              n454 = property on="ImageIdx" class="Slide (strict)"() -> ("Scale.Maximum"=w940:dbl)  [unwired: 2 in, 2 out]
              n455 = local read "img"() -> (w942:i32)
              n456 = property on="Temps" class="WFGraph (strict)"("Cursor.Cursor X"=w932) -> ()  [unwired: 2 in, 2 out]
              n457 = Increment(x=w942) -> (x+1=w933:i32)
              n458 = Divide(x=w933, y=w940) -> (x/y=w947:dbl)
              n459 = local write "img"(w933) -> ()
              n460 = Format Into String(w933) -> (resulting string=w939:string)  [unwired: 3 in, 1 out]
              n461 = Multiply(x=w947, y=100.0) -> (x*y=w941:dbl)
              n462 = property on="Temps grads" class="WFGraph (strict)"("Cursor.Cursor X"=w932) -> ()  [unwired: 2 in, 2 out]
              n463 = Format Into String(w934) -> (resulting string=w935:string)  [unwired: 3 in, 1 out]
              n464 = local write "Slide"(w941) -> ()
              n465 = Concatenate Strings("Processing image " ("Tutorial"), w939, " of " ("Tutorial"), w935) -> (w938:string)
              n466 = property on="FrozenFractionGraph" class="WFGraph (strict)"("Cursor.Cursor X"=w932) -> ()  [unwired: 2 in, 2 out]
              n467 = local write "Tutorial"(w938) -> ()
            }
            n468 = case shown="True" w889 {
              tunnel: w899 -> [_ w921]
              tunnel: w898 -> [_ w920]
              tunnel: w897 -> [_ w919]
              tunnel: w896 -> [_ w918]
              tunnel: w895 -> [_ w917]
              tunnel: w894 -> [_ w915]
              tunnel: w893 -> [_ w913]
              tunnel: w892 -> [_ w911]
              tunnel: w891 -> [_ w907]
              tunnel: w890 -> [_ w905]
              frame False {
              }
              frame True {
                # "Save Well data for validation"
                n469 = Transpose 2D Array(2D array=w921) -> (transposed array=w916:dbl[][])
                n470 = Transpose 2D Array(2D array=w920) -> (transposed array=w914:dbl[][])
                n471 = Transpose 2D Array(2D array=w919) -> (transposed array=w912:dbl[][])
                n472 = Transpose 2D Array(2D array=w918) -> (transposed array=w910:dbl[][])
                n473 = Build Array (concatenate)(w917, w916, w915, w914, w913, w912, w911, w910) -> (w909:dbl[][])
                n474 = Transpose 2D Array(2D array=w909) -> (transposed array=w908:dbl[][])
                n475 = call "Save Extra data.vi"("Temps"=w908, "Pixel Num."=w907, "Save data Title"=T9."Pixel Values Wells", "name or relative path"=w905) -> ()  [unwired: 2 in]
              }
            }
            n476 = Transpose 2D Array(2D array=w903) -> (transposed array=w900:dbl[][])
          }
          frame True {
            w948 = FALSE ("Visible")
          }
        }
        "Temps" <- w869
        n477 = property on="Correct Data" class="Bool"("Visible"=w870) -> ()  [unwired: 2 in, 2 out]
        n478 = case shown="True" w867 {
          tunnel: w869 -> [_ w887]
          tunnel: w868 -> [_ w886]
          frame False {
          }
          frame True {
            # "Save extra data for validation"
            n479 = call "Save Extra data.vi"("Temps"=w887, "Save data Title"=T9."All Wells Mean", "name or relative path"=w886) -> ()  [unwired: 3 in]
          }
        }
        n480 = call <vilib>:"Add State(s) to Queue__jki_lib_state_machine.vi"("State(s) in (\"\")"=w885) -> ("States Out"=w884:string)  [unwired: 14 in]
      }
      frame "Process: Calculate Gradients" {
        # "Your code here.\n(You can make a copy of, or modify, this frame)"
        n481 = local read "Temps"() -> (w951:dbl[][])
        n482 = for {
          tunnel: w951 -> [w960] mode=indexing
          workers-P: _ -> [_]
          tunnel: [w956] -> w950 mode=indexing
          n483 = Array Size(array=w960) -> (size(s)=w959:i32)
          n484 = Decrement(x=w959) -> (x-1=w958:i32)
          n485 = for {
            N: w958 -> [_]
            tunnel: w960 -> [w968]
            shift-right: [w962] -> w956
            shift-left: dbl[] [0.0] -> [w961]
            i -> [w967]
            n486 = Increment(x=w967) -> (x+1=w966:i32)
            n487 = Index Array(array=w968, index=w967) -> (element=w964:dbl)
            n488 = Index Array(array=w968, index=w966) -> (element=w965:dbl)
            n489 = Subtract(x=w965, y=w964) -> (x-y=w963:dbl)
            n490 = Build Array (concatenate)(w961, w963) -> (w962:dbl[])
          }
        }
        "Temps grads" <- w950
        n491 = call <vilib>:"Add State(s) to Queue__jki_lib_state_machine.vi"("State(s) in (\"\")"=w955) -> ("States Out"=w954:string)  [unwired: 14 in]
      }
      frame "Process: Calculate Freezing Points" {
        # "Your code here.\n(You can make a copy of, or modify, this frame)"
        n492 = local read "Temps grads"() -> (w973:dbl[][])
        n493 = local read "Temps"() -> (w971:dbl[][])
        n494 = Unbundle By Name(w978) -> ("Config.Freezing.EndIndex"=w969:i32, "Config.Freezing.Cutoff"=w977:dbl)
        n495 = local write "FreezeTemps"(dbl[] []) -> ()
        n496 = local write "FreezeIdx"(i32[] []) -> ()
        n497 = local write "FreezeArray"(bool[] []) -> ()
        n498 = Array Subset(array=w971, length (col)=w969) -> (w970:dbl[][])  [unwired: 3 in]
        n499 = Array Subset(array=w973, length (col)=w969) -> (w972:dbl[][])  [unwired: 3 in]
        n500 = for {
          tunnel: w972 -> [w990] mode=indexing
          workers-P: _ -> [_]
          tunnel: w970 -> [w999] mode=indexing
          tunnel: [w994] -> w982 mode=indexing
          tunnel: [w992] -> w981 mode=indexing
          tunnel: [w988] -> w980 mode=indexing
          tunnel: w977 -> [w987]
          # "Gradient Check"
          n501 = call <vilib>:"Std Deviation and Variance.vi"("X"=w990) -> ("standard deviation"=w989:dbl)  [unwired: 1 in, 2 out]
          n502 = Array Max & Min(array=w990) -> (max value=w997:dbl, max index (indices)=w993:i32)  [unwired: 2 out]
          n503 = Multiply(x=w987, y=w989) -> (x*y=w996:dbl)
          n504 = Array Subset(array=w999, length=w993) -> (w998:dbl[])  [unwired: 1 in]
          n505 = Greater?(x=w997, y=w996) -> (0:w995:bool)
          n506 = Array Max & Min(array=w998) -> (min value=w991:dbl, min index (indices)=w986:i32)  [unwired: 2 out]
          n507 = case shown="True" w995 {
            selector: w995 -> [w1001 w1002]
            tunnel: [w1000 w1004] -> w994
            tunnel: w986 -> [_ w1004]
            tunnel: [w1000 w1003] -> w992
            tunnel: w991 -> [_ w1003]
            tunnel: [w1001 w1002] -> w988
            frame False {
              w1000 = 0.0
            }
            frame True {
            }
          }
        }
        "FreezeIdx" <- w982
        "FreezeTemps" <- w981
        "FreezeArray" <- w980
        n508 = call <vilib>:"Add State(s) to Queue__jki_lib_state_machine.vi"("State(s) in Front (\"\")"="UI: Menu Save >> True\nUI: Menu Overlay Temps >> True" ("State(s) in Front (\"\")"), "State(s) in (\"\")"=w985) -> ("States Out"=w984:string)  [unwired: 13 in]
      }
      frame "Process: Calculate Melt Temp" {
        # "Your code here.\n(You can make a copy of, or modify, this frame)"
        n509 = local read "FreezeIdx"() -> (w1007:i32[])
        n510 = local read "Temps"() -> (w1006:dbl[][])
        n511 = for {
          tunnel: w1007 -> [w1012] mode=indexing
          workers-P: _ -> [_]
          tunnel: w1006 -> [w1017] mode=indexing
          tunnel: [w1015] -> w1005 mode=indexing
          n512 = Array Subset(array=w1017, index=w1012) -> (w1016:dbl[])  [unwired: 1 in]
          n513 = Not Equal To 0?(x=w1012) -> (x != 0?=w1013:bool)
          n514 = Array Max & Min(array=w1016) -> (max value=w1014:dbl)  [unwired: 3 out]
          n515 = case shown="False" w1013 {
            tunnel: [0.0 w1019] -> w1015
            tunnel: w1014 -> [_ w1019]
            frame False {
            }
            frame True {
            }
          }
        }
        "MeltTemps" <- w1005
        n516 = call <vilib>:"Add State(s) to Queue__jki_lib_state_machine.vi"("State(s) in (\"\")"=w1011) -> ("States Out"=w1010:string)  [unwired: 14 in]
      }
      frame "Process: Calculate Freeze Fraction" {
        # "Your code here.\n(You can make a copy of, or modify, this frame)"
        n517 = property on="FrozenFractionGraph" class="WFGraph (strict)"("Active Plot"=u32 0, "Legend Visible"=TRUE ("Legend:Visible")) -> ()  [unwired: 2 in, 2 out]
        n518 = local read "PartitionArray"() -> (w1023:string[])
        n519 = local read "FreezeTemps"() -> (w1028:dbl[])
        n520 = local read "FreezeIdx"() -> (w1026:i32[])
        n521 = local read "Temps"() -> (w1027:dbl[][])
        n522 = call "FrozenFraction_Calcualte.vi"("FreezeIdx"=w1026, "Temps"=w1027, "FreezeTemps"=w1028, "PartitionArray"=w1023) -> ("FreezeFract Concatinated"=→"FreezeFract Concatinated":dbl[], "FrozenFractionGraph"=→"FrozenFractionGraph":dbl[][])  [unwired: 6 in]
        n523 = call "WellPartition_Index.vi"("PartitionArray"=w1023) -> ("Unique Part Array"=w1022:string[])  [unwired: 1 in, 1 out]
        n524 = for {
          tunnel: w1022 -> [w1034] mode=indexing
          i -> [w1033]
          n525 = property on="FrozenFractionGraph" class="WFGraph (strict)"("Active Plot"=w1033, "Plot.Plot Name"=w1034) -> ()  [unwired: 2 in, 2 out]
        }
        n526 = call <vilib>:"Add State(s) to Queue__jki_lib_state_machine.vi"("State(s) in (\"\")"=w1032) -> ("States Out"=w1031:string)  [unwired: 14 in]
      }
      frame "Process: Calculate Offset" {
        # "Your code here.\n(You can make a copy of, or modify, this frame)"
        n527 = local read "ThermTemps"() -> (w1037:dbl[])
        n528 = local read "Path"() -> (w1035:path)
        n529 = call "TCam_FixpointTemps.vi"("input cluster"=w1038, "name or relative path"=w1035, "Therm_Temps"=w1037) -> ("Offsets"=→"Offsets":dbl[])  [unwired: 1 out]
        n530 = call <vilib>:"Add State(s) to Queue__jki_lib_state_machine.vi"("State(s) in (\"\")"=w1041) -> ("States Out"=w1040:string)  [unwired: 14 in]
      }
      frame "Process: Correct Offset" {
        # "Offset calculation\nT_Cam_Br_Corr = T_cam_Br+(T_therm_Fix - T_cam_Fix)"
        # "Your code here.\n(You can make a copy of, or modify, this frame)"
        n531 = local read "Offsets"() -> (w1045:dbl[])
        n532 = local read "Temps"() -> (w1046:dbl[][])
        n533 = for {
          tunnel: w1046 -> [w1060] mode=indexing
          tunnel: w1045 -> [w1059]
          tunnel: [w1058] -> w1044 mode=indexing
          n534 = Add(x=w1060, y=w1059) -> (x+y=w1058:dbl[])
        }
        n535 = local read "Path"() -> (w1042:path)
        n536 = case shown="True" TRUE {
          tunnel: w1044 -> [_ w1055]
          tunnel: w1042 -> [_ w1054]
          frame False {
          }
          frame True {
            # "Option to save the offset calculation temperatures"
            n537 = Build Path(base path=w1054, name or relative path=path "Temps after offset.csv") -> (appended path=w1052:path)
            n538 = call-poly <vilib>:"Write Delimited Spreadsheet.vi"("file path (dialog if empty)"=w1052, "2D data"=w1055, "append to file? (new file:F)"=FALSE, "transpose? (no:F)"=TRUE, "delimiter (\\t)"=";" ("delimiter (\\t)")) -> ()  [unwired: 9 in, 2 out]
          }
        }
        n539 = local write "Temps"(w1044) -> ()
        n540 = call <vilib>:"Add State(s) to Queue__jki_lib_state_machine.vi"("State(s) in (\"\")"=w1050) -> ("States Out"=w1049:string)  [unwired: 14 in]
      }
      frame "Process: Remove Offset" {
        # "Offset calculation\nT_Cam_Br_Corr = T_cam_Br+(T_therm_Fix - T_cam_Fix)"
        # "Your code here.\n(You can make a copy of, or modify, this frame)"
        n541 = local read "Offsets"() -> (w1062:dbl[])
        n542 = local read "Temps"() -> (w1063:dbl[][])
        n543 = for {
          tunnel: w1063 -> [w1070] mode=indexing
          tunnel: w1062 -> [w1069]
          tunnel: [w1068] -> w1061 mode=indexing
          n544 = Subtract(x=w1070, y=w1069) -> (x-y=w1068:dbl[])
        }
        n545 = local write "Temps"(w1061) -> ()
        n546 = call <vilib>:"Add State(s) to Queue__jki_lib_state_machine.vi"("State(s) in (\"\")"=w1067) -> ("States Out"=w1066:string)  [unwired: 14 in]
      }
      frame "---------- Image ----------" {
        # "Template Separator\n(You can make a copy of, or modify, this frame)"
        n547 = call <vilib>:"Add State(s) to Queue__jki_lib_state_machine.vi"("State(s) in (\"\")"=w1074) -> ("States Out"=w1073:string)  [unwired: 14 in]
      }
      frame "Image: Draw" {
        # "Template Separator\n(You can make a copy of, or modify, this frame)"
        n548 = call <vilib>:"Add State(s) to Queue__jki_lib_state_machine.vi"("State(s) in Front (\"\")"="UI: Cursor Set >> Busy\nImage: Clear ROI\nImage: Calculate BR\nImage: Calculate y space\nImage: Calculate x space\nImage: Calculate Positions\nImage: Drawlines\nImage: Draw Points\nUI: Cursor Set >> Idle" ("State(s) in Front (\"\")"), "State(s) in (\"\")"=w1079) -> ("States Out"=w1078:string)  [unwired: 13 in]
      }
      frame "Image: Redraw" {
        # "Template Separator\n(You can make a copy of, or modify, this frame)"
        n549 = call <vilib>:"Add State(s) to Queue__jki_lib_state_machine.vi"("State(s) in Front (\"\")"="UI: Cursor Set >> Busy\nImage: Clear ROI\nImage: Drawlines\nImage: Draw Points\nProcess: Calculate Temps\nUI: Cursor Set >> Idle" ("State(s) in Front (\"\")"), "State(s) in (\"\")"=w1084) -> ("States Out"=w1083:string)  [unwired: 13 in]
      }
      frame "Image: Set Cursors" {
        w1088 = -45.0 ("X Scale.Range:Minimum")
        w1089 = 40.0 ("Y Scale.Range:Maximum")
        w1085 = 0 ("lower limit")
        # "Template Separator\n(You can make a copy of, or modify, this frame)"
        n550 = local read "ImageIdx"() -> (w1087:u32)
        n551 = local read "maxSize"() -> (w1086:i32)
        n552 = property on="Temps grads" class="WFGraph (strict)"("Cursor.Cursor X"=w1087, "XScale.Maximum"=w1086, "XScale.Minimum"=w1085) -> ()  [unwired: 2 in, 2 out]
        n553 = property on="Temps single" class="WFGraph (strict)"("Cursor.Cursor X"=w1087, "XScale.Maximum"=w1086, "XScale.Minimum"=w1085, "YScale.Maximum"=w1089, "YScale.Minimum"=w1088) -> ()  [unwired: 2 in, 2 out]
        n554 = property on="Temps" class="WFGraph (strict)"("Cursor.Cursor X"=w1087, "XScale.Maximum"=w1086, "XScale.Minimum"=w1085, "YScale.Maximum"=w1089, "YScale.Minimum"=w1088) -> ()  [unwired: 2 in, 2 out]
        n555 = property on="FrozenFractionGraph" class="WFGraph (strict)"("Cursor.Cursor X"=w1087, "XScale.Maximum"=w1086, "XScale.Minimum"=w1085) -> ()  [unwired: 2 in, 2 out]
        n556 = property on="Fraction Single" class="WFGraph (strict)"("Cursor.Cursor X"=w1087, "XScale.Maximum"=w1086, "XScale.Minimum"=w1085) -> ()  [unwired: 2 in, 2 out]
        n557 = property on="Temps single grad" class="WFGraph (strict)"("Cursor.Cursor X"=w1087, "XScale.Maximum"=w1086, "XScale.Minimum"=w1085) -> ()  [unwired: 2 in, 2 out]
        n558 = property on="Temps" class="WFGraph (strict)"("Cursor.Cursor X"=w1087, "XScale.Maximum"=w1086, "XScale.Minimum"=w1085) -> ()  [unwired: 2 in, 2 out]
        n559 = call <vilib>:"Add State(s) to Queue__jki_lib_state_machine.vi"("State(s) in (\"\")"=w1093) -> ("States Out"=w1092:string)  [unwired: 14 in]
      }
      frame "Image: Drawlines" {
        # "Template Separator\n(You can make a copy of, or modify, this frame)"
        n560 = Unbundle By Name(w1094) -> ("Points.Top Left.X"=w1110:sgl, "Points.Top Right.X"=w1109:sgl, "Points.Bottom Left.X"=w1108:sgl, "Points.Bottom Right.X"=w1107:sgl)
        n561 = Equal To 0?(x=w1110) -> (x = 0?=w1106:bool)
        n562 = Equal To 0?(x=w1109) -> (x = 0?=w1105:bool)
        n563 = Equal To 0?(x=w1108) -> (x = 0?=w1096:bool)
        n564 = Equal To 0?(x=w1107) -> (x = 0?=w1097:bool)
        n565 = Or(x=w1096, y=w1097) -> (x .or. y?=w1095:bool)
        n566 = Select(t="", s=w1096, f="Image: Draw Line >> TL_BL\n") -> (s? t:f=w1102:string)
        n567 = Select(t="", s=w1095, f="Image: Draw Line >> TR_BR\nImage: Draw Line >> BL_BR\nImage: Draw Line >> Vertical\nImage: Draw Line >> Horizontal") -> (s? t:f=w1099:string)
        n568 = case shown="False" w1106 {
          tunnel: w1105 -> [w1117 _]
          tunnel: w1102 -> [w1116 _]
          tunnel: w1099 -> [w1115 _]
          tunnel: [w1114 _] -> w1098
          frame False {
            n569 = case shown="False" w1117 {
              tunnel: w1116 -> [w1120 _]
              tunnel: w1115 -> [w1119 _]
              tunnel: [w1118 _] -> w1114
              frame False {
                n570 = Concatenate Strings("Image: Draw Line >> TL_TR\n", w1120, w1119) -> (w1118:string)
              }
              frame True {
              }
            }
          }
          frame True {
          }
        }
        n571 = call <vilib>:"Add State(s) to Queue__jki_lib_state_machine.vi"("State(s) in Front (\"\")"=w1098, "State(s) in (\"\")"=w1113) -> ("States Out"=w1112:string)  [unwired: 13 in]
      }
      frame "Image: Draw Line" {
        w1122 = u32 2  # Width
        # "Your code here.\n(You can make a copy of, or modify, this frame)"
        n572 = Unbundle By Name(w1126) -> ("Image Out"=w1127:T1)
        n573 = case shown="\"Vertical\"" w1128 {
          tunnel: w1127 -> [w1132 w1140 w1149 w1156 w1162 w1167 w1176]
          tunnel: w1126 -> [_ w1141 w1150 w1151 w1157 w1171 w1180]
          tunnel: [w1132 w1135 w1148 w1155 w1161 w1163 w1172] -> w1125
          tunnel: w1124 -> [w1131 w1139 w1147 w1154 w1160 w1165 w1175]
          tunnel: [w1131 w1134 w1146 w1153 w1159 w1164 w1174] -> w1123
          tunnel: w1122 -> [_ w1133 w1142 _ _ w1166 w1173]
          frame "False", Default {
          }
          frame "TL_TR" {
            n574 = Unbundle By Name(w1141) -> ("Points.Top Left"=w1138:T2, "Points.Top Right"=w1137:T2)
            n575 = Build Array(w1138, w1137) -> (w1136:T2[])
            n576 = call "IMAQ Overlay Multiple Lines 2"("Image"=w1140, "Line End Points"=w1136, "error in (no error)"=w1139, "Width"=w1133) -> ("Image Out"=w1135:T1, "error out"=w1134:errorcluster)  [unwired: 10 in]
          }
          frame "TL_BL" {
            n577 = Unbundle By Name(w1150) -> ("Points.Top Left"=w1145:T2, "Points.Bottom Left"=w1144:T2)
            n578 = Build Array(w1145, w1144) -> (w1143:T2[])
            n579 = call "IMAQ Overlay Multiple Lines 2"("Image"=w1149, "Line End Points"=w1143, "error in (no error)"=w1147, "Width"=w1142) -> ("Image Out"=w1148:T1, "error out"=w1146:errorcluster)  [unwired: 10 in]
          }
          frame "Vertical" {
            n580 = call "TCam_VerticalLines.vi"("Width"=u32 1, "error in (no error)"=w1154, "Cluster"=w1151, "Refnum in"=w1156) -> ("error out"=w1153:errorcluster, "Refnum out"=w1155:T1)  [unwired: 6 in]
          }
          frame "Horizontal" {
            n581 = call "TCam_HorizontalLines.vi"("Width"=u32 1, "error in (no error)"=w1160, "Cluster"=w1157, "Refnum in"=w1162) -> ("error out"=w1159:errorcluster, "Refnum out"=w1161:T1)  [unwired: 6 in]
          }
          frame "TR_BR" {
            n582 = Unbundle By Name(w1171) -> ("Points.Top Right"=w1170:T2, "Points.Bottom Right"=w1169:T2)
            n583 = Build Array(w1170, w1169) -> (w1168:T2[])
            n584 = call "IMAQ Overlay Multiple Lines 2"("Image"=w1167, "Line End Points"=w1168, "error in (no error)"=w1165, "Width"=w1166) -> ("Image Out"=w1163:T1, "error out"=w1164:errorcluster)  [unwired: 10 in]
          }
          frame "BL_BR" {
            n585 = Unbundle By Name(w1180) -> ("Points.Bottom Left"=w1179:T2, "Points.Bottom Right"=w1178:T2)
            n586 = Build Array(w1179, w1178) -> (w1177:T2[])
            n587 = call "IMAQ Overlay Multiple Lines 2"("Image"=w1176, "Line End Points"=w1177, "error in (no error)"=w1175, "Width"=w1173) -> ("Image Out"=w1172:T1, "error out"=w1174:errorcluster)  [unwired: 10 in]
          }
        }
        n588 = local write "Image"(w1125) -> ()
        n589 = call <vilib>:"Add State(s) to Queue__jki_lib_state_machine.vi"("State(s) in (\"\")"=w1130) -> ("States Out"=w1129:string)  [unwired: 14 in]
      }
      frame "Image: Draw Points" {
        # "Your code here.\n(You can make a copy of, or modify, this frame)"
        n590 = Unbundle By Name(w1183) -> ("Points.Top Left.X"=w1192:sgl, "Points.Top Right.X"=w1191:sgl, "Points.Bottom Left.X"=w1190:sgl, "Points.Bottom Right.X"=w1189:sgl)
        n591 = Equal To 0?(x=w1192) -> (x = 0?=w1188:bool)
        n592 = Equal To 0?(x=w1191) -> (x = 0?=w1187:bool)
        n593 = Equal To 0?(x=w1190) -> (x = 0?=w1186:bool)
        n594 = Equal To 0?(x=w1189) -> (x = 0?=w1185:bool)
        n595 = Unbundle By Name(w1183) -> ("Image Out"=w1194:T1, "Scan Area"=w1181:dbl)
        n596 = Compound Arithmetic op=OR(w1188, w1187, w1186, w1185) -> (w1184:bool)
        n597 = case shown="False" w1184 {
          tunnel: w1194 -> [w1203 _]
          tunnel: w1183 -> [w1200 w1204]
          tunnel: [w1198 w1204] -> w1182
          tunnel: w1181 -> [w1197 _]
          frame False {
            n598 = local read "Points"() -> (w1202:T2[])
            n599 = call "TCam_CenterArray.vi"("Image in"=w1203, "Point Array"=w1202, "Size"=w1197) -> ("Image"=w1201:T1, "Array"=w1199:cluster{"X":i32, "Y":i32}[][])  [unwired: 3 in, 1 out]
            n600 = local write "Image"(w1201) -> ()
            n601 = Bundle By Name(cluster=w1200, "Points.Pixels"=w1199) -> (w1198:T4)
          }
          frame True {
          }
        }
        n602 = call <vilib>:"Add State(s) to Queue__jki_lib_state_machine.vi"("State(s) in (\"\")"=w1196) -> ("States Out"=w1195:string)  [unwired: 14 in]
      }
      frame "Image: Calculate x space" {
        # "Your code here.\n(You can make a copy of, or modify, this frame)"
        n603 = Unbundle By Name(w1213) -> ("Points.Top Left"=w1219:T2, "Points.Top Right"=w1218:T2, "PCR Size"=w1205:u16)
        n604 = case shown="0, Default" w1205 {
          tunnel: [24 12] -> w1206
          frame 0, Default {
          }
          frame 1 {
          }
        }
        n605 = Unbundle(w1219) -> ("X"=w1216:sgl, "Y"=w1214:sgl)
        n606 = Unbundle(w1218) -> ("X"=w1217:sgl, "Y"=w1215:sgl)
        n607 = Subtract(x=w1217, y=w1216) -> (x-y=w1210:sgl)
        n608 = Subtract(x=w1215, y=w1214) -> (x-y=w1208:sgl)
        n609 = Decrement(x=w1206) -> (x-1=w1209:i32)
        n610 = Divide(x=w1210, y=w1209) -> (x/y=w1211:sgl)
        n611 = Divide(x=w1208, y=w1209) -> (x/y=w1207:sgl)
        n612 = Bundle By Name(cluster=w1213, "Points.x_space"=w1211, "Points.y_space"=w1207) -> (w1212:T4)
        n613 = call <vilib>:"Add State(s) to Queue__jki_lib_state_machine.vi"("State(s) in (\"\")"=w1222) -> ("States Out"=w1221:string)  [unwired: 14 in]
      }
      frame "Image: Calculate BR" {
        # "Your code here.\n(You can make a copy of, or modify, this frame)"
        n614 = Unbundle By Name(w1233) -> ("Points.Top Left"=w1239:T2, "Points.Top Right"=w1238:T2, "Points.Bottom Left"=w1231:T2)
        n615 = Unbundle(w1239) -> ("X"=w1236:sgl, "Y"=w1234:sgl)
        n616 = Unbundle(w1231) -> ("X"=w1230:sgl, "Y"=w1228:sgl)
        n617 = Unbundle(w1238) -> ("X"=w1237:sgl, "Y"=w1235:sgl)
        n618 = Subtract(x=w1237, y=w1236) -> (x-y=w1229:sgl)
        n619 = Add(x=w1230, y=w1229) -> (x+y=w1225:sgl)
        n620 = Subtract(x=w1235, y=w1234) -> (x-y=w1227:sgl)
        n621 = Add(x=w1227, y=w1228) -> (x+y=w1226:sgl)
        n622 = Bundle By Name(cluster=w1233, "Points.Bottom Right.X"=w1225, "Points.Bottom Right.Y"=w1226) -> (w1232:T4)
        n623 = call <vilib>:"Add State(s) to Queue__jki_lib_state_machine.vi"("State(s) in (\"\")"=w1242) -> ("States Out"=w1241:string)  [unwired: 14 in]
      }
      frame "Image: Calculate y space" {
        # "Your code here.\n(You can make a copy of, or modify, this frame)"
        n624 = Unbundle By Name(w1251) -> ("Points.Top Left"=w1257:T2, "Points.Bottom Left"=w1256:T2, "PCR Size"=w1243:u16)
        n625 = case shown="1" w1243 {
          tunnel: [16 8] -> w1244
          frame 0, Default {
          }
          frame 1 {
          }
        }
        n626 = Unbundle(w1257) -> ("X"=w1254:sgl, "Y"=w1252:sgl)
        n627 = Unbundle(w1256) -> ("X"=w1255:sgl, "Y"=w1253:sgl)
        n628 = Subtract(x=w1255, y=w1254) -> (x-y=w1248:sgl)
        n629 = Subtract(x=w1253, y=w1252) -> (x-y=w1246:sgl)
        n630 = Decrement(x=w1244) -> (x-1=w1247:i32)
        n631 = Divide(x=w1248, y=w1247) -> (x/y=w1249:sgl)
        n632 = Divide(x=w1246, y=w1247) -> (x/y=w1245:sgl)
        n633 = Bundle By Name(cluster=w1251, "Points.x space 2"=w1249, "Points.y space 2"=w1245) -> (w1250:T4)
        n634 = call <vilib>:"Add State(s) to Queue__jki_lib_state_machine.vi"("State(s) in (\"\")"=w1260) -> ("States Out"=w1259:string)  [unwired: 14 in]
      }
      frame "Image: Calculate Positions" {
        # "Your code here.\n(You can make a copy of, or modify, this frame)"
        n635 = Unbundle By Name(w1265) -> ("Scan Area"=w1263:dbl, "Points.Top Left.X"=w1273:sgl, "Points.Top Right.X"=w1272:sgl, "Points.Bottom Left.X"=w1271:sgl, "Points.Bottom Right.X"=w1270:sgl)
        n636 = Equal To 0?(x=w1273) -> (x = 0?=w1269:bool)
        n637 = Equal To 0?(x=w1272) -> (x = 0?=w1268:bool)
        n638 = Equal To 0?(x=w1271) -> (x = 0?=w1267:bool)
        n639 = Equal To 0?(x=w1270) -> (x = 0?=w1266:bool)
        n640 = Compound Arithmetic op=OR(w1269, w1268, w1267, w1266) -> (w1264:bool)
        n641 = case shown="False" w1264 {
          tunnel: w1265 -> [w1278 _]
          tunnel: w1263 -> [w1277 _]
          frame False {
            n642 = call "TCam_PointCalculator.vi"("Cluster"=w1278, "Size"=w1277) -> ("Points"=→"Points":T2[])  [unwired: 9 in]
          }
          frame True {
          }
        }
        n643 = call <vilib>:"Add State(s) to Queue__jki_lib_state_machine.vi"("State(s) in (\"\")"=w1276) -> ("States Out"=w1275:string)  [unwired: 14 in]
      }
      frame "Image: Clear ROI" {
        # "Your code here.\n(You can make a copy of, or modify, this frame)"
        n644 = Unbundle By Name(w1283) -> ("Image Out"=w1282:T1)
        n645 = call "IMAQ Clear Overlay"("error in (no error)"=w1281, "Image"=w1282) -> ("error out"=w1280:errorcluster)  [unwired: 8 in, 1 out]
        n646 = call <vilib>:"Add State(s) to Queue__jki_lib_state_machine.vi"("State(s) in (\"\")"=w1285) -> ("States Out"=w1284:string)  [unwired: 14 in]
      }
      frame "Image: Set ROI" {
        # "Your code here.\n(You can make a copy of, or modify, this frame)"
        n647 = Unbundle By Name(w1289) -> ("State"=w1291:i32)
        n648 = case shown="0, Default" w1291 {
          tunnel: [w1295 w1298 w1300 w1302] -> w1290
          tunnel: w1289 -> [w1296 w1297 w1299 w1301]
          frame 0, Default {
            n649 = Unbundle By Name(w1296) -> ("Points.Top Left"=w1295:T2)
          }
          frame 1 {
            n650 = Unbundle By Name(w1297) -> ("Points.Top Right"=w1298:T2)
          }
          frame 2 {
            n651 = Unbundle By Name(w1299) -> ("Points.Bottom Left"=w1300:T2)
          }
          frame 3 {
            n652 = Unbundle By Name(w1301) -> ("Points.Bottom Right"=w1302:T2)
          }
        }
        n653 = call "IMAQ Convert Point to ROI"("error in (no error)"=w1288, "Point"=w1290) -> ("error out"=w1287:errorcluster, "ROI Descriptor"=w1292:T11)  [unwired: 7 in]
        n654 = property on="Image" class="ImageControl"(error in=w1287, "ROI"=w1292) -> (error out=w1286:errorcluster)  [unwired: 1 in, 1 out]
        n655 = call <vilib>:"Add State(s) to Queue__jki_lib_state_machine.vi"("State(s) in (\"\")"=w1294) -> ("States Out"=w1293:string)  [unwired: 14 in]
      }
      frame "---------- Overlay ----------" {
        # "Template Separator\n(You can make a copy of, or modify, this frame)"
        n656 = call <vilib>:"Add State(s) to Queue__jki_lib_state_machine.vi"("State(s) in (\"\")"=w1306) -> ("States Out"=w1305:string)  [unwired: 14 in]
      }
      frame "Overlay: Overlay Freeze" {
        # "Your code here.\n(You can make a copy of, or modify, this frame)"
        n657 = local read "FreezeArray"() -> (w1308:bool[])
        n658 = local read "FreezeIdx"() -> (w1309:i32[])
        n659 = local read "Points"() -> (w1310:T2[])
        n660 = Unbundle By Name(w1312) -> ("img_array"=w1311:T1[])
        n661 = call "OverlayFreezeRange.vi"("FreezeIdx"=w1309, "FreezeArray"=w1308) -> ("Range"=w1307:i32)
        n662 = for {
          N -> [w1318]
          tunnel: w1309 -> [w1330] mode=indexing
          tunnel: w1311 -> [w1331]
          tunnel: w1310 -> [w1329] mode=indexing
          tunnel: w1308 -> [w1328] mode=indexing
          tunnel: w1307 -> [w1327]
          n663 = local read "img"() -> (w1319:i32)
          n664 = case shown="True" w1328 {
            tunnel: w1331 -> [_ w1339]
            tunnel: w1330 -> [_ w1332]
            tunnel: w1329 -> [_ w1337]
            tunnel: w1327 -> [_ w1334]
            frame False {
            }
            frame True {
              n665 = Divide(x=w1332, y=w1334) -> (x/y=w1336:dbl)
              n666 = Array Subset(array=w1339, index=w1332) -> (w1338:T1[])  [unwired: 1 in]
              n667 = Multiply(x=w1336, y=30.0) -> (x*y=w1333:dbl)
              n668 = for {
                tunnel: w1338 -> [w1345] mode=indexing
                tunnel: w1337 -> [w1344]
                workers-P: _ -> [_]
                tunnel: w1333 -> [w1343]
                n669 = call "ColorRamp.vi"("Slide"=w1343) -> ("Color"=w1342:u32)
                n670 = call "IMAQ Overlay Text"("BG Color (Transparent)"=w1342, "Font, Size & Style"=T10 {"Desired Font (Application)"=enum."Application Font", "[User-specified Font]"={"Font Name"="", "Size"=1, "Strikeout?"=FALSE, "Italic?"=FALSE, "Underline?"=FALSE, "Outline?"=FALSE, "Shadow?"=FALSE, "Bold?"=FALSE, "Rotation Angle"=0.0}, "Horizontal Alignment"=1, "Vertical Alignment"=0}, "String"="   ", "Origin"=w1344, "Image"=w1345) -> ()  [unwired: 5 in, 2 out]
              }
            }
          }
          n671 = Increment(x=w1319) -> (x+1=w1326:i32)
          n672 = Divide(x=w1319, y=w1318) -> (x/y=w1325:dbl)
          n673 = local write "img"(w1326) -> ()
          n674 = Multiply(x=w1325, y=100.0) -> (x*y=w1324:dbl)
          n675 = local write "Slide"(w1324) -> ()
          n676 = Format Into String(initial string="Overlaying Well " ("Tutorial"), w1319) -> (resulting string=w1321:string)  [unwired: 2 in, 1 out]
          n677 = Format Into String(initial string=" of ", w1318) -> (resulting string=w1322:string)  [unwired: 2 in, 1 out]
          n678 = Concatenate Strings(w1321, w1322) -> (w1320:string)
          n679 = local write "Tutorial"(w1320) -> ()
        }
        n680 = call <vilib>:"Add State(s) to Queue__jki_lib_state_machine.vi"("State(s) in (\"\")"=w1315) -> ("States Out"=w1314:string)  [unwired: 14 in]
      }
      frame "Overlay: Overlay Freeze Temps" {
        # "Your code here.\n(You can make a copy of, or modify, this frame)"
        n681 = local read "FreezeTemps"() -> (w1349:dbl[])
        n682 = local read "FreezeArray"() -> (w1347:bool[])
        n683 = local read "FreezeIdx"() -> (w1348:i32[])
        n684 = local read "Points"() -> (w1350:T2[])
        n685 = Unbundle By Name(w1352) -> ("img_array"=w1351:T1[])
        n686 = call "OverlayFreezeRange.vi"("FreezeIdx"=w1348, "FreezeArray"=w1347) -> ("Range"=w1346:i32)
        n687 = for {
          N -> [w1356]
          tunnel: w1348 -> [w1371] mode=indexing
          tunnel: w1351 -> [w1372]
          tunnel: w1350 -> [w1370] mode=indexing
          tunnel: w1349 -> [w1369] mode=indexing
          tunnel: w1347 -> [w1368] mode=indexing
          tunnel: w1346 -> [w1367]
          n688 = local read "img"() -> (w1366:i32)
          n689 = case shown="True" w1368 {
            tunnel: w1372 -> [_ w1381]
            tunnel: w1371 -> [_ w1373]
            tunnel: w1370 -> [_ w1379]
            tunnel: w1369 -> [_ w1376]
            tunnel: w1367 -> [_ w1375]
            frame False {
            }
            frame True {
              n690 = Divide(x=w1373, y=w1375) -> (x/y=w1378:dbl)
              n691 = Array Subset(array=w1381, index=w1373) -> (w1380:T1[])  [unwired: 1 in]
              n692 = Multiply(x=w1378, y=30.0) -> (x*y=w1374:dbl)
              n693 = for {
                tunnel: w1380 -> [w1386] mode=indexing
                tunnel: w1379 -> [w1385]
                tunnel: w1376 -> [w1384]
                workers-P: _ -> [_]
                tunnel: w1374 -> [w1383]
                n694 = call "ColorRamp.vi"("Slide"=w1383) -> ("Color"=w1382:u32)
                n695 = Format Into String(format string="%3.2f", w1384) -> (resulting string=w1389:string)  [unwired: 2 in, 1 out]
                n696 = call "IMAQ Overlay Text"("BG Color (Transparent)"=w1382, "Font, Size & Style"=T10 {"Desired Font (Application)"=enum."Application Font", "[User-specified Font]"={"Font Name"="", "Size"=6, "Strikeout?"=FALSE, "Italic?"=FALSE, "Underline?"=FALSE, "Outline?"=FALSE, "Shadow?"=FALSE, "Bold?"=FALSE, "Rotation Angle"=0.0}, "Horizontal Alignment"=1, "Vertical Alignment"=0}, "String"=w1389, "Origin"=w1385, "Image"=w1386) -> ()  [unwired: 5 in, 2 out]
              }
            }
          }
          n697 = Increment(x=w1366) -> (x+1=w1360:i32)
          n698 = Divide(x=w1366, y=w1356) -> (x/y=w1361:dbl)
          n699 = local write "img"(w1360) -> ()
          n700 = Multiply(x=w1361, y=100.0) -> (x*y=w1362:dbl)
          n701 = local write "Slide"(w1362) -> ()
          n702 = Format Into String(initial string="Overlaying Well " ("Tutorial"), w1366) -> (resulting string=w1364:string)  [unwired: 2 in, 1 out]
          n703 = Format Into String(initial string=" of ", w1356) -> (resulting string=w1363:string)  [unwired: 2 in, 1 out]
          n704 = Concatenate Strings(w1364, w1363) -> (w1365:string)
          n705 = local write "Tutorial"(w1365) -> ()
        }
        n706 = call <vilib>:"Add State(s) to Queue__jki_lib_state_machine.vi"("State(s) in (\"\")"=w1355) -> ("States Out"=w1354:string)  [unwired: 14 in]
      }
      frame "Overlay: Overlay Freeze Old" {
        # "Your code here.\n(You can make a copy of, or modify, this frame)"
        n707 = local read "FreezeArray"() -> (w1391:bool[])
        n708 = Unbundle By Name(w1394) -> ("img_array"=w1396:T1[])
        n709 = local read "FreezeIdx"() -> (w1392:i32[])
        n710 = Unbundle By Name(w1394) -> ("Points.Pixels"=w1393:cluster{"X":i32, "Y":i32}[][])
        n711 = local read "Points"() -> (w1395:T2[])
        n712 = call "OverlayFreezeRange.vi"("FreezeIdx"=w1392, "FreezeArray"=w1391) -> ("Range"=w1390:i32)
        n713 = for {
          N -> [w1402]
          tunnel: w1392 -> [w1417] mode=indexing
          tunnel: w1396 -> [w1420]
          tunnel: w1395 -> [w1418] mode=indexing
          workers-P: _ -> [_]
          tunnel: w1390 -> [w1415]
          tunnel: w1393 -> [w1414] mode=indexing
          tunnel: w1391 -> [w1400] mode=indexing
          n714 = local read "img"() -> (w1403:i32)
          n715 = Increment(x=w1403) -> (x+1=w1408:i32)
          n716 = Divide(x=w1417, y=w1415) -> (x/y=w1416:dbl)
          n717 = Array Subset(array=w1420, index=w1417) -> (w1419:T1[])  [unwired: 1 in]
          n718 = local write "img"(w1408) -> ()
          n719 = Multiply(x=w1416, y=30.0) -> (x*y=w1413:dbl)
          n720 = Divide(x=w1403, y=w1402) -> (x/y=w1411:dbl)
          n721 = case shown="True" w1400 {
            tunnel: w1419 -> [_ w1424]
            tunnel: w1418 -> [_ w1423]
            tunnel: w1414 -> [_ w1422]
            tunnel: w1413 -> [_ w1421]
            frame False {
            }
            frame True {
              n722 = for {
                tunnel: w1424 -> [w1425] mode=indexing
                tunnel: w1423 -> [w1429]
                tunnel: w1421 -> [w1427]
                tunnel: w1422 -> [w1428]
                n723 = call "ColorRamp.vi"("Slide"=w1427) -> ("Color"=w1426:u32)
                n724 = call "IMAQ Overlay Points"("Color"=w1426, "Array of Points"=w1428, "Point"=w1429, "Image"=w1425) -> ()  [unwired: 6 in, 2 out]
              }
            }
          }
          n725 = Multiply(x=w1411, y=100.0) -> (x*y=w1410:dbl)
          n726 = local write "Slide"(w1410) -> ()
          n727 = Format Into String(w1403) -> (resulting string=w1406:string)  [unwired: 3 in, 1 out]
          n728 = Format Into String(w1402) -> (resulting string=w1407:string)  [unwired: 3 in, 1 out]
          n729 = Concatenate Strings("Overlaying Well " ("Tutorial"), w1406, " of " ("Tutorial"), w1407) -> (w1405:string)
          n730 = local write "Tutorial"(w1405) -> ()
        }
        n731 = call <vilib>:"Add State(s) to Queue__jki_lib_state_machine.vi"("State(s) in (\"\")"=w1399) -> ("States Out"=w1398:string)  [unwired: 14 in]
      }
      frame "Overlay: Remove Overlays" {
        # "Your code here.\n(You can make a copy of, or modify, this frame)"
        n732 = Unbundle By Name(w1431) -> ("img_array"=w1430:T1[])
        n733 = for {
          tunnel: w1430 -> [w1435] mode=indexing
          n734 = call "IMAQ Clear Overlay"("Image"=w1435) -> ()  [unwired: 9 in, 2 out]
        }
        n735 = call <vilib>:"Add State(s) to Queue__jki_lib_state_machine.vi"("State(s) in (\"\")"=w1434) -> ("States Out"=w1433:string)  [unwired: 14 in]
      }
      frame "Overlay: Update Focus Well" {
        # "Your code here.\n(You can make a copy of, or modify, this frame)"
        n736 = local read "FrozenFractionGraph"() -> (w1437:dbl[][])
        n737 = local read "FreezeIdx"() -> (w1439:i32[])
        n738 = local read "Temps"() -> (w1447:dbl[][])
        n739 = local read "PartitionArray"() -> (w1442:string[])
        n740 = local read "Temps grads"() -> (w1446:dbl[][])
        n741 = local read "MeltTemps"() -> (w1438:dbl[])
        n742 = call "PCRNameArray.vi"("input cluster"=w1441) -> ("WellArray"=w1440:string[])
        n743 = local read "FreezeTemps"() -> (w1445:dbl[])
        n744 = local read "Well"() -> (w1443:i32)
        n745 = Empty Array?(array=w1447) -> (empty?=w1444:bool)
        n746 = case shown="False" w1444 {
          tunnel: w1443 -> [w1453 _]
          tunnel: w1447 -> [w1469 _]
          tunnel: w1446 -> [w1468 _]
          tunnel: w1445 -> [w1467 _]
          tunnel: w1442 -> [w1452 _]
          tunnel: w1440 -> [w1464 _]
          tunnel: w1439 -> [w1460 _]
          tunnel: w1438 -> [w1459 _]
          tunnel: w1437 -> [w1457 _]
          frame False {
            n747 = call "WellPartition_Index.vi"("PartitionArray"=w1452, "Well"=w1453) -> ("Partition Index"=w1454:i32)  [unwired: 1 out]
            n748 = Index Array(array=w1459, index=w1453) -> (element=→"MeltTemp":dbl)
            n749 = Index Array(array=w1469, index (row)=w1453) -> (element=w1462:dbl[])  [unwired: 1 in]
            n750 = Index Array(array=w1467, index=w1453) -> (element=→"FreezeTemp":dbl)
            n751 = Index Array(array=w1468, index (row)=w1453) -> (element=→"Temps single grad":dbl[])  [unwired: 1 in]
            n752 = Index Array(array=w1452, index=w1453) -> (element=w1451:string)
            "Contents" <- w1451
            n753 = Index Array(array=w1464, index=w1453) -> (element=→"Well":string)
            n754 = Index Array(array=w1460, index=w1453) -> (element=w1455:i32)
            n755 = Index Array(array=w1457, index (row)=w1454) -> (element=→"Fraction Single":dbl[])  [unwired: 1 in]
            n756 = Index Array(array=w1462, index=w1455) -> (element=→"CurTemp":dbl)
            n757 = local write "ImageIdx"(w1455) -> ()
            n758 = local write "Temps single"(w1462) -> ()
            n759 = property on="Fraction Single" class="WFGraph (strict)"("Plot.Plot Name"=w1451) -> ()  [unwired: 2 in, 2 out]
          }
          frame True {
          }
        }
        n760 = call <vilib>:"Add State(s) to Queue__jki_lib_state_machine.vi"("State(s) in Front (\"\")"="Image: Set Cursors" ("State(s) in Front (\"\")"), "State(s) in (\"\")"=w1450) -> ("States Out"=w1449:string)  [unwired: 13 in]
      }
    }
  }
